vi "Interface.vi"() -> ()   [LabVIEW 2012]
uses:
  MeasureModeControl.ctl
  <vilib>/Utility/miscctls.llb/LVBoundsTypeDef.ctl
  GlobalVariables/LanguagesSettings.vi
  GlobalVariables/CaptParameters.vi
  GlobalVariables/MachineInfos.vi
  GlobalVariables/StabilizationSettings.vi
  GlobalVariables/CalibrationVolumes.vi
  GlobalVariables/HardwarePresent.vi
  GlobalVariables/AppState.vi
  GlobalVariables/PressureAndTimeSamples.vi
  GlobalVariables/CurrentPressure.vi
  GlobalVariables/CommunicationActivity.vi
  GlobalVariables/CalibrationState.vi
  GlobalVariables/FittedCurvePolynom.vi
  <vilib>/Utility/file.llb/Write To Spreadsheet File (string).vi
  <vilib>/Utility/file.llb/Read From Spreadsheet File (string).vi
  GlobalVariables/MeasureExportStrings.vi
  <vilib>/Utility/config.llb/Read Key (String).vi
  GlobalVariables/UserInfos.vi
  <vilib>/Utility/config.llb/NI_LVConfig.lvlib
panel:
  in  "DeleteMeasureLine":bool
  in  "ExportData":bool
  in  "LoadData":bool
  in  "SaveData":bool
  in  "ReloadResultTableTexts":bool
  in  "MeasureMode":T1
  in  "ReloadDiskVolumes":bool
  in  "StabilityAchieved":bool
  in  "UpdateServiceGraph":bool
  in  "ComputeCalibrationResult":bool
  in  "SingleCalibrationMeasureButtonsVisible":bool
  out "FirstGraphSampleIndex":i32
  in  "ServiceButtonsVisible":bool
  in  "ExportMeasuresButtonsVisible":bool
  in  "ChangeMenuState":bool
  in  "MeasureIndicatorsVisible":bool
  in  "MeasureSetupButtonsVisible":bool
  in  "CalibrationButtonsVisible":bool
  in  "CalibrationResultsVisible":bool
  in  "UserFilledDataChanged":bool
  out "NotificationTexts":string[](array[string])
  out "rPressionM":dbl caption="Pression courante" format="%#.1f bars"
  out "error out":errorcluster caption="sortie d'erreur"
  out "indicateurPerteSignal":bool caption="Perte du signal de pression"
  out "indicateurDefautPuissance":bool caption="Défaut de puissance"
  out "indicateurSurpression":bool caption="Surpression"
  in  "btnExit":bool
  out "vTimeDate":timestamp format="%<%.1X\n%x>T"
  out "strInstallName":string="INSTALL NAME"
  in  "AppTab":T2(tab) caption="Onglets1"
  out "presentationPicture":picture caption="Please wait …"
  in  "MeasuresTabs":enum32{"Grain measures", "Pore measures"}(tab) caption="Measures"
  in  "LoadGrainMeasuresBtn":bool
  in  "SaveGrainMeasuresBtn":bool caption="SaveDataFileButton"
  in  "ExportGrainMeasuresBtn":bool caption="Exporter"
  in  "ClearGrainMeasuresBtn":bool caption="Clear measures table"
  out "grainMeasuresTable":string[][](table)=[["Date", "Numéro", "ID de l'échantillon", "Profondeur (coudées)", "Poids à sec (g)", "Volume de grain (cm3)", "Densité de grain (g/cm3)", "Volume de pore (cm3)", "Porosité (%)", "Volume de l'enveloppe (cm3)", "Longueur (cm)", "Diamètre (cm)", "Epaisseur (cm)", "Température (°C)", "Commentaires"]] caption="Résultats Mesures de grains"
  in  "ClearGrainMeasureBtn":bool
  in  "LoadPoreMeasuresBtn":bool
  in  "SavePoreMeasuresBtn":bool caption="SaveDataFileButton"
  in  "ExportPoreMeasuresBtn":bool caption="Exporter"
  out "poreMeasuresTable":string[][](table)=[["Date", "Numéro", "ID de l'échantillon", "Profondeur (coudées)", "Poids à sec (g)", "Volume de grain (cm3)", "Densité de grain (g/cm3)", "Volume de pore (cm3)", "Porosité (%)", "Volume de l'enveloppe (cm3)", "Longueur (cm)", "Diamètre (cm)", "Epaisseur (cm)", "Température (°C)", "Commentaires"]] caption="Résultats"
  in  "ClearPoreMeasuresBtn":bool caption="Clear measures table"
  in  "ClearPoreMeasureBtn":bool
  in  "btnMesureGrain":bool
  out "MeasureTotalAddedVolume":dbl caption="Volume total"
  in  "MeasureDiskSet":i32(listbox) caption="Jeu de disques"
  in  "MeasureDiskVolumes":i32[](listbox) caption="Volumes disponibles"
  in  "Comments":string caption="Commentaires"
  in  "Temperature":dbl caption="Température (°C)"
  in  "BulkVolume":dbl caption="Volume de grain (cm3)"
  in  "DryWeight":dbl caption="Poids à sec (g)"
  in  "SampleDepth":dbl caption="Profondeur (cm)"
  in  "SampleID":string caption="ID de l'échantillon"
  in  "SampleNumber":string caption="Numéro"
  in  "DoMeasureMeasure":bool caption="LaunchMeasureMeasure"
  in  "ReferenceCellMeasure":u16=1 caption="Cellule de référence" min=1 max=2
  in  "DiskSet":i32(listbox) caption="Jeu de disques"
  in  "RestartCalibration":bool
  out "CalibrationStep":u32 caption="Nombre de mesures effectuées"
  in  "CalibrationFilePath":path caption="Fichier de calibration"
  in  "LoadCalibrationFileBtn":bool
  in  "ReferenceCellCalibration":u16=1 caption="Cellule de référence" min=1 max=2
  in  "AvalaibleVolumesList":i32[](listbox) caption="Volumes disponibles"
  in  "ChosenVolume":dbl caption="Volume total"
  in  "DoMeasureCalibration":bool caption="DoCalibrationMeasure"
  in  "EndCalibration":bool caption="Finir la calibration"
  out "Correlation":dbl
  out "AverageAbsoluteDeviation":dbl caption="Deviation moyenne"
  in  "SaveCalibrationFile":bool caption="Save calibration file"
  out "ResidueInd":dbl caption="Résidu"
  out "FittedPolynomCoeffs":dbl[](array[numeric]) caption="Coefficient du polynome d'interpolation"
  in  "ExportToPDF":bool caption="Export to PDF"
  in  "ExportToHTMLBtn":bool
  in  "Client":string
  in  "Country":string caption="Pays"
  in  "Formation":string
  in  "LatitudeLongitude":string caption="Latitude/Longitude"
  in  "Operator":string caption="Opérateur"
  in  "Well":string caption="Puits"
  in  "Lab":string caption="Laboratoire"
  in  "Company":string caption="Entreprise"
  in  "Field":string caption="Champs"
  in  "Location":string caption="Lieu"
  out "PurgeState":string
  in  "FlushPressureGraph":bool
  out "PressureGraph":T3(graph)
  out "NotificationArea":string
  in  "manualModeBtn":bool
  out "vPressionM":dbl format="%#.1f bars"
  in  "btnVidanger":bool
  in  "btnEtal":bool
  in  "btnMesurePore":bool
  in  "MaximalWaitTime":u32 caption="Temps maximal d'attente (ms)"
  in  "VarianceTrigger":dbl caption="Variance minimale"
  in  "MinimalWaitTime":u32 caption="Temps minimal d'attente (ms)"
  in  "PressureCaptorConfig":T4 caption="Configuration du capteur"
  in  "mdpControl":string caption="Mot de passe"
  in  "SamplesMasks":bool[](array[boolean]) caption="Prise en compte point n°"
  out "AverageAbsoluteDeviationServices":dbl caption="Deviation moyenne"
  out "CorrelationServices":dbl caption="Correlation"
  out "ResiduServices":dbl caption="Résidu"
  out "FittedPolynomCoeffsServices":dbl[](array[numeric]) caption="Coefficient du polynome d'interpolation"
  out "XYGraphService":cluster{dbl[], dbl[]}[](graph)=[{[1.0, 2.0, 4.0], [2.0, 1.0, 0.0]}, {[0.5, 1.5, 3.5], [3.0, 4.0, 2.0]}] caption="Mesure et courbe d'étalonnage"
  out "pumeActive":bool caption="PUM-E actif"
  out "pressureCaptorActive":bool caption="Capteur de pression actif"
  in  "MachineName":string caption="Nom de la machine"
  in  "Pressure Gain":dbl=1.0 caption="Gain de pression"
  in  "Pressure Offset":dbl caption="Offset de pression"
  in  "LanguagesList":i32(listbox) caption="Langues disponibles"
  in  "SaveConfigChanges":bool caption="Save changes"
  in  "ValvesConfig":T5 caption="Configuration des valves" {"Mode" items=["RTU", "ASCII"]}
  # "Stabilisation"
  # "Services"
  # "Transmission"
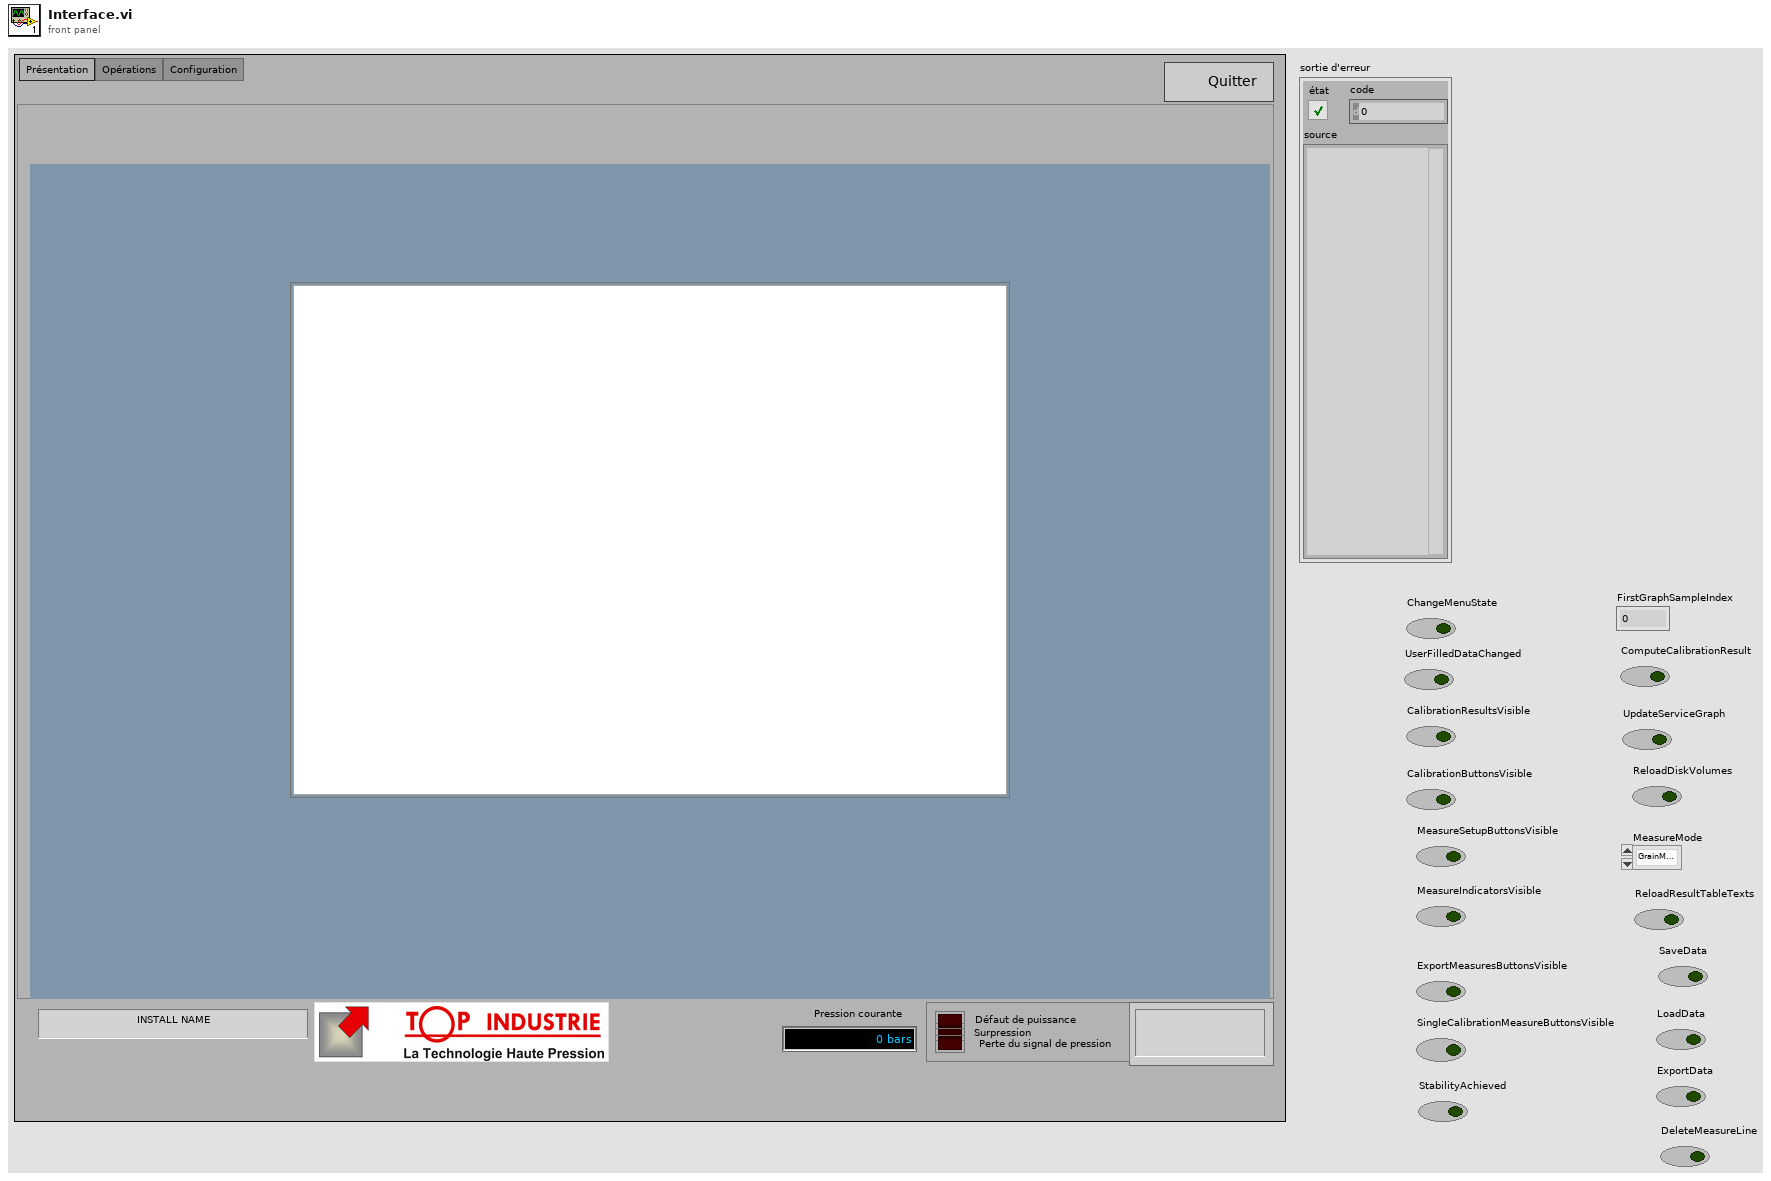
[diagram p1: front panel]
types:
  T1 = typedef "MeasureModeControl.ctl" = enum16{"GrainMeasure", "PoreMeasure"}
  T2 = enum32{"Présentation", "Opérations", "Configuration"}
  T3 = cluster{"TimeSamples":dbl[], "PressureSamples":dbl[]}
  T4 = cluster{"Baudrate":u32, "Port":string, "Databits":u16, "Parity":u16, "Stopbits":u16, "Flow Control":u16, "Slave Address":u16, "Register Address":u16, "Timeout (ms)":u16, "MaxCaptorPressure":dbl}
  T5 = cluster{"Baudrate":u32, "Port":string, "Databits":u16, "Parity":u16, "Stopbits":u16, "Flow Control":u16, "Slave Address":u16, "Mode":u16, "Timeout (ms)":u16}
  T6 = enum8{"Enabled", "Disabled", "Disabled and Grayed Out"}
  T7 = cluster{bool, "CalibrationStep":u32, "Volumes":dbl[], "PressureRatios":dbl[], "Weights":bool[]}
  T8 = typedef "LVBoundsTypeDef.ctl" = cluster{"Width":u32, "Height":u32}
  T9 = cluster{"SupportedLanguagesList":string[], "ActiveLanguage":string, "ActiveLanguageIndex":u16, "LocalisationFileContent[out]":cluster{"Indices":u32[], "LocalizedWords":string[][]}}
  T10 = cluster{"baudrate":u32, "databits":u16, "paritybit":u16, "stopbits":u16, "flux control":u16, "Port":string, "Register Address":u16, "Serial Parameters":cluster{"Mode":enum16{"RTU", "ASCII"}, "Slave Address":u8}, "Timeout":u32, "PressureLimit":dbl}
  T11 = cluster{"SerialNumber":string, "MachineName":string}
  T12 = cluster{"baudrate":u32, "Port":string, "databits":u16, "paritybit":u16, "stopbits":u16, "flux control":u16, "Slave Address":u8, "Register Address":u16, "Timeout":u32, "PressureLimit":dbl}
  T13 = cluster{"CalibrationVolumes":dbl[], "SetName":string}[]
  T14 = cluster{"MinimalWaitTime":u32, "VarianceTrigger":dbl, "MaxWaitTime":u32}
  T15 = typedef "imagedata.ctl" = cluster{"image type":i32, "image depth":i32, "image":u8[], "mask":u8[], "colors":u32[], "Rectangle":cluster{"left":i16, "top":i16, "right":i16, "bottom":i16}}
  T16 = cluster{"Indices":u32[], "LocalizedWords":string[][]}
  T17 = cluster{"SignalLoss":bool, "PumeActive":bool, "CaptorActive":bool}
  T18 = cluster{"CalibrationVolumes":dbl[], "SetName":string}
  T19 = cluster{"SampleNumber":string, "SampleID":string, "SampleDepth":dbl, "DryWeight":dbl, "BulkVolume":dbl, "Temperature":dbl, "Comments":string}
  T20 = cluster{"date":string, "sampleNumber":string, "sampleID":string, "sampleDepth":dbl, "dryWeight":dbl, "grainDensity":dbl, "bulk volume":dbl, "poreVolume":dbl, "porosity":dbl, "sleeveVolume":dbl, "sleeveLength":dbl, "sleeveDiameter":dbl, "sleeveThickness":dbl, "temperature":dbl, "comments":string}
  T21 = cluster{"NewVal":u32, "VarianceTrigger":dbl, "MaxWaitTime":u32}
  T22 = cluster{"MinimalWaitTime":u32, "NewVal":dbl, "MaxWaitTime":u32}
  T23 = cluster{"MinimalWaitTime":u32, "VarianceTrigger":dbl, "NewVal":u32}
  T24 = cluster{"Baudrate":u32, "Databits":u16, "Parity":u16, "Stopbits":u16, "Flow Control":u16, "Port":string, "Register Address":u16, cluster{u16, "Slave Address":u16}, "Timeout (ms)":u16, "MaxCaptorPressure":dbl}
  T25 = cluster{"SupportedLanguagesList":string[], "String":string, "LanguagesList":i32, "LocalisationFileContent[out]":cluster{"Indices":u32[], "LocalizedWords":string[][]}}
  T26 = typedef "NI_LVConfig.lvlib/Config Data RefNum.ctl" = refnum<k1>
  T27 = typedef "LVRowAndColumnTypeDef.ctl" = cluster{"Row":i32, "Column":i32}
  T28 = cluster{"location":string, "Field":string, "Company":string, "Lab":string, "Operator":string, "Well":string, "Lat/Long":string, "Formation":string, "Country":string, "Client":string}
  T29 = cluster{"NewVal":string, "Field":string, "Company":string, "Lab":string, "Operator":string, "Well":string, "Lat/Long":string, "Formation":string, "Country":string, "Client":string}
  T30 = cluster{"location":string, "NewVal":string, "Company":string, "Lab":string, "Operator":string, "Well":string, "Lat/Long":string, "Formation":string, "Country":string, "Client":string}
  T31 = cluster{"location":string, "Field":string, "NewVal":string, "Lab":string, "Operator":string, "Well":string, "Lat/Long":string, "Formation":string, "Country":string, "Client":string}
  T32 = cluster{"location":string, "Field":string, "Company":string, "NewVal":string, "Operator":string, "Well":string, "Lat/Long":string, "Formation":string, "Country":string, "Client":string}
  T33 = cluster{"location":string, "Field":string, "Company":string, "Lab":string, "NewVal":string, "Well":string, "Lat/Long":string, "Formation":string, "Country":string, "Client":string}
  T34 = cluster{"location":string, "Field":string, "Company":string, "Lab":string, "Operator":string, "NewVal":string, "Lat/Long":string, "Formation":string, "Country":string, "Client":string}
  T35 = cluster{"location":string, "Field":string, "Company":string, "Lab":string, "Operator":string, "Well":string, "NewVal":string, "Formation":string, "Country":string, "Client":string}
  T36 = cluster{"location":string, "Field":string, "Company":string, "Lab":string, "Operator":string, "Well":string, "Lat/Long":string, "NewVal":string, "Country":string, "Client":string}
  T37 = cluster{"location":string, "Field":string, "Company":string, "Lab":string, "Operator":string, "Well":string, "Lat/Long":string, "Formation":string, "NewVal":string, "Client":string}
  T38 = cluster{"location":string, "Field":string, "Company":string, "Lab":string, "Operator":string, "Well":string, "Lat/Long":string, "Formation":string, "Country":string, "NewVal":string}
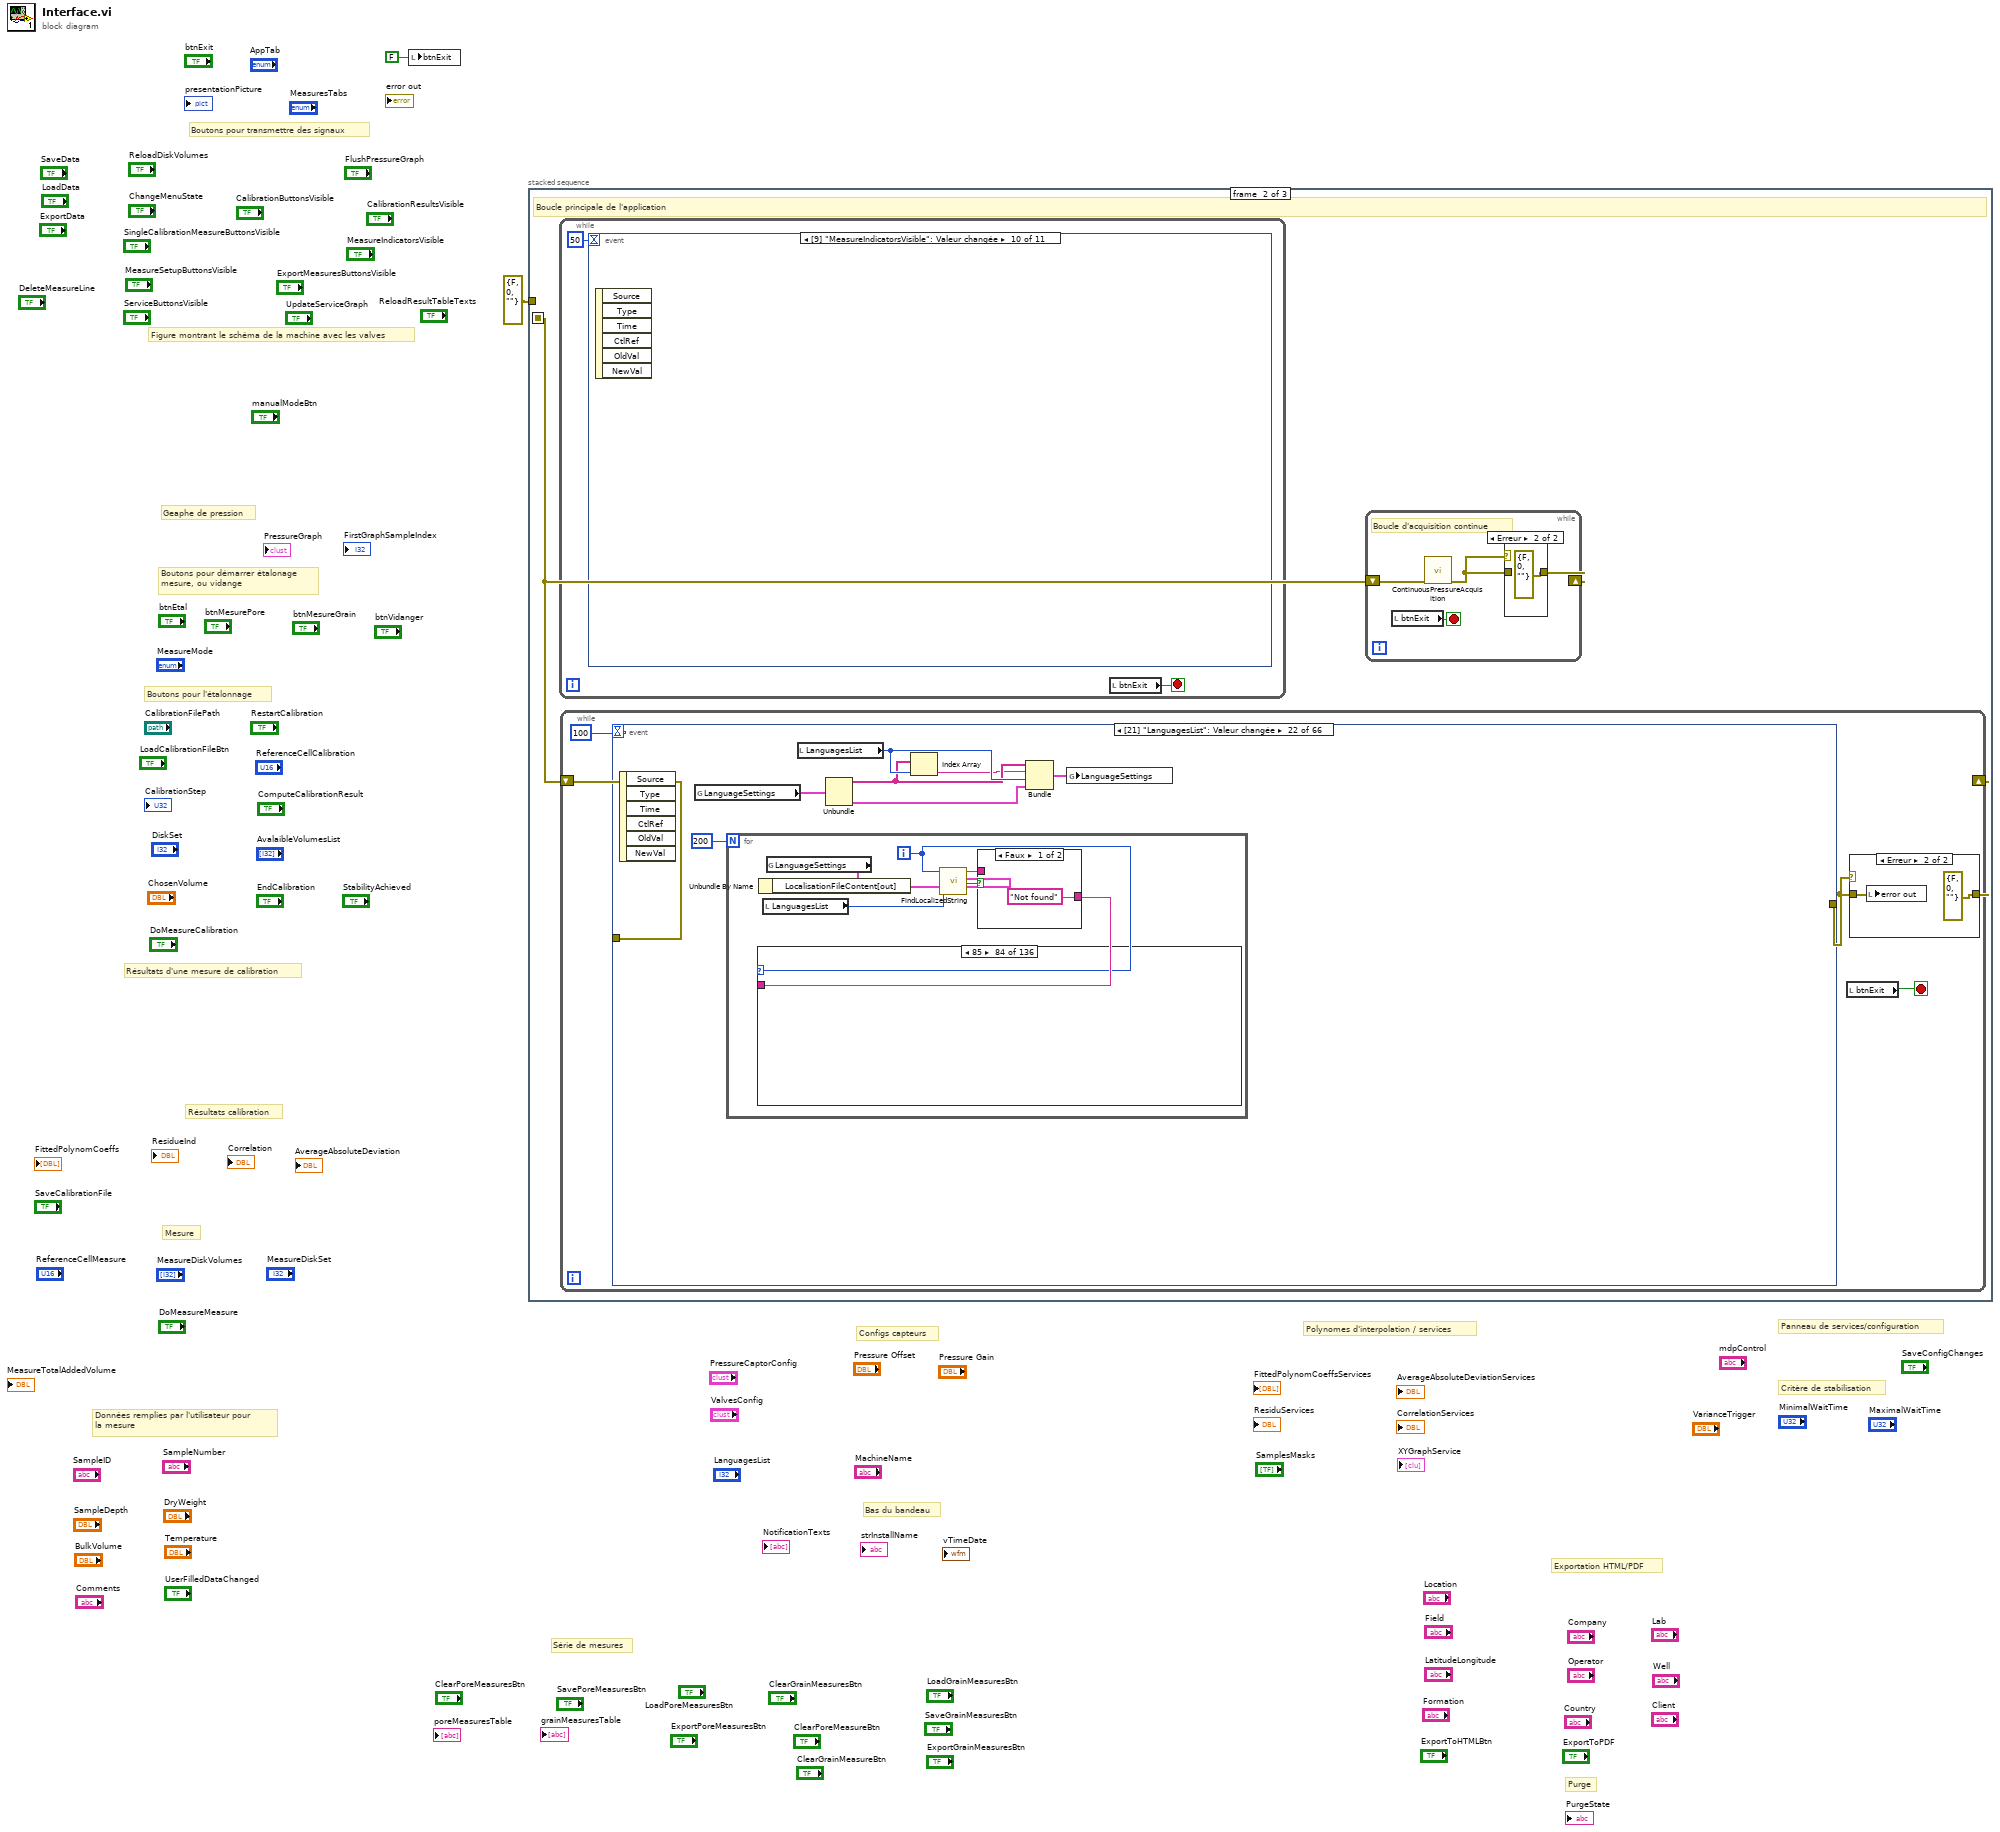
[diagram p0: block diagram]
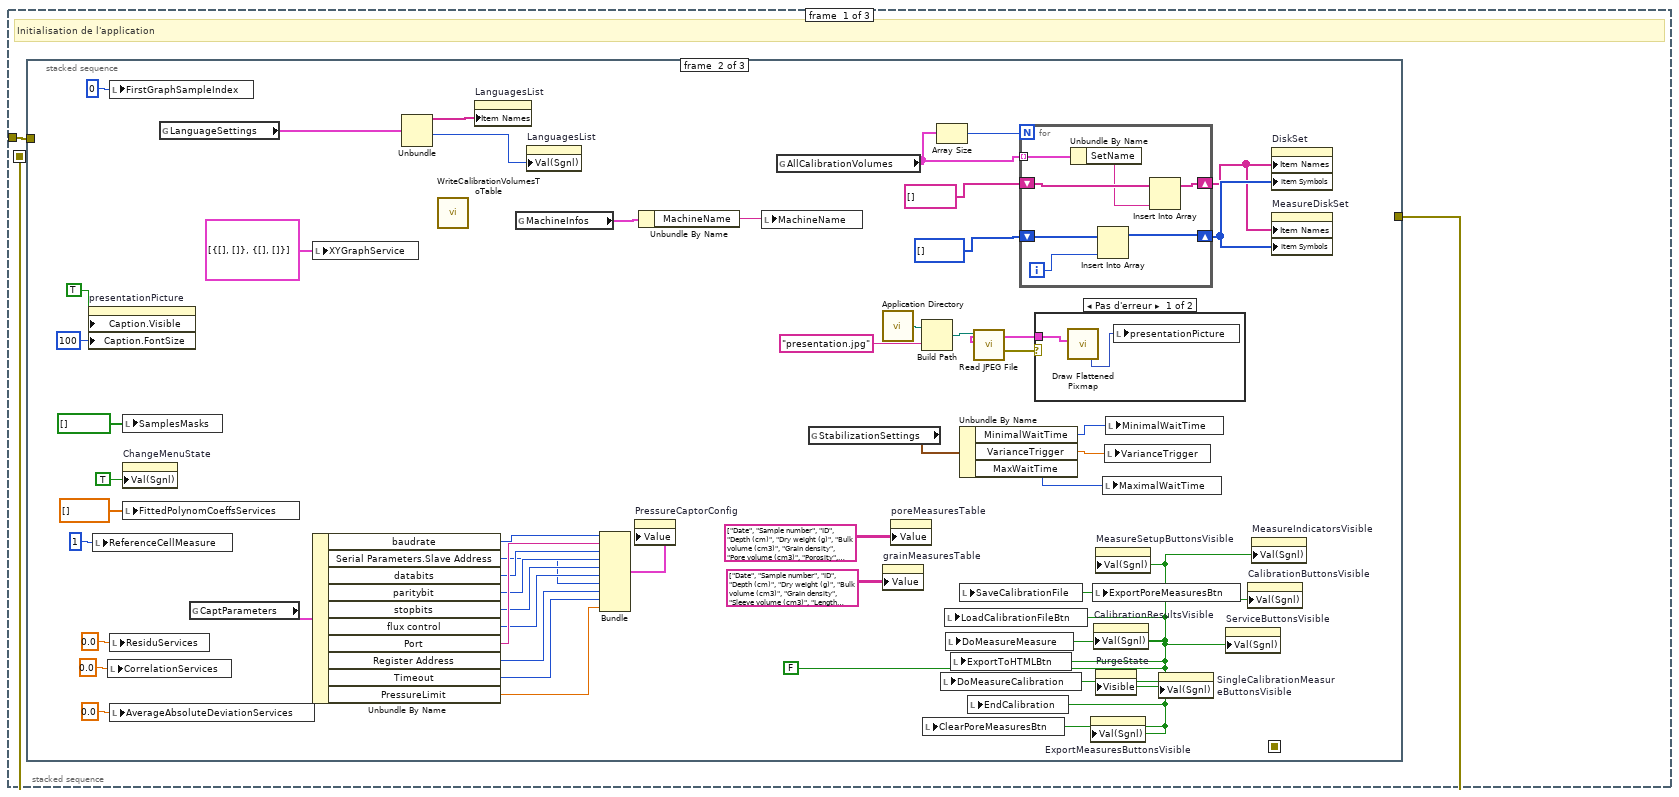
[diagram p2: hidden frame]
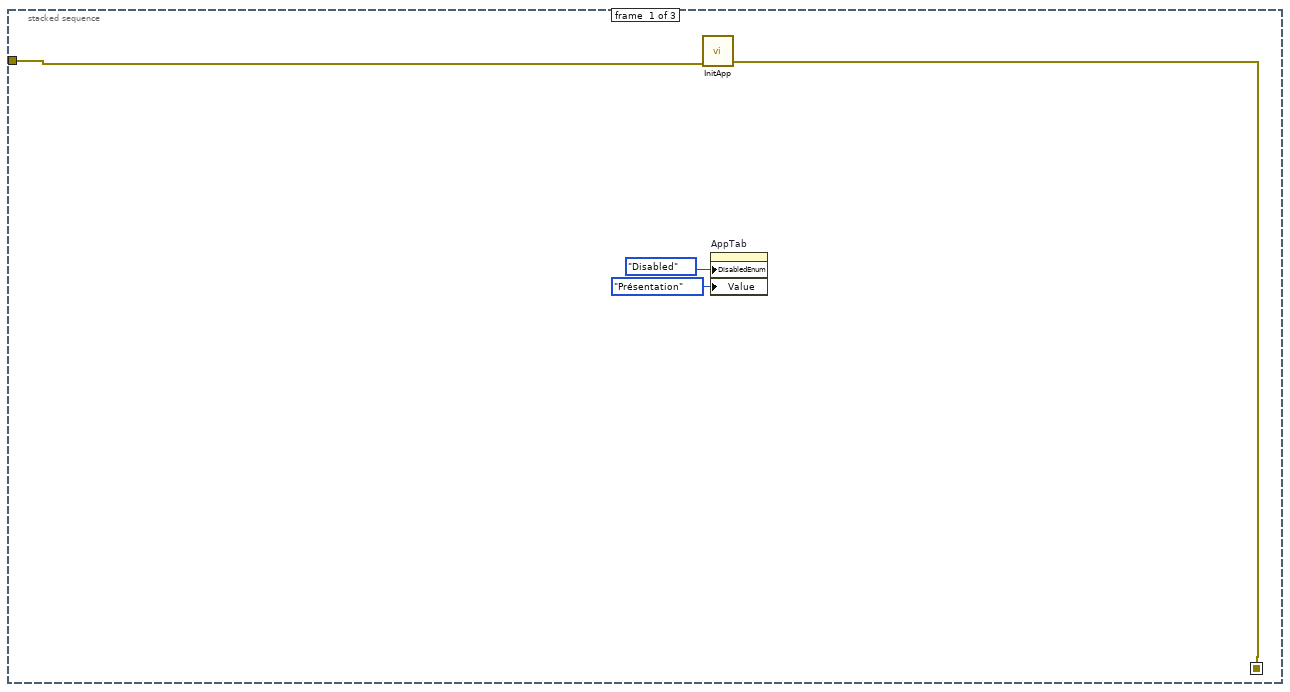
[diagram p3: hidden frame]
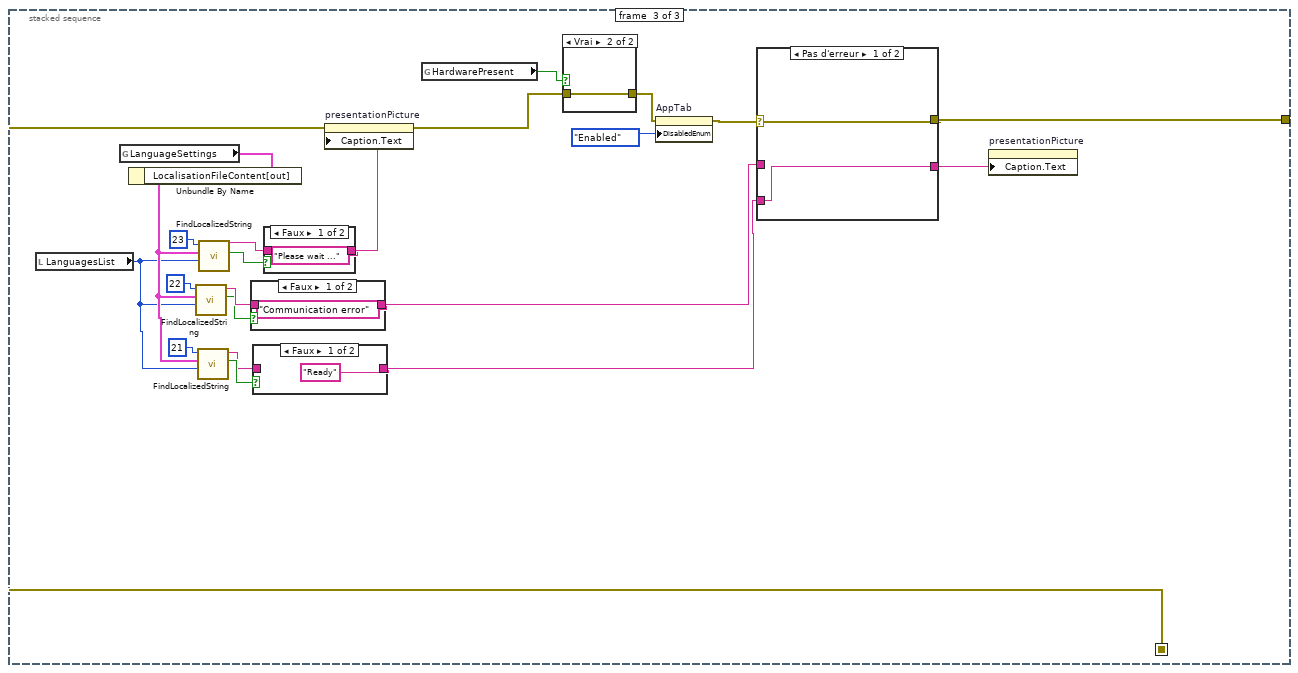
[diagram p5: hidden frame]
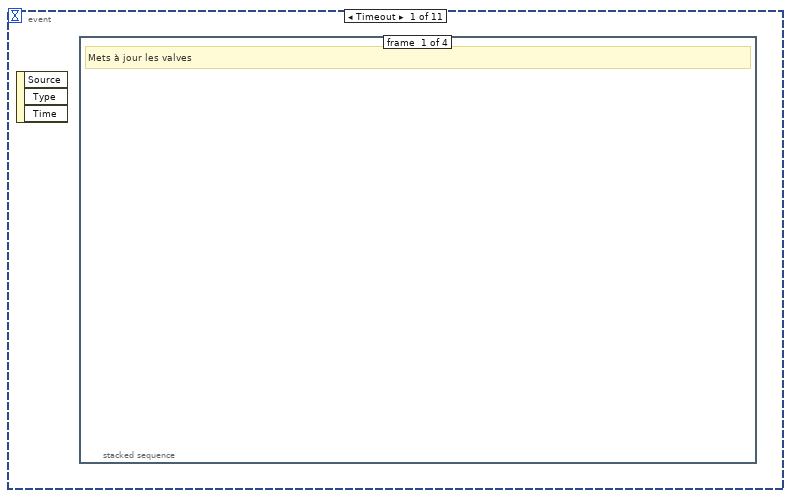
[diagram p12: hidden frame]
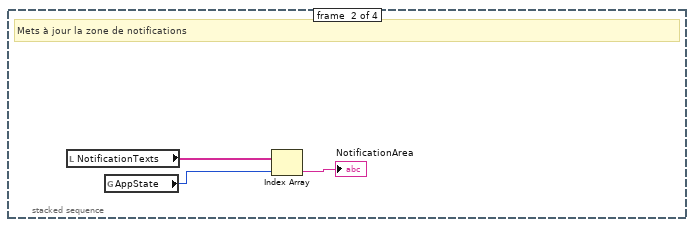
[diagram p13: hidden frame]
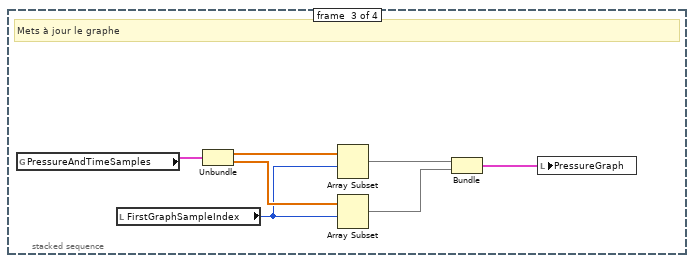
[diagram p14: hidden frame]
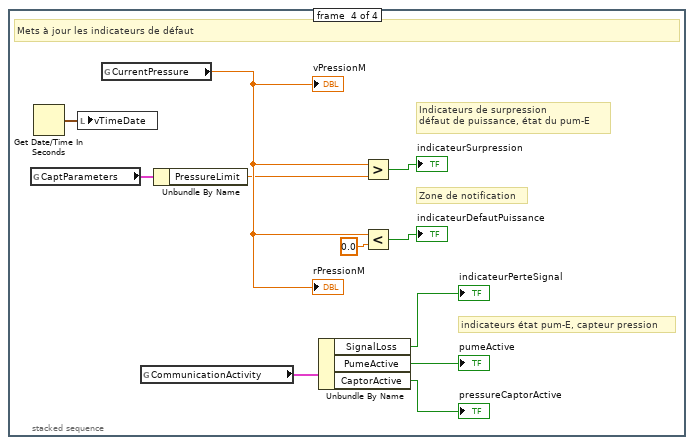
[diagram p15: hidden frame]
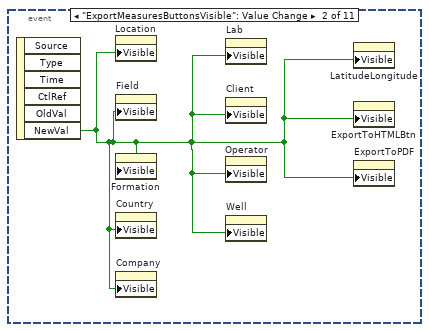
[diagram p16: hidden frame]
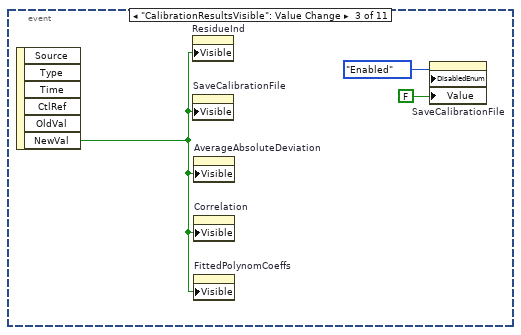
[diagram p17: hidden frame]
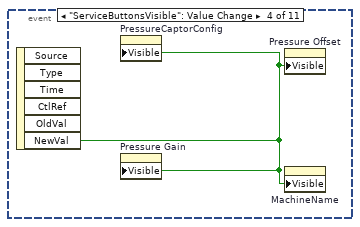
[diagram p18: hidden frame]
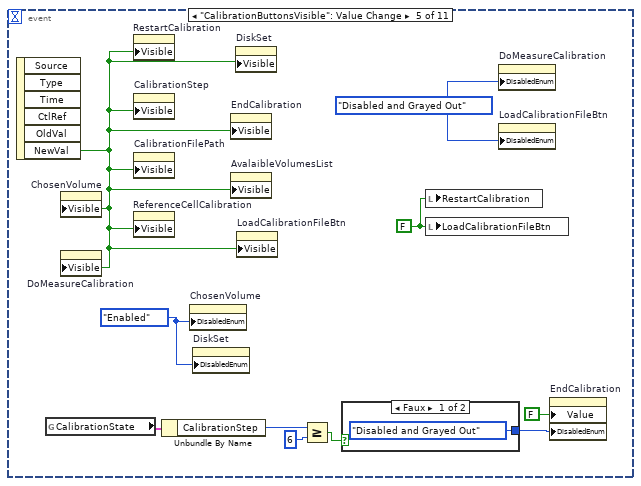
[diagram p19: hidden frame]
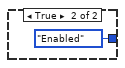
[diagram p20: hidden frame]
diagram:
  # "Boutons pour transmettre des signaux"
  # "Configs capteurs"
  # "Polynomes d'interpolation / services"
  # "Critère de stabilisation"
  # "Résultats d'une mesure de calibration"
  # "Geaphe de pression"
  # "Figure montrant le schéma de la machine avec les valves"
  # "Exportation HTML/PDF"
  # "Série de mesures"
  # "Données remplies par l'utilisateur pour \nla mesure"
  # "Panneau de services/configuration"
  # "Mesure"
  # "Résultats calibration"
  # "Purge"
  # "Boutons pour démarrer étalonage\nmesure, ou vidange"
  # "Bas du bandeau"
  # "Boutons pour l'étalonnage"
  n1 = local write "btnExit"(FALSE ("btnExit")) -> ()
  n2 = stacked-sequence {
    seq-local: [w3 _ _] -> [_ w99 _]
    tunnel: errorcluster {"status"=FALSE, "code"=0, "source"=""} ("error in") -> [w4 _ _]
    frame #0 {
      # "Initialisation de l'application"
      n3 = stacked-sequence {
        seq-local: [w5 _ _] -> [_ _ w64]
        tunnel: w4 -> [w8 _ _]
        tunnel: [_ _ w65] -> w3
        frame #0 {
          n4 = call "InitApp.vi"("error in"=w8) -> ("error out"=w5:errorcluster)  [unwired: 10 in]
          n5 = property on="AppTab" class="Onglet (strict)"("DisabledEnum"=T6."Disabled" ("Disabled"), "Value"=T2."Présentation" ("Onglets1")) -> ()  [unwired: 2 in, 2 out]
        }
        frame #1 {
          w30 = FALSE ("Visible")
          n6 = property on="presentationPicture" class="Image"("Caption.Visible"=TRUE, "Caption.FontSize"=100) -> ()  [unwired: 2 in, 2 out]
          n7 = local write "ReferenceCellMeasure"(u16 1 ("ReferenceCellMeasure")) -> ()
          n8 = local write "CorrelationServices"(0.0 ("CorrelationServices")) -> ()
          n9 = local write "FirstGraphSampleIndex"(u32 0 ("FirstGraphSampleIndex")) -> ()
          n10 = local write "ResiduServices"(0.0 ("ResiduServices")) -> ()
          n11 = local write "AverageAbsoluteDeviationServices"(0.0 ("AverageAbsoluteDeviationServices")) -> ()
          n12 = local write "SamplesMasks"(bool[] [] ("SamplesMasks")) -> ()
          n13 = property on="ChangeMenuState" class="Bool (strict)"("Val(Sgnl)"=TRUE ("Value (Signaling)")) -> ()  [unwired: 2 in, 2 out]
          n14 = local write "FittedPolynomCoeffsServices"(dbl[] [] ("FittedPolynomCoeffsServices")) -> ()
          n15 = global read "LanguagesSettings.vi" "LanguageSettings"() -> (w53:T9)
          n16 = global read "CaptParameters.vi" "CaptParameters"() -> (w50:T10)
          n17 = local write "XYGraphService"(cluster{dbl[], dbl[]}[] [{[], []}, {[], []}] ("XYGraphService")) -> ()
          n18 = Unbundle By Name(w50) -> ("baudrate"=w49:u32, "Serial Parameters.Slave Address"=w43:u8, "databits"=w47:u16, "paritybit"=w46:u16, "stopbits"=w45:u16, "flux control"=w44:u16, "Port"=w48:string, "Register Address"=w42:u16, "Timeout"=w41:u32, "PressureLimit"=w23:dbl)
          n19 = Unbundle(w53) -> ("SupportedLanguagesList"=w52:string[], "ActiveLanguageIndex"=w51:u16)  [unwired: 2 out]
          n20 = call "WriteCalibrationVolumesToTable.vi"() -> ()  [unwired: 12 in]
          n21 = property on="LanguagesList" class="LstDér (strict)"("Item Names"=w52) -> ()  [unwired: 2 in, 2 out]
          n22 = global read "MachineInfos.vi" "MachineInfos"() -> (w22:T11)
          n23 = property on="LanguagesList" class="LstDér (strict)"("Val(Sgnl)"=w51) -> ()  [unwired: 2 in, 2 out]
          n24 = Bundle("baudrate"=w49, "Port"=w48, "databits"=w47, "paritybit"=w46, "stopbits"=w45, "flux control"=w44, "Slave Address"=w43, "Register Address"=w42, "Timeout"=w41, "PressureLimit"=w23) -> (w40:T12)  [unwired: 1 in]
          n25 = property on="PressureCaptorConfig" class="Clust (strict)"("Value"=w40) -> ()  [unwired: 2 in, 2 out]
          n26 = Unbundle By Name(w22) -> ("MachineName"=w21:string)
          n27 = local write "MachineName"(w21) -> ()
          n28 = global read "CalibrationVolumes.vi" "AllCalibrationVolumes"() -> (w14:T13)
          n29 = global read "StabilizationSettings.vi" "StabilizationSettings"() -> (w20:T14)
          n30 = call <vilib>:"Application Directory.vi"() -> ("Application Directory"=w39:path)
          n31 = property on="grainMeasuresTable" class="Tbl (strict)"("Value"=string[][] [["Date", "Sample number", "ID", "Depth (cm)", "Dry weight (g)", "Bulk volume (cm3)", "Grain density", "Sleeve volume (cm3)", "Length (cm)", "Diameter (cm)", "Thickness (cm)", "Temperature (°C)", "Comments"]] ("measuresTable")) -> ()  [unwired: 2 in, 2 out]
          n32 = property on="poreMeasuresTable" class="Tbl (strict)"("Value"=string[][] [["Date", "Sample number", "ID", "Depth (cm)", "Dry weight (g)", "Bulk volume (cm3)", "Grain density", "Pore volume (cm3)", "Porosity", "Sleeve volume (cm3)", "Length (cm)", "Diameter (cm)", "Thickness (cm)", "Temperature (°C)", "Comments"]] ("measuresTable")) -> ()  [unwired: 2 in, 2 out]
          n33 = Build Path(base path=w39, name or relative path="presentation.jpg") -> (appended path=w38:path)
          n34 = local write "ClearPoreMeasuresBtn"(w30) -> ()
          n35 = Array Size(array=w14) -> (size(s)=w15:i32)
          n36 = local write "DoMeasureCalibration"(w30) -> ()
          n37 = local write "LoadCalibrationFileBtn"(w30) -> ()
          n38 = local write "DoMeasureMeasure"(w30) -> ()
          n39 = local write "ExportToHTMLBtn"(w30) -> ()
          n40 = Unbundle By Name(w20) -> ("MinimalWaitTime"=w19:u32, "VarianceTrigger"=w18:dbl, "MaxWaitTime"=w17:u32)
          n41 = local write "SaveCalibrationFile"(w30) -> ()
          n42 = local write "EndCalibration"(w30) -> ()
          n43 = call <vilib>:"Read JPEG File.vi"("path to JPEG file"=w38) -> ("error out"=w36:errorcluster, "image data"=w37:T15)  [unwired: 8 in, 1 out]
          n44 = for {
            N: w15 -> [_]
            shift-right: [w60] -> w11
            shift-left: string[] [] -> [w61]
            tunnel: w14 -> [w59] mode=indexing
            shift-right: [w55] -> w12
            shift-left: i32[] [] -> [w57]
            i -> [w56]
            n45 = Unbundle By Name(w59) -> ("SetName"=w58:string)
            n46 = Insert Into Array(array=w57, new element=w56) -> (w55:i32[])  [unwired: 1 in]
            n47 = Insert Into Array(array=w61, new element=w58) -> (w60:string[])  [unwired: 1 in]
          }
          n48 = case shown="Pas d'erreur" w36 {
            tunnel: w37 -> [w63 _]
            frame No Error {
              n49 = call <vilib>:"Draw Flattened Pixmap.vi"("image data"=w63) -> ("new picture"=w62:picture)  [unwired: 8 in]
              n50 = local write "presentationPicture"(w62) -> ()
            }
            frame Error {
            }
          }
          n51 = property on="ExportMeasuresButtonsVisible" class="Bool (strict)"("Val(Sgnl)"=w30) -> ()  [unwired: 2 in, 2 out]
          n52 = local write "ExportPoreMeasuresBtn"(w30) -> ()
          n53 = property on="CalibrationResultsVisible" class="Bool (strict)"("Val(Sgnl)"=w30) -> ()  [unwired: 2 in, 2 out]
          n54 = property on="MeasureSetupButtonsVisible" class="Bool (strict)"("Val(Sgnl)"=w30) -> ()  [unwired: 2 in, 2 out]
          n55 = property on="PurgeState" class="Ch"("Visible"=w30) -> ()  [unwired: 2 in, 2 out]
          n56 = local write "MaximalWaitTime"(w17) -> ()
          n57 = local write "VarianceTrigger"(w18) -> ()
          n58 = local write "MinimalWaitTime"(w19) -> ()
          n59 = property on="SingleCalibrationMeasureButtonsVisible" class="Bool (strict)"("Val(Sgnl)"=w30) -> ()  [unwired: 2 in, 2 out]
          n60 = property on="ServiceButtonsVisible" class="Bool (strict)"("Val(Sgnl)"=w30) -> ()  [unwired: 2 in, 2 out]
          n61 = property on="CalibrationButtonsVisible" class="Bool (strict)"("Val(Sgnl)"=w30) -> ()  [unwired: 2 in, 2 out]
          n62 = property on="MeasureIndicatorsVisible" class="Bool (strict)"("Val(Sgnl)"=w30) -> ()  [unwired: 2 in, 2 out]
          n63 = property on="DiskSet" class="LstDér (strict)"("Item Names"=w11, "Item Symbols"=w12) -> ()  [unwired: 2 in, 2 out]
          n64 = property on="MeasureDiskSet" class="LstDér (strict)"("Item Names"=w11, "Item Symbols"=w12) -> ()  [unwired: 2 in, 2 out]
        }
        frame #2 {
          n65 = local read "LanguagesList"() -> (w83:i32)
          n66 = global read "LanguagesSettings.vi" "LanguageSettings"() -> (w69:T9)
          n67 = Unbundle By Name(w69) -> ("LocalisationFileContent[out]"=w84:T16)
          n68 = call "FindLocalizedString.vi"("LangIndex"=w83, "LocalizationFileContent"=w84, "WordIndex"=22) -> ("Found"=w73:bool, "LocalizedString"=w74:string)  [unwired: 7 in]
          n69 = call "FindLocalizedString.vi"("LangIndex"=w83, "LocalizationFileContent"=w84, "WordIndex"=21) -> ("Found"=w81:bool, "LocalizedString"=w80:string)  [unwired: 7 in]
          n70 = call "FindLocalizedString.vi"("LangIndex"=w83, "LocalizationFileContent"=w84, "WordIndex"=23) -> ("Found"=w76:bool, "LocalizedString"=w77:string)  [unwired: 7 in]
          n71 = case shown="Faux" w73 {
            tunnel: w74 -> [_ w94]
            tunnel: ["Communication error" w94] -> w75
            frame False {
            }
            frame True {
            }
          }
          n72 = case shown="Faux" w81 {
            tunnel: w80 -> [_ w88]
            tunnel: ["Ready" w88] -> w85
            frame False {
            }
            frame True {
            }
          }
          n73 = case shown="Faux" w76 {
            tunnel: w77 -> [_ w92]
            tunnel: ["Please wait ..." w92] -> w78
            frame False {
            }
            frame True {
            }
          }
          n74 = property on="presentationPicture" class="Image"(error in=w64, "Caption.Text"=w78) -> (error out=w72:errorcluster)  [unwired: 1 in, 1 out]
          n75 = global read "HardwarePresent.vi" "HardwarePresent"() -> (w86:bool)
          n76 = case shown="Vrai" w86 {
            tunnel: [w89 w90] -> w68
            tunnel: w72 -> [w89 w90]
            frame False {
            }
            frame True {
            }
          }
          n77 = property on="AppTab" class="Onglet (strict)"(error in=w68, "DisabledEnum"=T6."Enabled" ("Disabled")) -> (error out=w67:errorcluster)  [unwired: 1 in, 1 out]
          n78 = case shown="Pas d'erreur" w67 {
            selector: w67 -> [w96 w98]
            tunnel: [w96 w98] -> w65
            tunnel: w75 -> [_ w97]
            tunnel: [w95 w97] -> w79
            tunnel: w85 -> [w95 _]
            frame No Error {
            }
            frame Error {
            }
          }
          n79 = property on="presentationPicture" class="Image"("Caption.Text"=w79) -> ()  [unwired: 2 in, 2 out]
        }
      }
    }
    frame #1 {
      # "Boucle principale de l'application"
      n80 = while {
        stop <- w106 stop-if-true
        n81 = event shown="[9] \"MeasureIndicatorsVisible\": Valeur changée" {
          selector: _ -> [_ _ _ _ _ _ _ _ _ _ _]
          dyn-events: _ -> [_ _ _ _ _ _ _ _ _ _ _]
          timeout: 50 -> [_ _ _ _ _ _ _ _ _ _ _]
          event Timeout {
            n82 = event-data() -> ()  [unwired: 1 in, 3 out]
            n83 = stacked-sequence {
              frame #0 {
                # "Mets à jour les valves"
              }
              frame #1 {
                # "Mets à jour la zone de notifications"
                n84 = local read "NotificationTexts"() -> (w108:string[])
                n85 = global read "AppState.vi" "AppState"() -> (w110:u16)
                n86 = Index Array(array=w108, index=w110) -> (element=→"NotificationArea":string)
              }
              frame #2 {
                # "Mets à jour le graphe"
                n87 = global read "PressureAndTimeSamples.vi" "PressureAndTimeSamples"() -> (w117:T3)
                n88 = local read "FirstGraphSampleIndex"() -> (w113:i32)
                n89 = Unbundle(w117) -> ("TimeSamples"=w115:dbl[], "PressureSamples"=w114:dbl[])
                n90 = Array Subset(array=w115, index=w113) -> (w112:dbl[])  [unwired: 1 in]
                n91 = Array Subset(array=w114, index=w113) -> (w111:dbl[])  [unwired: 1 in]
                n92 = Bundle(w112, w111) -> (w116:cluster{dbl[], dbl[]})  [unwired: 1 in]
                n93 = local write "PressureGraph"(w116) -> ()
              }
              frame #3 {
                # "indicateurs état pum-E, capteur pression"
                # "Indicateurs de surpression\ndéfaut de puissance, état du pum-E"
                # "Zone de notification"
                # "Mets à jour les indicateurs de défaut"
                n94 = global read "CaptParameters.vi" "CaptParameters"() -> (w120:T10)
                n95 = Get Date/Time In Seconds() -> (seconds since 1Jan1904=w118:timestamp)
                n96 = local write "vTimeDate"(w118) -> ()
                n97 = global read "CurrentPressure.vi" "CurrentPressure"() -> (w121:dbl)
                "vPressionM" <- w121
                "rPressionM" <- w121
                n98 = global read "CommunicationActivity.vi" "CommunicationActivity"() -> (w128:T17)
                n99 = Unbundle By Name(w120) -> ("PressureLimit"=w119:dbl)
                n100 = Unbundle By Name(w128) -> ("SignalLoss"=→"indicateurPerteSignal":bool, "PumeActive"=→"pumeActive":bool, "CaptorActive"=→"pressureCaptorActive":bool)
                n101 = Greater?(x=w121, y=w119) -> (0:→"indicateurSurpression":bool)
                n102 = Less?(x=w121, y=0.0) -> (x < y?=→"indicateurDefautPuissance":bool)
              }
            }
          }
          event "ExportMeasuresButtonsVisible": Value Change {
            n103 = event-data() -> ("NewVal"=w129:bool)  [unwired: 1 in, 5 out]
            n104 = property on="Location" class="Ch"("Visible"=w129) -> ()  [unwired: 2 in, 2 out]
            n105 = property on="Field" class="Ch"("Visible"=w129) -> ()  [unwired: 2 in, 2 out]
            n106 = property on="Formation" class="Ch"("Visible"=w129) -> ()  [unwired: 2 in, 2 out]
            n107 = property on="Country" class="Ch"("Visible"=w129) -> ()  [unwired: 2 in, 2 out]
            n108 = property on="Company" class="Ch"("Visible"=w129) -> ()  [unwired: 2 in, 2 out]
            n109 = property on="Lab" class="Ch"("Visible"=w129) -> ()  [unwired: 2 in, 2 out]
            n110 = property on="Client" class="Ch"("Visible"=w129) -> ()  [unwired: 2 in, 2 out]
            n111 = property on="Operator" class="Ch"("Visible"=w129) -> ()  [unwired: 2 in, 2 out]
            n112 = property on="Well" class="Ch"("Visible"=w129) -> ()  [unwired: 2 in, 2 out]
            n113 = property on="LatitudeLongitude" class="Ch"("Visible"=w129) -> ()  [unwired: 2 in, 2 out]
            n114 = property on="ExportToHTMLBtn" class="Bool (strict)"("Visible"=w129) -> ()  [unwired: 2 in, 2 out]
            n115 = property on="ExportToPDF" class="Bool (strict)"("Visible"=w129) -> ()  [unwired: 2 in, 2 out]
          }
          event "CalibrationResultsVisible": Value Change {
            n116 = event-data() -> ("NewVal"=w131:bool)  [unwired: 1 in, 5 out]
            n117 = property on="ResidueInd" class="NumNb (strict)"("Visible"=w131) -> ()  [unwired: 2 in, 2 out]
            n118 = property on="SaveCalibrationFile" class="Bool (strict)"("Visible"=w131) -> ()  [unwired: 2 in, 2 out]
            n119 = property on="AverageAbsoluteDeviation" class="NumNb (strict)"("Visible"=w131) -> ()  [unwired: 2 in, 2 out]
            n120 = property on="Correlation" class="NumNb (strict)"("Visible"=w131) -> ()  [unwired: 2 in, 2 out]
            n121 = property on="FittedPolynomCoeffs" class="Tabl (strict)"("Visible"=w131) -> ()  [unwired: 2 in, 2 out]
            n122 = property on="SaveCalibrationFile" class="Bool (strict)"("DisabledEnum"=T6."Enabled" ("Disabled"), "Value"=FALSE ("SaveCalibrationFile")) -> ()  [unwired: 2 in, 2 out]
          }
          event "ServiceButtonsVisible": Value Change {
            n123 = event-data() -> ("NewVal"=w133:bool)  [unwired: 1 in, 5 out]
            n124 = property on="PressureCaptorConfig" class="Clust (strict)"("Visible"=w133) -> ()  [unwired: 2 in, 2 out]
            n125 = property on="Pressure Gain" class="NumNb (strict)"("Visible"=w133) -> ()  [unwired: 2 in, 2 out]
            n126 = property on="Pressure Offset" class="NumNb (strict)"("Visible"=w133) -> ()  [unwired: 2 in, 2 out]
            n127 = property on="MachineName" class="Ch"("Visible"=w133) -> ()  [unwired: 2 in, 2 out]
          }
          event "CalibrationButtonsVisible": Value Change {
            w136 = FALSE ("RestartCalibration")
            w135 = T6."Enabled" ("Disabled")
            w143 = T6."Disabled and Grayed Out" ("Disabled")
            n128 = event-data() -> ("NewVal"=w134:bool)  [unwired: 1 in, 5 out]
            n129 = global read "CalibrationState.vi" "CalibrationState"() -> (w137:T7)
            n130 = property on="ChosenVolume" class="NumNb (strict)"("Visible"=w134) -> ()  [unwired: 2 in, 2 out]
            n131 = property on="DoMeasureCalibration" class="Bool (strict)"("Visible"=w134) -> ()  [unwired: 2 in, 2 out]
            n132 = property on="RestartCalibration" class="Bool (strict)"("Visible"=w134) -> ()  [unwired: 2 in, 2 out]
            n133 = property on="CalibrationStep" class="NumNb (strict)"("Visible"=w134) -> ()  [unwired: 2 in, 2 out]
            n134 = property on="CalibrationFilePath" class="Chm"("Visible"=w134) -> ()  [unwired: 2 in, 2 out]
            n135 = property on="ReferenceCellCalibration" class="NumNb (strict)"("Visible"=w134) -> ()  [unwired: 2 in, 2 out]
            n136 = Unbundle By Name(w137) -> ("CalibrationStep"=w138:u32)
            n137 = property on="ChosenVolume" class="NumNb (strict)"("DisabledEnum"=w135) -> ()  [unwired: 2 in, 2 out]
            n138 = property on="DiskSet" class="LstDér (strict)"("DisabledEnum"=w135) -> ()  [unwired: 2 in, 2 out]
            n139 = property on="EndCalibration" class="Bool (strict)"("Visible"=w134) -> ()  [unwired: 2 in, 2 out]
            n140 = property on="AvalaibleVolumesList" class="LstDér (strict)"("Visible"=w134) -> ()  [unwired: 2 in, 2 out]
            n141 = property on="DiskSet" class="LstDér (strict)"("Visible"=w134) -> ()  [unwired: 2 in, 2 out]
            n142 = property on="LoadCalibrationFileBtn" class="Bool (strict)"("Visible"=w134) -> ()  [unwired: 2 in, 2 out]
            n143 = Greater Or Equal?(x=w138, y=u32 6) -> (x >= y?=w140:bool)
            n144 = case shown="Faux" w140 {
              tunnel: [T6."Disabled and Grayed Out" ("Disabled") T6."Enabled" ("Disabled")] -> w141
              frame False {
              }
              frame True {
              }
            }
            n145 = local write "RestartCalibration"(w136) -> ()
            n146 = local write "LoadCalibrationFileBtn"(w136) -> ()
            n147 = property on="DoMeasureCalibration" class="Bool (strict)"("DisabledEnum"=w143) -> ()  [unwired: 2 in, 2 out]
            n148 = property on="LoadCalibrationFileBtn" class="Bool (strict)"("DisabledEnum"=w143) -> ()  [unwired: 2 in, 2 out]
            n149 = property on="EndCalibration" class="Bool (strict)"("Value"=FALSE ("EndCalibration"), "DisabledEnum"=w141) -> ()  [unwired: 2 in, 2 out]
          }
          event "SingleCalibrationMeasureButtonsVisible": Value Change {
            n150 = event-data() -> ()  [unwired: 1 in, 6 out]
          }
          event "ChangeMenuState": Value Change {
            n151 = event-data() -> ()  [unwired: 1 in, 6 out]
            n152 = global read "AppState.vi" "AppState"() -> (w152:u16)
            n153 = global read "CalibrationState.vi" "CalibrationState"() -> (w148:T7)
            n154 = global read "AppState.vi" "AppState"() -> (w170:u16)
            n155 = global read "CalibrationState.vi" "CalibrationState"() -> (w176:T7)
            n156 = global read "AppState.vi" "AppState"() -> (w165:u16)
            n157 = global read "AppState.vi" "AppState"() -> (w160:u16)
            n158 = Not Equal?(x=w152, y=u16 1) -> (x != y?=w154:bool)
            n159 = Not Equal?(x=w152, y=u16 3) -> (x != y?=w155:bool)
            n160 = Unbundle(w148) -> (w150:bool)  [unwired: 4 out]
            n161 = And(x=w154, y=w155) -> (x .and. y?=w146:bool)
            n162 = Not Equal?(x=w170, y=u16 3) -> (x != y?=w171:bool)
            n163 = And(x=w150, y=w146) -> (x .and. y?=w149:bool)
            n164 = Unbundle(w176) -> (w167:bool)  [unwired: 4 out]
            n165 = Not Equal?(x=w160, y=u16 1) -> (x != y?=w158:bool)
            n166 = Not Equal?(x=w160, y=u16 3) -> (x != y?=w157:bool)
            n167 = Not Equal?(x=w165, y=u16 1) -> (x != y?=w162:bool)
            n168 = Not Equal?(x=w165, y=u16 3) -> (x != y?=w163:bool)
            n169 = case shown="Faux" w149 {
              tunnel: [T6."Disabled and Grayed Out" ("Disabled") T6."Enabled" ("Disabled")] -> w147
              frame False {
              }
              frame True {
              }
            }
            n170 = case shown="Faux" w171 {
              tunnel: [T6."Disabled and Grayed Out" ("Disabled") T6."Enabled" ("Disabled")] -> w174
              frame False {
              }
              frame True {
              }
            }
            n171 = And(x=w158, y=w157) -> (x .and. y?=w156:bool)
            n172 = And(x=w162, y=w163) -> (x .and. y?=w161:bool)
            n173 = And(x=w167, y=w156) -> (x .and. y?=w168:bool)
            n174 = case shown="Faux" w161 {
              tunnel: [T6."Disabled and Grayed Out" ("Disabled") T6."Enabled" ("Disabled")] -> w173
              frame False {
              }
              frame True {
              }
            }
            n175 = case shown="Faux" w168 {
              tunnel: [T6."Disabled and Grayed Out" ("Disabled") T6."Enabled" ("Disabled")] -> w175
              frame False {
              }
              frame True {
              }
            }
            n176 = property on="btnMesureGrain" class="Bool (strict)"("DisabledEnum"=w147) -> ()  [unwired: 2 in, 2 out]
            n177 = property on="btnVidanger" class="Bool (strict)"("DisabledEnum"=w174) -> ()  [unwired: 2 in, 2 out]
            n178 = property on="btnEtal" class="Bool (strict)"("DisabledEnum"=w173) -> ()  [unwired: 2 in, 2 out]
            n179 = property on="btnMesurePore" class="Bool (strict)"("DisabledEnum"=w175) -> ()  [unwired: 2 in, 2 out]
          }
          event "MeasureSetupButtonsVisible": Value Change {
            n180 = event-data() -> ("NewVal"=w186:bool)  [unwired: 1 in, 5 out]
            n181 = local read "MeasureMode"() -> (w188:T1)
            n182 = property on="ReferenceCellMeasure" class="NumNb (strict)"("Visible"=w186) -> ()  [unwired: 2 in, 2 out]
            n183 = property on="SampleNumber" class="Ch"("Visible"=w186) -> ()  [unwired: 2 in, 2 out]
            n184 = property on="Temperature" class="NumNb (strict)"("Visible"=w186) -> ()  [unwired: 2 in, 2 out]
            n185 = property on="Comments" class="Ch"("Visible"=w186) -> ()  [unwired: 2 in, 2 out]
            n186 = property on="SampleDepth" class="NumNb (strict)"("Visible"=w186) -> ()  [unwired: 2 in, 2 out]
            n187 = property on="DryWeight" class="NumNb (strict)"("Visible"=w186) -> ()  [unwired: 2 in, 2 out]
            n188 = property on="SampleID" class="Ch"("Visible"=w186) -> ()  [unwired: 2 in, 2 out]
            n189 = Equal?(x=w188, y=MeasureModeControl."PoreMeasure") -> (x = y?=w189:bool)
            n190 = And(x=w186, y=w189) -> (x .and. y?=w185:bool)
            n191 = property on="BulkVolume" class="NumNb (strict)"("Visible"=w185) -> ()  [unwired: 2 in, 2 out]
            n192 = property on="MeasureTotalAddedVolume" class="NumNb (strict)"("Visible"=w186) -> ()  [unwired: 2 in, 2 out]
            n193 = property on="MeasureDiskSet" class="LstDér (strict)"("Visible"=w186) -> ()  [unwired: 2 in, 2 out]
            n194 = property on="MeasureDiskVolumes" class="LstDér (strict)"("Visible"=w186) -> ()  [unwired: 2 in, 2 out]
            n195 = property on="DoMeasureMeasure" class="Bool (strict)"("Visible"=w186, "DisabledEnum"=T6."Disabled and Grayed Out" ("Disabled")) -> ()  [unwired: 2 in, 2 out]
          }
          event "ReloadDiskVolumes": Value Change {
            # "On re-remplit la liste des volumes des disques"
            # "On re-remplit la liste des volumes des disques"
            n196 = event-data() -> ()  [unwired: 1 in, 6 out]
            n197 = global read "CalibrationVolumes.vi" "AllCalibrationVolumes"() -> (w194:T13)
            n198 = global read "CalibrationVolumes.vi" "AllCalibrationVolumes"() -> (w199:T13)
            n199 = local read "MeasureDiskSet"() -> (w195:i32)
            n200 = global read "CalibrationVolumes.vi" "AllCalibrationVolumes"() -> (w210:T13)
            n201 = local read "DiskSet"() -> (w206:i32)
            n202 = To Long Integer(number=w195) -> (32bit integer=w193:i32)
            n203 = To Long Integer(number=w206) -> (32bit integer=w200:i32)
            n204 = Index Array(array=w194, index=w193) -> (element=w192:T18)
            n205 = Array Size(array=w210) -> (size(s)=w211:i32)
            n206 = Index Array(array=w199, index=w200) -> (element=w201:T18)
            n207 = Unbundle(w192) -> ("CalibrationVolumes"=w191:dbl[])  [unwired: 1 out]
            n208 = for {
              N: w211 -> [_]
              shift-right: [w218] -> w207
              shift-left: string[] [] -> [w219]
              tunnel: w210 -> [w217] mode=indexing
              shift-right: [w213] -> w208
              shift-left: i32[] [] -> [w215]
              i -> [w214]
              n209 = Insert Into Array(array=w215, new element=w214) -> (w213:i32[])  [unwired: 1 in]
              n210 = Unbundle By Name(w217) -> ("SetName"=w216:string)
              n211 = Insert Into Array(array=w219, new element=w216) -> (w218:string[])  [unwired: 1 in]
            }
            n212 = Unbundle(w201) -> ("CalibrationVolumes"=w203:dbl[])  [unwired: 1 out]
            n213 = Number To Fractional String(number=w191) -> (F-format string=w196:string[])  [unwired: 3 in]
            n214 = Number To Fractional String(number=w203) -> (F-format string=w202:string[])  [unwired: 3 in]
            n215 = property on="MeasureDiskVolumes" class="LstDér (strict)"("Item Names"=w196, "DisabledEnum"=T6."Enabled" ("Disabled"), "Val(Sgnl)"=i32[] [] ("Value (Signaling)")) -> ()  [unwired: 2 in, 2 out]
            n216 = property on="AvalaibleVolumesList" class="LstDér (strict)"("Item Names"=w202, "DisabledEnum"=T6."Enabled" ("Disabled"), "Val(Sgnl)"=i32[] [] ("Value (Signaling)")) -> ()  [unwired: 2 in, 2 out]
            n217 = property on="DiskSet" class="LstDér (strict)"("Item Names"=w207, "Item Symbols"=w208) -> ()  [unwired: 2 in, 2 out]
            n218 = property on="MeasureDiskSet" class="LstDér (strict)"("Item Names"=w207, "Item Symbols"=w208) -> ()  [unwired: 2 in, 2 out]
          }
          event "MeasureIndicatorsVisible": Value Change {
            n219 = event-data() -> ()  [unwired: 1 in, 6 out]
          }
          event "ReloadResultTableTexts": Value Change {
            n220 = event-data() -> ()  [unwired: 1 in, 6 out]
            n221 = for {
              N: 15 -> [_]
              i -> [w225]
              n222 = local read "LanguagesList"() -> (w224:i32)
              n223 = global read "LanguagesSettings.vi" "LanguageSettings"() -> (w223:T9)
              n224 = Unbundle By Name(w223) -> ("LocalisationFileContent[out]"=w222:T16)
              n225 = call "FindLocalizedString.vi"("LangIndex"=w224, "LocalizationFileContent"=w222, "WordIndex"=w225) -> ("Found"=w226:bool, "LocalizedString"=w227:string)  [unwired: 7 in]
              n226 = case shown="Faux" w226 {
                tunnel: w227 -> [_ w347]
                tunnel: ["Not found" w347] -> w221
                frame False {
                }
                frame True {
                }
              }
              n227 = case shown="Par défaut" w225 {
                tunnel: w221 -> [_ w228 w237 w246 w255 w264 w273 w282 w287 w292 w301 w310 w319 w328 w337]
                frame Default {
                }
                frame 1 {
                  n228 = local read "poreMeasuresTable"() -> (w236:string[][])
                  n229 = property on="SampleNumber" class="Ch"("Caption.Text"=w228) -> ()  [unwired: 2 in, 2 out]
                  n230 = local read "grainMeasuresTable"() -> (w229:string[][])
                  n231 = Replace Array Subset(array=w236, new element=w228, index (row)=0, index (col)=1) -> (w235:string[][])
                  n232 = local write "poreMeasuresTable"(w235) -> ()
                  n233 = Replace Array Subset(array=w229, new element=w228, index (row)=0, index (col)=1) -> (w230:string[][])
                  n234 = local write "grainMeasuresTable"(w230) -> ()
                }
                frame 2 {
                  n235 = local read "poreMeasuresTable"() -> (w245:string[][])
                  n236 = local read "grainMeasuresTable"() -> (w238:string[][])
                  n237 = property on="SampleID" class="Ch"("Caption.Text"=w237) -> ()  [unwired: 2 in, 2 out]
                  n238 = Replace Array Subset(array=w245, new element=w237, index (row)=0, index (col)=2) -> (w244:string[][])
                  n239 = local write "poreMeasuresTable"(w244) -> ()
                  n240 = Replace Array Subset(array=w238, new element=w237, index (row)=0, index (col)=2) -> (w239:string[][])
                  n241 = local write "grainMeasuresTable"(w239) -> ()
                }
                frame 3 {
                  n242 = local read "poreMeasuresTable"() -> (w254:string[][])
                  n243 = local read "grainMeasuresTable"() -> (w247:string[][])
                  n244 = property on="SampleDepth" class="NumNb (strict)"("Caption.Text"=w246) -> ()  [unwired: 2 in, 2 out]
                  n245 = Replace Array Subset(array=w254, new element=w246, index (row)=0, index (col)=3) -> (w253:string[][])
                  n246 = local write "poreMeasuresTable"(w253) -> ()
                  n247 = Replace Array Subset(array=w247, new element=w246, index (row)=0, index (col)=3) -> (w248:string[][])
                  n248 = local write "grainMeasuresTable"(w248) -> ()
                }
                frame 4 {
                  n249 = local read "poreMeasuresTable"() -> (w263:string[][])
                  n250 = local read "grainMeasuresTable"() -> (w256:string[][])
                  n251 = property on="DryWeight" class="NumNb (strict)"("Caption.Text"=w255) -> ()  [unwired: 2 in, 2 out]
                  n252 = Replace Array Subset(array=w263, new element=w255, index (row)=0, index (col)=4) -> (w262:string[][])
                  n253 = local write "poreMeasuresTable"(w262) -> ()
                  n254 = Replace Array Subset(array=w256, new element=w255, index (row)=0, index (col)=4) -> (w257:string[][])
                  n255 = local write "grainMeasuresTable"(w257) -> ()
                }
                frame 5 {
                  n256 = local read "poreMeasuresTable"() -> (w272:string[][])
                  n257 = local read "grainMeasuresTable"() -> (w265:string[][])
                  n258 = property on="BulkVolume" class="NumNb (strict)"("Caption.Text"=w264) -> ()  [unwired: 2 in, 2 out]
                  n259 = Replace Array Subset(array=w272, new element=w264, index (row)=0, index (col)=5) -> (w271:string[][])
                  n260 = local write "poreMeasuresTable"(w271) -> ()
                  n261 = Replace Array Subset(array=w265, new element=w264, index (row)=0, index (col)=5) -> (w266:string[][])
                  n262 = local write "grainMeasuresTable"(w266) -> ()
                }
                frame 6 {
                  n263 = local read "poreMeasuresTable"() -> (w281:string[][])
                  n264 = local read "grainMeasuresTable"() -> (w274:string[][])
                  n265 = Replace Array Subset(array=w281, new element=w273, index (row)=0, index (col)=6) -> (w280:string[][])
                  n266 = local write "poreMeasuresTable"(w280) -> ()
                  n267 = Replace Array Subset(array=w274, new element=w273, index (row)=0, index (col)=6) -> (w275:string[][])
                  n268 = local write "grainMeasuresTable"(w275) -> ()
                }
                frame 7 {
                  n269 = local read "poreMeasuresTable"() -> (w286:string[][])
                  n270 = Replace Array Subset(array=w286, new element=w282, index (row)=0, index (col)=7) -> (w285:string[][])
                  n271 = local write "poreMeasuresTable"(w285) -> ()
                }
                frame 8 {
                  n272 = local read "poreMeasuresTable"() -> (w291:string[][])
                  n273 = Replace Array Subset(array=w291, new element=w287, index (row)=0, index (col)=8) -> (w290:string[][])
                  n274 = local write "poreMeasuresTable"(w290) -> ()
                }
                frame 9 {
                  n275 = local read "poreMeasuresTable"() -> (w300:string[][])
                  n276 = local read "grainMeasuresTable"() -> (w293:string[][])
                  n277 = Replace Array Subset(array=w300, new element=w292, index (row)=0, index (col)=9) -> (w299:string[][])
                  n278 = local write "poreMeasuresTable"(w299) -> ()
                  n279 = Replace Array Subset(array=w293, new element=w292, index (row)=0, index (col)=7) -> (w294:string[][])
                  n280 = local write "grainMeasuresTable"(w294) -> ()
                }
                frame 10 {
                  n281 = local read "poreMeasuresTable"() -> (w309:string[][])
                  n282 = local read "grainMeasuresTable"() -> (w302:string[][])
                  n283 = Replace Array Subset(array=w309, new element=w301, index (row)=0, index (col)=10) -> (w308:string[][])
                  n284 = local write "poreMeasuresTable"(w308) -> ()
                  n285 = Replace Array Subset(array=w302, new element=w301, index (row)=0, index (col)=8) -> (w303:string[][])
                  n286 = local write "grainMeasuresTable"(w303) -> ()
                }
                frame 11 {
                  n287 = local read "poreMeasuresTable"() -> (w318:string[][])
                  n288 = local read "grainMeasuresTable"() -> (w311:string[][])
                  n289 = Replace Array Subset(array=w318, new element=w310, index (row)=0, index (col)=11) -> (w317:string[][])
                  n290 = local write "poreMeasuresTable"(w317) -> ()
                  n291 = Replace Array Subset(array=w311, new element=w310, index (row)=0, index (col)=9) -> (w312:string[][])
                  n292 = local write "grainMeasuresTable"(w312) -> ()
                }
                frame 12 {
                  n293 = local read "poreMeasuresTable"() -> (w327:string[][])
                  n294 = local read "grainMeasuresTable"() -> (w320:string[][])
                  n295 = Replace Array Subset(array=w327, new element=w319, index (row)=0, index (col)=12) -> (w326:string[][])
                  n296 = local write "poreMeasuresTable"(w326) -> ()
                  n297 = Replace Array Subset(array=w320, new element=w319, index (row)=0, index (col)=10) -> (w321:string[][])
                  n298 = local write "grainMeasuresTable"(w321) -> ()
                }
                frame 13 {
                  n299 = local read "poreMeasuresTable"() -> (w336:string[][])
                  n300 = property on="Temperature" class="NumNb (strict)"("Caption.Text"=w328) -> ()  [unwired: 2 in, 2 out]
                  n301 = local read "grainMeasuresTable"() -> (w329:string[][])
                  n302 = Replace Array Subset(array=w336, new element=w328, index (row)=0, index (col)=13) -> (w335:string[][])
                  n303 = local write "poreMeasuresTable"(w335) -> ()
                  n304 = Replace Array Subset(array=w329, new element=w328, index (row)=0, index (col)=11) -> (w330:string[][])
                  n305 = local write "grainMeasuresTable"(w330) -> ()
                }
                frame 14 {
                  n306 = local read "poreMeasuresTable"() -> (w345:string[][])
                  n307 = property on="Comments" class="Ch"("Caption.Text"=w337) -> ()  [unwired: 2 in, 2 out]
                  n308 = local read "grainMeasuresTable"() -> (w338:string[][])
                  n309 = Replace Array Subset(array=w345, new element=w337, index (row)=0, index (col)=14) -> (w344:string[][])
                  n310 = local write "poreMeasuresTable"(w344) -> ()
                  n311 = Replace Array Subset(array=w338, new element=w337, index (row)=0, index (col)=12) -> (w339:string[][])
                  n312 = local write "grainMeasuresTable"(w339) -> ()
                }
              }
            }
          }
        }
        n313 = local read "btnExit"() -> (w106:bool)
      }
      n314 = while {
        shift-right: [w349] -> _
        shift-left: w99 -> [w351]
        stop <- w352 stop-if-true
        n315 = event shown="[21] \"LanguagesList\": Valeur changée" {
          selector: _ -> [_ _ _ _ _ _ _ _ _ _ _ _ _ _ _ _ _ _ _ _ _ _ _ _ _ _ _ _ _ _ _ _ _ _ _ _ _ _ _ _ _ _ _ _ _ _ _ _ _ _ _ _ _ _ _ _ _ _ _ _ _ _ _ _ _ _]
          dyn-events: _ -> [_ _ _ _ _ _ _ _ _ _ _ _ _ _ _ _ _ _ _ _ _ _ _ _ _ _ _ _ _ _ _ _ _ _ _ _ _ _ _ _ _ _ _ _ _ _ _ _ _ _ _ _ _ _ _ _ _ _ _ _ _ _ _ _ _ _]
          timeout: 100 -> [_ _ _ _ _ _ _ _ _ _ _ _ _ _ _ _ _ _ _ _ _ _ _ _ _ _ _ _ _ _ _ _ _ _ _ _ _ _ _ _ _ _ _ _ _ _ _ _ _ _ _ _ _ _ _ _ _ _ _ _ _ _ _ _ _ _]
          tunnel: w351 -> [_ _ w376 w446 w466 _ _ _ _ _ _ _ _ _ _ _ w506 _ _ _ _ _ w834 w838 _ w865 _ _ _ _ _ _ _ w926 _ _ w974 _ _ _ w1020 _ _ _ _ _ _ _ _ _ _ _ _ _ _ _ _ _ _ _ _ w1252 _ w1264 w1286 w1319]
          tunnel: [_ _ w378 w445 w465 _ _ _ _ _ _ _ _ _ _ _ w507 _ _ _ _ _ w834 w838 _ w860 _ _ _ _ _ _ _ w925 _ _ w973 _ _ _ w1019 _ _ _ _ _ _ _ _ _ _ _ _ _ _ _ _ _ _ _ _ w1251 _ w1263 w1285 w1318] -> w348
          event "btnMesurePore": Value Change {
            # "Si la calibration est faîte, que l'on est\nen mode idle: on lance la mesure"
            n316 = event-data() -> ("NewVal"=w359:bool)  [unwired: 1 in, 5 out]
            n317 = global read "CalibrationState.vi" "CalibrationState"() -> (w358:T7)
            n318 = Unbundle(w358) -> (w357:bool)  [unwired: 4 out]
            n319 = And(x=w357, y=w359) -> (x .and. y?=w356:bool)
            n320 = case shown="Vrai" w356 {
              frame False {
              }
              frame True {
                n321 = stacked-sequence {
                  frame #0 {
                    # "On désactive le mode automatique"
                    n322 = property on="manualModeBtn" class="Bool (strict)"("Val(Sgnl)"=FALSE ("Value (Signaling)")) -> ()  [unwired: 2 in, 2 out]
                  }
                  frame #1 {
                    # "On passe en mode mesure: et on indique que c'est une mesure de pores"
                    n323 = global write "AppState.vi" "AppState"(u16 2 ("AppState")) -> ()
                    n324 = local write "MeasureMode"(MeasureModeControl."PoreMeasure" ("MeasureMode")) -> ()
                  }
                  frame #2 {
                    w363 = TRUE ("Value (Signaling)")
                    w364 = FALSE ("Value (Signaling)")
                    # "On efface/affiche les contrôles qu'il faut. On change l'état de l'app"
                    n325 = property on="MeasureSetupButtonsVisible" class="Bool (strict)"("Val(Sgnl)"=w363) -> ()  [unwired: 2 in, 2 out]
                    n326 = property on="ChangeMenuState" class="Bool (strict)"("Val(Sgnl)"=w363) -> ()  [unwired: 2 in, 2 out]
                    n327 = property on="ReloadDiskVolumes" class="Bool (strict)"("Val(Sgnl)"=w363) -> ()  [unwired: 2 in, 2 out]
                    n328 = property on="CalibrationResultsVisible" class="Bool (strict)"("Val(Sgnl)"=w364) -> ()  [unwired: 2 in, 2 out]
                    n329 = property on="CalibrationButtonsVisible" class="Bool (strict)"("Val(Sgnl)"=w364) -> ()  [unwired: 2 in, 2 out]
                    n330 = property on="MeasureIndicatorsVisible" class="Bool (strict)"("Val(Sgnl)"=w364) -> ()  [unwired: 2 in, 2 out]
                    n331 = property on="PurgeState" class="Ch"("Visible"=w364) -> ()  [unwired: 2 in, 2 out]
                    n332 = property on="ExportMeasuresButtonsVisible" class="Bool (strict)"("Val(Sgnl)"=w364) -> ()  [unwired: 2 in, 2 out]
                  }
                  frame #3 {
                    # "On change l'onglet des résultats de mesure affiché"
                    n333 = property on="MeasuresTabs" class="Onglet (strict)"("Value"=enum32{"Grain measures", "Pore measures"}."Pore measures" ("MeasuresTabs")) -> ()  [unwired: 2 in, 2 out]
                  }
                }
              }
            }
          }
          event "btnMesureGrain": Value Change {
            # "Si la calibration est faîte, que l'on est\nen mode idle: on lance la mesure"
            n334 = event-data() -> ("NewVal"=w366:bool)  [unwired: 1 in, 5 out]
            n335 = global read "CalibrationState.vi" "CalibrationState"() -> (w369:T7)
            n336 = Unbundle(w369) -> (w368:bool)  [unwired: 4 out]
            n337 = And(x=w368, y=w366) -> (x .and. y?=w367:bool)
            n338 = case shown="Vrai" w367 {
              frame False {
              }
              frame True {
                n339 = stacked-sequence {
                  frame #0 {
                    # "On désactive le mode automatique"
                    n340 = property on="manualModeBtn" class="Bool (strict)"("Val(Sgnl)"=FALSE ("Value (Signaling)")) -> ()  [unwired: 2 in, 2 out]
                  }
                  frame #1 {
                    # "On passe en mode mesure: et on indique que c'est une mesure de pores"
                    n341 = global write "AppState.vi" "AppState"(u16 2 ("AppState")) -> ()
                    n342 = local write "MeasureMode"(MeasureModeControl."GrainMeasure" ("MeasureMode")) -> ()
                  }
                  frame #2 {
                    w373 = TRUE ("Value (Signaling)")
                    w374 = FALSE ("Value (Signaling)")
                    # "On efface/affiche les contrôles qu'il faut. On change l'état de l'app"
                    n343 = property on="MeasureSetupButtonsVisible" class="Bool (strict)"("Val(Sgnl)"=w373) -> ()  [unwired: 2 in, 2 out]
                    n344 = property on="ChangeMenuState" class="Bool (strict)"("Val(Sgnl)"=w373) -> ()  [unwired: 2 in, 2 out]
                    n345 = property on="ReloadDiskVolumes" class="Bool (strict)"("Val(Sgnl)"=w373) -> ()  [unwired: 2 in, 2 out]
                    n346 = property on="CalibrationResultsVisible" class="Bool (strict)"("Val(Sgnl)"=w374) -> ()  [unwired: 2 in, 2 out]
                    n347 = property on="CalibrationButtonsVisible" class="Bool (strict)"("Val(Sgnl)"=w374) -> ()  [unwired: 2 in, 2 out]
                    n348 = property on="MeasureIndicatorsVisible" class="Bool (strict)"("Val(Sgnl)"=w374) -> ()  [unwired: 2 in, 2 out]
                    n349 = property on="PurgeState" class="Ch"("Visible"=w374) -> ()  [unwired: 2 in, 2 out]
                    n350 = property on="ExportMeasuresButtonsVisible" class="Bool (strict)"("Val(Sgnl)"=w374) -> ()  [unwired: 2 in, 2 out]
                  }
                  frame #3 {
                    # "On change l'onglet de résultats de mesures affiché"
                    n351 = property on="MeasuresTabs" class="Onglet (strict)"("Value"=enum32{"Grain measures", "Pore measures"}."Grain measures" ("MeasuresTabs")) -> ()  [unwired: 2 in, 2 out]
                  }
                }
              }
            }
          }
          event "DoMeasureMeasure": Value Change {
            # "Si on est bien dans l'état de mesure"
            n352 = event-data() -> ("NewVal"=w382:bool)  [unwired: 1 in, 5 out]
            n353 = global read "AppState.vi" "AppState"() -> (w380:u16)
            n354 = Equal?(x=w380, y=u16 2) -> (x = y?=w381:bool)
            n355 = And(x=w381, y=w382) -> (x .and. y?=w377:bool)
            n356 = case shown="Vrai" w377 {
              tunnel: w376 -> [w383 w385]
              tunnel: [w383 w384] -> w378
              frame False {
              }
              frame True {
                n357 = stacked-sequence {
                  tunnel: w385 -> [_ w402 _ _]
                  tunnel: [_ w398 _ _] -> w384
                  frame #0 {
                    n358 = property on="manualModeBtn" class="Bool (strict)"("DisabledEnum"=T6."Disabled and Grayed Out" ("Disabled"), "Val(Sgnl)"=FALSE ("Value (Signaling)")) -> ()  [unwired: 2 in, 2 out]
                  }
                  frame #1 {
                    # "Effectue la mesure et reporte la valeur"
                    n359 = local read "MeasureTotalAddedVolume"() -> (w396:dbl)
                    n360 = local read "ReferenceCellMeasure"() -> (w414:u16)
                    n361 = global read "PressureAndTimeSamples.vi" "PressureAndTimeSamples"() -> (w416:T3)
                    n362 = global read "FittedCurvePolynom.vi" "FittedCurvePolynom"() -> (w415:dbl[])
                    n363 = To Long Integer(number=w414) -> ()  [unwired: 1 out]
                    n364 = call "Measure.vi"("Graph in"=w416, "error in"=w402) -> ("error out"=w398:errorcluster, "Values"=w394:cluster{dbl[], dbl[]}, "StabilityAchieved"=w399:bool)  [unwired: 7 in]
                    n365 = local write "StabilityAchieved"(w399) -> ()
                    n366 = global write "PressureAndTimeSamples.vi" "PressureAndTimeSamples"(w394) -> ()
                    n367 = call "Horner.vi"("Meilleure poly"=w415) -> ("Y"=w395:dbl[])  [unwired: 10 in]
                    n368 = call "ElementWiseMinus.vi"("a"=w396, "Array [in]"=w395) -> ("Array[out]"=w397:dbl[])  [unwired: 9 in]
                    n369 = local read "SampleNumber"() -> (w411:string)
                    n370 = local read "SampleDepth"() -> (w409:dbl)
                    n371 = local read "Temperature"() -> (w408:dbl)
                    n372 = local read "BulkVolume"() -> (w404:dbl)
                    n373 = local read "Comments"() -> (w407:string)
                    n374 = local read "DryWeight"() -> (w403:dbl)
                    n375 = local read "SampleID"() -> (w410:string)
                    n376 = Bundle("SampleNumber"=w411, "SampleID"=w410, "SampleDepth"=w409, "DryWeight"=w403, "BulkVolume"=w404, "Temperature"=w408, "Comments"=w407) -> (w412:T19)  [unwired: 1 in]
                    n377 = local read "MeasureMode"() -> (w388:T1)
                    n378 = Index Array(array=w397, index=0) -> (element=w400:dbl)
                    n379 = local read "MeasureMode"() -> (w393:T1)
                    n380 = call "ComputeSampleData.vi"("MeasureMode"=w388, "MeasuredVolume"=w400, "UserFilledData"=w412) -> ("MeasureData"=w413:T20)  [unwired: 8 in]
                    n381 = local read "MeasureMode"() -> (w391:T1)
                    n382 = call "DataToStringArray.vi"("MeasureMode"=w393, "MeasureData"=w413) -> ("Array"=w405:string[])  [unwired: 9 in]
                    n383 = Equal?(x=w391, y=MeasureModeControl."PoreMeasure") -> (x = y?=w389:bool)
                    n384 = case shown="Vrai" w389 {
                      tunnel: [w419 w420] -> w406
                      frame False {
                        n385 = property on="grainMeasuresTable" class="Tbl (strict)"() -> ("Value"=w419:string[][])  [unwired: 2 in, 2 out]
                      }
                      frame True {
                        n386 = property on="poreMeasuresTable" class="Tbl (strict)"() -> ("Value"=w420:string[][])  [unwired: 2 in, 2 out]
                      }
                    }
                    n387 = Insert Into Array(array=w406, new element=w405) -> (w392:string[][])  [unwired: 2 in]
                    n388 = case shown="Vrai" w389 {
                      tunnel: w392 -> [w417 w418]
                      frame False {
                        n389 = property on="grainMeasuresTable" class="Tbl (strict)"("Value"=w417) -> ()  [unwired: 2 in, 2 out]
                      }
                      frame True {
                        n390 = property on="poreMeasuresTable" class="Tbl (strict)"("Value"=w418) -> ()  [unwired: 2 in, 2 out]
                      }
                    }
                  }
                  frame #2 {
                    # "Affiche/cache les boutons qu'il faut"
                    n391 = property on="MeasureIndicatorsVisible" class="Bool (strict)"("Val(Sgnl)"=TRUE) -> ()  [unwired: 2 in, 2 out]
                    n392 = global write "AppState.vi" "AppState"(u16 0 ("AppState")) -> ()
                    n393 = property on="manualModeBtn" class="Bool (strict)"("DisabledEnum"=T6."Enabled" ("Disabled")) -> ()  [unwired: 2 in, 2 out]
                    n394 = global read "LanguagesSettings.vi" "LanguageSettings"() -> (w430:T9)
                    n395 = Unbundle By Name(w430) -> ("LocalisationFileContent[out]"=w431:T16)
                    n396 = local read "StabilityAchieved"() -> (w426:bool)
                    n397 = local read "MeasureMode"() -> (w422:T1)
                    n398 = local read "LanguagesList"() -> (w427:i32)
                    n399 = case shown="Faux" w426 {
                      tunnel: [u32 131 ("WordIndex") u32 130 ("WordIndex")] -> w425
                      frame False {
                      }
                      frame True {
                      }
                    }
                    n400 = call "FindLocalizedString.vi"("LangIndex"=w427, "LocalizationFileContent"=w431, "WordIndex"=w425) -> ("Found"=w428:bool, "LocalizedString"=w429:string)  [unwired: 7 in]
                    n401 = Equal?(x=w422, y=MeasureModeControl."GrainMeasure") -> (x = y?=w423:bool)
                    n402 = case shown="Faux" w428 {
                      tunnel: w429 -> [_ w442]
                      tunnel: ["Not found" w442] -> _
                      frame False {
                      }
                      frame True {
                      }
                    }
                    n403 = case shown="Faux" w423 {
                      tunnel: [enum32{"Grain measures", "Pore measures"}."Pore measures" ("MeasuresTabs") enum32{"Grain measures", "Pore measures"}."Grain measures" ("MeasuresTabs")] -> w424
                      frame False {
                      }
                      frame True {
                      }
                    }
                    n404 = property on="MeasuresTabs" class="Onglet (strict)"("Value"=w424) -> ()  [unwired: 2 in, 2 out]
                    n405 = property on="DoMeasureMeasure" class="Bool (strict)"("Value"=FALSE ("DoMeasureMeasure")) -> ()  [unwired: 2 in, 2 out]
                    n406 = property on="MeasureSetupButtonsVisible" class="Bool (strict)"("Val(Sgnl)"=FALSE ("Value (Signaling)")) -> ()  [unwired: 2 in, 2 out]
                  }
                  frame #3 {
                    n407 = property on="ChangeMenuState" class="Bool (strict)"("Val(Sgnl)"=TRUE ("Value (Signaling)")) -> ()  [unwired: 2 in, 2 out]
                  }
                }
              }
            }
          }
          event "SaveData": Value Change {
            n408 = event-data() -> ("NewVal"=w444:bool)  [unwired: 1 in, 5 out]
            n409 = case shown="Vrai" w444 {
              tunnel: w446 -> [w447 w455]
              tunnel: [w447 w454] -> w445
              frame False {
              }
              frame True {
                n410 = call "File Dialog4"("default name"="data.csv", "error in"=w455, "pattern (all files)"="*.csv", "pattern label"="Data file") -> ("selected path"=w448:path, "cancelled"=w449:bool, "error out"=w454:errorcluster)  [unwired: 8 in, 1 out]
                n411 = Not(x=w449) -> (.not. x?=w450:bool)
                n412 = case shown="Vrai" w450 {
                  tunnel: w448 -> [_ w461]
                  frame False {
                  }
                  frame True {
                    n413 = local read "MeasureMode"() -> (w457:T1)
                    n414 = Equal?(x=w457, y=MeasureModeControl."PoreMeasure" ("MeasureMode")) -> (x = y?=w458:bool)
                    n415 = case shown="Vrai" w458 {
                      tunnel: [w462 w463] -> w459
                      frame False {
                        n416 = property on="grainMeasuresTable" class="Tbl (strict)"() -> ("Value"=w462:string[][])  [unwired: 2 in, 2 out]
                      }
                      frame True {
                        n417 = property on="poreMeasuresTable" class="Tbl (strict)"() -> ("Value"=w463:string[][])  [unwired: 2 in, 2 out]
                      }
                    }
                    n418 = call-poly <vilib>:"Write To Spreadsheet File.vi"("delimiter (\\t)"=";" ("delimiter (\\t)"), "2D data"=w459, "file path (dialog if empty)"=w461) -> ()  [unwired: 5 in, 1 out]
                  }
                }
              }
            }
          }
          event "LoadData": Value Change {
            n419 = event-data() -> ("NewVal"=w464:bool)  [unwired: 1 in, 5 out]
            n420 = case shown="Vrai" w464 {
              tunnel: w466 -> [w467 w469]
              tunnel: [w467 w468] -> w465
              frame False {
              }
              frame True {
                n421 = call "File Dialog"("default name"="data.csv", "error in"=w469, "pattern (all files)"="*.csv", "pattern label"="Data file") -> ("selected path"=w475:path, "cancelled"=w474:bool, "error out"=w468:errorcluster)  [unwired: 8 in, 1 out]
                n422 = Not(x=w474) -> (.not. x?=w473:bool)
                n423 = case shown="Vrai" w473 {
                  tunnel: w475 -> [_ w481]
                  frame False {
                  }
                  frame True {
                    n424 = call-poly <vilib>:"Read From Spreadsheet File.vi"("delimiter (\\t)"=";" ("delimiter (\\t)"), "file path (dialog if empty)"=w481) -> ("all rows"=w476:string[][])  [unwired: 5 in, 4 out]
                    n425 = local read "MeasureMode"() -> (w478:T1)
                    n426 = Equal?(x=w478, y=MeasureModeControl."PoreMeasure" ("MeasureMode")) -> (x = y?=w479:bool)
                    n427 = case shown="Vrai" w479 {
                      tunnel: w476 -> [w482 w483]
                      frame False {
                        n428 = property on="grainMeasuresTable" class="Tbl (strict)"("Value"=w482) -> ()  [unwired: 2 in, 2 out]
                      }
                      frame True {
                        n429 = property on="poreMeasuresTable" class="Tbl (strict)"("Value"=w483) -> ()  [unwired: 2 in, 2 out]
                      }
                    }
                  }
                }
              }
            }
          }
          event "ExportData": Value Change {
            n430 = event-data() -> ("NewVal"=w484:bool)  [unwired: 1 in, 5 out]
            n431 = case shown="Vrai" w484 {
              selector: w484 -> [_ w489]
              frame False {
              }
              frame True {
                w488 = FALSE ("Value (Signaling)")
                n432 = property on="ExportMeasuresButtonsVisible" class="Bool (strict)"("Val(Sgnl)"=w489) -> ()  [unwired: 2 in, 2 out]
                n433 = property on="CalibrationButtonsVisible" class="Bool (strict)"("Val(Sgnl)"=w488) -> ()  [unwired: 2 in, 2 out]
                n434 = property on="CalibrationResultsVisible" class="Bool (strict)"("Val(Sgnl)"=w488) -> ()  [unwired: 2 in, 2 out]
                n435 = property on="MeasureIndicatorsVisible" class="Bool (strict)"("Val(Sgnl)"=w488) -> ()  [unwired: 2 in, 2 out]
                n436 = property on="MeasureSetupButtonsVisible" class="Bool (strict)"("Val(Sgnl)"=w488) -> ()  [unwired: 2 in, 2 out]
                n437 = property on="PurgeState" class="Ch"("Visible"=FALSE) -> ()  [unwired: 2 in, 2 out]
                n438 = property on="ChangeMenuState" class="Bool (strict)"("Val(Sgnl)"=TRUE ("Value (Signaling)")) -> ()  [unwired: 2 in, 2 out]
                n439 = global write "AppState.vi" "AppState"(u16 5 ("AppState")) -> ()
              }
            }
          }
          event "SampleNumber": Value Change {
            n440 = event-data() -> ()  [unwired: 1 in, 6 out]
            n441 = property on="UserFilledDataChanged" class="Bool (strict)"("Val(Sgnl)"=TRUE ("Value (Signaling)")) -> ()  [unwired: 2 in, 2 out]
          }
          event "btnExit": Value Change {
            w491 = TRUE ("Visible")
            w492 = T6."Enabled" ("Disabled")
            n442 = event-data() -> ()  [unwired: 1 in, 6 out]
            n443 = property on="PurgeState" class="Ch"("Visible"=w491) -> ()  [unwired: 2 in, 2 out]
            n444 = property on="CalibrationButtonsVisible" class="Bool (strict)"("Val(Sgnl)"=w491) -> ()  [unwired: 2 in, 2 out]
            n445 = property on="CalibrationResultsVisible" class="Bool (strict)"("Val(Sgnl)"=w491) -> ()  [unwired: 2 in, 2 out]
            n446 = property on="MeasureIndicatorsVisible" class="Bool (strict)"("Val(Sgnl)"=w491) -> ()  [unwired: 2 in, 2 out]
            n447 = property on="MeasureSetupButtonsVisible" class="Bool (strict)"("Val(Sgnl)"=w491) -> ()  [unwired: 2 in, 2 out]
            n448 = property on="ExportMeasuresButtonsVisible" class="Bool (strict)"("Val(Sgnl)"=w491) -> ()  [unwired: 2 in, 2 out]
            n449 = property on="btnMesurePore" class="Bool (strict)"("DisabledEnum"=w492) -> ()  [unwired: 2 in, 2 out]
            n450 = property on="btnVidanger" class="Bool (strict)"("DisabledEnum"=w492) -> ()  [unwired: 2 in, 2 out]
            n451 = property on="btnEtal" class="Bool (strict)"("DisabledEnum"=w492) -> ()  [unwired: 2 in, 2 out]
          }
          event "MachineName": Value Change {
            n452 = event-data() -> ("NewVal"=w493:string)  [unwired: 1 in, 5 out]
            n453 = global read "MachineInfos.vi" "MachineInfos"() -> (w496:T11)
            n454 = Unbundle By Name(w496) -> ("SerialNumber"=w494:string)
            n455 = Bundle("SerialNumber"=w494, "NewVal"=w493) -> (w495:cluster{"SerialNumber":string, "NewVal":string})  [unwired: 1 in]
            n456 = global write "MachineInfos.vi" "MachineInfos"(w495) -> ()
          }
          event "SampleID": Value Change {
            n457 = event-data() -> ()  [unwired: 1 in, 6 out]
            n458 = property on="UserFilledDataChanged" class="Bool (strict)"("Val(Sgnl)"=TRUE ("Value (Signaling)")) -> ()  [unwired: 2 in, 2 out]
          }
          event "SampleDepth": Value Change {
            n459 = event-data() -> ()  [unwired: 1 in, 6 out]
            n460 = property on="UserFilledDataChanged" class="Bool (strict)"("Val(Sgnl)"=TRUE ("Value (Signaling)")) -> ()  [unwired: 2 in, 2 out]
          }
          event "DryWeight": Value Change {
            n461 = event-data() -> ()  [unwired: 1 in, 6 out]
            n462 = property on="UserFilledDataChanged" class="Bool (strict)"("Val(Sgnl)"=TRUE ("Value (Signaling)")) -> ()  [unwired: 2 in, 2 out]
          }
          event "BulkVolume": Value Change {
            n463 = event-data() -> ()  [unwired: 1 in, 6 out]
            n464 = property on="UserFilledDataChanged" class="Bool (strict)"("Val(Sgnl)"=TRUE ("Value (Signaling)")) -> ()  [unwired: 2 in, 2 out]
          }
          event "Temperature": Value Change {
            n465 = event-data() -> ()  [unwired: 1 in, 6 out]
            n466 = property on="UserFilledDataChanged" class="Bool (strict)"("Val(Sgnl)"=TRUE ("Value (Signaling)")) -> ()  [unwired: 2 in, 2 out]
          }
          event "Comments": Value Change {
            n467 = event-data() -> ()  [unwired: 1 in, 6 out]
            n468 = property on="UserFilledDataChanged" class="Bool (strict)"("Val(Sgnl)"=TRUE ("Value (Signaling)")) -> ()  [unwired: 2 in, 2 out]
          }
          event "UserFilledDataChanged": Value Change {
            n469 = event-data() -> ("NewVal"=w503:bool)  [unwired: 1 in, 5 out]
            n470 = case shown="Vrai" w503 {
              frame False {
              }
              frame True {
                n471 = local write "UserFilledDataChanged"(FALSE ("UserFilledDataChanged")) -> ()
                n472 = property on="DoMeasureMeasure" class="Bool (strict)"("DisabledEnum"=T6."Enabled" ("Disabled")) -> ()  [unwired: 2 in, 2 out]
              }
            }
          }
          event "SaveConfigChanges": Value Change {
            n473 = event-data() -> ("NewVal"=w508:bool)  [unwired: 1 in, 5 out]
            n474 = case shown="Vrai" w508 {
              tunnel: w506 -> [w509 w512]
              tunnel: [w509 w511] -> w507
              frame False {
              }
              frame True {
                n475 = flat-sequence {
                  tunnel: w512 -> [w514]
                  tunnel: [w513] -> w510
                  tunnel: [w516] -> w511
                  tunnel: w510 -> [w516]
                  frame #0 {
                    n476 = call "WriteConfiguration.vi"("error in"=w514) -> ("error out"=w513:errorcluster)  [unwired: 10 in]
                  }
                  frame #1 {
                    n477 = local write "SaveConfigChanges"(FALSE ("SaveConfigChanges")) -> ()
                  }
                }
              }
            }
          }
          event "MinimalWaitTime": Value Change {
            n478 = event-data() -> ("NewVal"=w518:u32)  [unwired: 1 in, 5 out]
            n479 = global read "StabilizationSettings.vi" "StabilizationSettings"() -> (w520:T14)
            n480 = Unbundle(w520) -> ("VarianceTrigger"=w519:dbl, "MaxWaitTime"=w517:u32)  [unwired: 1 out]
            n481 = Bundle("NewVal"=w518, "VarianceTrigger"=w519, "MaxWaitTime"=w517) -> (w521:T21)  [unwired: 1 in]
            n482 = global write "StabilizationSettings.vi" "StabilizationSettings"(w521) -> ()
          }
          event "VarianceTrigger": Value Change {
            n483 = event-data() -> ("NewVal"=w523:dbl)  [unwired: 1 in, 5 out]
            n484 = global read "StabilizationSettings.vi" "StabilizationSettings"() -> (w526:T14)
            n485 = Unbundle(w526) -> ("MinimalWaitTime"=w524:u32, "MaxWaitTime"=w522:u32)  [unwired: 1 out]
            n486 = Bundle("MinimalWaitTime"=w524, "NewVal"=w523, "MaxWaitTime"=w522) -> (w525:T22)  [unwired: 1 in]
            n487 = global write "StabilizationSettings.vi" "StabilizationSettings"(w525) -> ()
          }
          event "MaximalWaitTime": Value Change {
            n488 = event-data() -> ("NewVal"=w527:u32)  [unwired: 1 in, 5 out]
            n489 = global read "StabilizationSettings.vi" "StabilizationSettings"() -> (w531:T14)
            n490 = Unbundle(w531) -> ("MinimalWaitTime"=w529:u32, "VarianceTrigger"=w528:dbl)  [unwired: 1 out]
            n491 = Bundle("MinimalWaitTime"=w529, "VarianceTrigger"=w528, "NewVal"=w527) -> (w530:T23)  [unwired: 1 in]
            n492 = global write "StabilizationSettings.vi" "StabilizationSettings"(w530) -> ()
          }
          event "PressureCaptorConfig", "ValvesConfig": Value Change {
            n493 = event-data() -> ()  [unwired: 1 in, 6 out]
            n494 = local read "PressureCaptorConfig"() -> (w536:T4)
            n495 = Unbundle By Name(w536) -> ("Baudrate"=w545:u32, "Port"=w540:string, "Databits"=w544:u16, "Parity"=w543:u16, "Stopbits"=w542:u16, "Flow Control"=w541:u16, "Slave Address"=w538:u16, "Register Address"=w534:u16, "Timeout (ms)"=w539:u16, "MaxCaptorPressure"=w532:dbl)
            n496 = Bundle(u16 0, "Slave Address"=w538) -> (w537:cluster{u16, "Slave Address":u16})  [unwired: 1 in]
            n497 = Bundle("Baudrate"=w545, "Databits"=w544, "Parity"=w543, "Stopbits"=w542, "Flow Control"=w541, "Port"=w540, "Register Address"=w534, w537, "Timeout (ms)"=w539, "MaxCaptorPressure"=w532) -> (w535:T24)  [unwired: 1 in]
            n498 = global write "CaptParameters.vi" "CaptParameters"(w535) -> ()
          }
          event "LanguagesList": Value Change {
            n499 = event-data() -> ()  [unwired: 1 in, 6 out]
            n500 = global read "LanguagesSettings.vi" "LanguageSettings"() -> (w550:T9)
            n501 = for {
              N: 200 -> [_]
              i -> [w556]
              n502 = local read "LanguagesList"() -> (w555:i32)
              n503 = global read "LanguagesSettings.vi" "LanguageSettings"() -> (w554:T9)
              n504 = Unbundle By Name(w554) -> ("LocalisationFileContent[out]"=w553:T16)
              n505 = call "FindLocalizedString.vi"("LangIndex"=w555, "LocalizationFileContent"=w553, "WordIndex"=w556) -> ("Found"=w557:bool, "LocalizedString"=w559:string)  [unwired: 7 in]
              n506 = case shown="Faux" w557 {
                tunnel: w559 -> [_ w832]
                tunnel: ["Not found" w832] -> w558
                frame False {
                }
                frame True {
                }
              }
              n507 = case shown="85" w556 {
                tunnel: w558 -> [_ w560 w569 w578 w587 w596 w605 w614 w619 w624 w633 w642 w651 w660 w669 _ _ _ _ _ _ _ _ _ w678 w684 w689 _ w693 w694 w695 w696 w697 w699 w703 _ _ _ _ _ _ _ _ _ _ _ w707 _ _ _ _ w708 w709 _ w710 _ _ _ _ _ _ _ _ _ _ _ w711 w712 w713 w714 w715 w716 w717 _ w718 w719 w720 w721 w724 w728 w732 w735 w740 _ w744 _ w746 w747 w748 _ _ w749 w750 w751 w752 _ w753 w754 w755 _ w756 w757 w758 w759 _ w760 w767 w768 w769 w770 w771 w772 w773 w774 w775 w776 w777 w778 w779 w780 w782 w785 w789 w793 w797 w801 w805 _ _ _ _ w809 w816 w817 w821 w826]
                frame 0, Default {
                }
                frame 1 {
                  n508 = local read "poreMeasuresTable"() -> (w568:string[][])
                  n509 = property on="SampleNumber" class="Ch"("Caption.Text"=w560) -> ()  [unwired: 2 in, 2 out]
                  n510 = local read "grainMeasuresTable"() -> (w561:string[][])
                  n511 = Replace Array Subset(array=w568, new element=w560, index (row)=0, index (col)=1) -> (w567:string[][])
                  n512 = Replace Array Subset(array=w561, new element=w560, index (row)=0, index (col)=1) -> (w562:string[][])
                  n513 = local write "grainMeasuresTable"(w562) -> ()
                  n514 = local write "poreMeasuresTable"(w567) -> ()
                }
                frame 2 {
                  n515 = local read "poreMeasuresTable"() -> (w574:string[][])
                  n516 = property on="SampleID" class="Ch"("Caption.Text"=w569) -> ()  [unwired: 2 in, 2 out]
                  n517 = local read "grainMeasuresTable"() -> (w570:string[][])
                  n518 = Replace Array Subset(array=w574, new element=w569, index (row)=0, index (col)=2) -> (w577:string[][])
                  n519 = local write "poreMeasuresTable"(w577) -> ()
                  n520 = Replace Array Subset(array=w570, new element=w569, index (row)=0, index (col)=2) -> (w571:string[][])
                  n521 = local write "grainMeasuresTable"(w571) -> ()
                }
                frame 3 {
                  n522 = property on="SampleDepth" class="NumNb (strict)"("Caption.Text"=w578) -> ()  [unwired: 2 in, 2 out]
                  n523 = local read "poreMeasuresTable"() -> (w583:string[][])
                  n524 = local read "grainMeasuresTable"() -> (w579:string[][])
                  n525 = Replace Array Subset(array=w579, new element=w578, index (row)=0, index (col)=3) -> (w580:string[][])
                  n526 = Replace Array Subset(array=w583, new element=w578, index (row)=0, index (col)=3) -> (w586:string[][])
                  n527 = local write "grainMeasuresTable"(w580) -> ()
                  n528 = local write "poreMeasuresTable"(w586) -> ()
                }
                frame 4 {
                  n529 = local read "poreMeasuresTable"() -> (w595:string[][])
                  n530 = local read "grainMeasuresTable"() -> (w588:string[][])
                  n531 = property on="DryWeight" class="NumNb (strict)"("Caption.Text"=w587) -> ()  [unwired: 2 in, 2 out]
                  n532 = Replace Array Subset(array=w588, new element=w587, index (row)=0, index (col)=4) -> (w589:string[][])
                  n533 = Replace Array Subset(array=w595, new element=w587, index (row)=0, index (col)=4) -> (w594:string[][])
                  n534 = local write "grainMeasuresTable"(w589) -> ()
                  n535 = local write "poreMeasuresTable"(w594) -> ()
                }
                frame 5 {
                  n536 = property on="BulkVolume" class="NumNb (strict)"("Caption.Text"=w596) -> ()  [unwired: 2 in, 2 out]
                  n537 = local read "poreMeasuresTable"() -> (w604:string[][])
                  n538 = local read "grainMeasuresTable"() -> (w597:string[][])
                  n539 = Replace Array Subset(array=w597, new element=w596, index (row)=0, index (col)=5) -> (w598:string[][])
                  n540 = Replace Array Subset(array=w604, new element=w596, index (row)=0, index (col)=5) -> (w603:string[][])
                  n541 = local write "grainMeasuresTable"(w598) -> ()
                  n542 = local write "poreMeasuresTable"(w603) -> ()
                }
                frame 6 {
                  n543 = local read "poreMeasuresTable"() -> (w613:string[][])
                  n544 = local read "grainMeasuresTable"() -> (w606:string[][])
                  n545 = Replace Array Subset(array=w606, new element=w605, index (row)=0, index (col)=6) -> (w607:string[][])
                  n546 = Replace Array Subset(array=w613, new element=w605, index (row)=0, index (col)=6) -> (w612:string[][])
                  n547 = local write "grainMeasuresTable"(w607) -> ()
                  n548 = local write "poreMeasuresTable"(w612) -> ()
                }
                frame 7 {
                  n549 = local read "poreMeasuresTable"() -> (w618:string[][])
                  n550 = Replace Array Subset(array=w618, new element=w614, index (row)=0, index (col)=7) -> (w617:string[][])
                  n551 = local write "poreMeasuresTable"(w617) -> ()
                }
                frame 8 {
                  n552 = local read "poreMeasuresTable"() -> (w623:string[][])
                  n553 = Replace Array Subset(array=w623, new element=w619, index (row)=0, index (col)=8) -> (w622:string[][])
                  n554 = local write "poreMeasuresTable"(w622) -> ()
                }
                frame 9 {
                  n555 = local read "poreMeasuresTable"() -> (w632:string[][])
                  n556 = local read "grainMeasuresTable"() -> (w625:string[][])
                  n557 = Replace Array Subset(array=w632, new element=w624, index (row)=0, index (col)=9) -> (w631:string[][])
                  n558 = Replace Array Subset(array=w625, new element=w624, index (row)=0, index (col)=7) -> (w626:string[][])
                  n559 = local write "grainMeasuresTable"(w626) -> ()
                  n560 = local write "poreMeasuresTable"(w631) -> ()
                }
                frame 10 {
                  n561 = local read "poreMeasuresTable"() -> (w641:string[][])
                  n562 = local read "grainMeasuresTable"() -> (w634:string[][])
                  n563 = Replace Array Subset(array=w634, new element=w633, index (row)=0, index (col)=8) -> (w635:string[][])
                  n564 = Replace Array Subset(array=w641, new element=w633, index (row)=0, index (col)=10) -> (w640:string[][])
                  n565 = local write "poreMeasuresTable"(w640) -> ()
                  n566 = local write "grainMeasuresTable"(w635) -> ()
                }
                frame 11 {
                  n567 = local read "poreMeasuresTable"() -> (w650:string[][])
                  n568 = local read "grainMeasuresTable"() -> (w643:string[][])
                  n569 = Replace Array Subset(array=w643, new element=w642, index (row)=0, index (col)=9) -> (w644:string[][])
                  n570 = Replace Array Subset(array=w650, new element=w642, index (row)=0, index (col)=11) -> (w649:string[][])
                  n571 = local write "grainMeasuresTable"(w644) -> ()
                  n572 = local write "poreMeasuresTable"(w649) -> ()
                }
                frame 12 {
                  n573 = local read "poreMeasuresTable"() -> (w659:string[][])
                  n574 = local read "grainMeasuresTable"() -> (w652:string[][])
                  n575 = Replace Array Subset(array=w652, new element=w651, index (row)=0, index (col)=10) -> (w653:string[][])
                  n576 = Replace Array Subset(array=w659, new element=w651, index (row)=0, index (col)=12) -> (w658:string[][])
                  n577 = local write "poreMeasuresTable"(w658) -> ()
                  n578 = local write "grainMeasuresTable"(w653) -> ()
                }
                frame 13 {
                  n579 = property on="Temperature" class="NumNb (strict)"("Caption.Text"=w660) -> ()  [unwired: 2 in, 2 out]
                  n580 = local read "poreMeasuresTable"() -> (w668:string[][])
                  n581 = local read "grainMeasuresTable"() -> (w661:string[][])
                  n582 = Replace Array Subset(array=w668, new element=w660, index (row)=0, index (col)=13) -> (w667:string[][])
                  n583 = Replace Array Subset(array=w661, new element=w660, index (row)=0, index (col)=11) -> (w662:string[][])
                  n584 = local write "grainMeasuresTable"(w662) -> ()
                  n585 = local write "poreMeasuresTable"(w667) -> ()
                }
                frame 14 {
                  n586 = property on="Comments" class="Ch"("Caption.Text"=w669) -> ()  [unwired: 2 in, 2 out]
                  n587 = local read "poreMeasuresTable"() -> (w677:string[][])
                  n588 = local read "grainMeasuresTable"() -> (w670:string[][])
                  n589 = Replace Array Subset(array=w670, new element=w669, index (row)=0, index (col)=12) -> (w671:string[][])
                  n590 = Replace Array Subset(array=w677, new element=w669, index (row)=0, index (col)=14) -> (w676:string[][])
                  n591 = local write "grainMeasuresTable"(w671) -> ()
                  n592 = local write "poreMeasuresTable"(w676) -> ()
                }
                frame 15 {
                }
                frame 16 {
                }
                frame 17 {
                }
                frame 18 {
                }
                frame 19 {
                }
                frame 20 {
                }
                frame 21 {
                }
                frame 22 {
                }
                frame 23 {
                }
                frame 24 {
                  n593 = property on="AppTab" class="Onglet (strict)"() -> ("Pages"=w682:refnum<vi>[])  [unwired: 2 in, 2 out]
                  n594 = Index Array(array=w682, index=0) -> (element=w680:refnum<vi>)
                  n595 = property class="Page"(reference=w680, "IndependentLabel"=TRUE, "TabCaption"=w678) -> ()  [unwired: 1 in, 2 out]
                }
                frame 25 {
                  n596 = property on="AppTab" class="Onglet (strict)"() -> ("Pages"=w685:refnum<vi>[])  [unwired: 2 in, 2 out]
                  n597 = Index Array(array=w685, index=1) -> (element=w686:refnum<vi>)
                  n598 = property class="Page"(reference=w686, "IndependentLabel"=TRUE, "TabCaption"=w684) -> ()  [unwired: 1 in, 2 out]
                }
                frame 26 {
                  n599 = property on="AppTab" class="Onglet (strict)"() -> ("Pages"=w690:refnum<vi>[])  [unwired: 2 in, 2 out]
                  n600 = Index Array(array=w690, index=2) -> (element=w691:refnum<vi>)
                  n601 = property class="Page"(reference=w691, "IndependentLabel"=TRUE, "TabCaption"=w689) -> ()  [unwired: 1 in, 2 out]
                }
                frame 27 {
                }
                frame 28 {
                  n602 = property on="strInstallName" class="Ch"("Value"=w693) -> ()  [unwired: 2 in, 2 out]
                }
                frame 29 {
                  n603 = property on="btnExit" class="Bool (strict)"("BoolText.Text"=w694) -> ()  [unwired: 2 in, 2 out]
                }
                frame 30 {
                  n604 = property on="btnEtal" class="Bool (strict)"("BoolText.Text"=w695) -> ()  [unwired: 2 in, 2 out]
                }
                frame 31 {
                  n605 = property on="btnMesurePore" class="Bool (strict)"("BoolText.Text"=w696) -> ()  [unwired: 2 in, 2 out]
                }
                frame 32 {
                  n606 = property on="btnVidanger" class="Bool (strict)"("BoolText.Text"=w697) -> ()  [unwired: 2 in, 2 out]
                  n607 = property on="manualModeBtn" class="Bool (strict)"("Value"=FALSE) -> ()  [unwired: 2 in, 2 out]
                }
                frame 33 {
                  n608 = property on="manualModeBtn" class="Bool (strict)"() -> ("Strings [4]"=w702:string[])  [unwired: 2 in, 2 out]
                  n609 = Replace Array Subset(array=w702, new element=w699, index=0) -> (w701:string[])
                  n610 = property on="manualModeBtn" class="Bool (strict)"("Strings [4]"=w701) -> ()  [unwired: 2 in, 2 out]
                }
                frame 34 {
                  n611 = property on="manualModeBtn" class="Bool (strict)"() -> ("Strings [4]"=w706:string[])  [unwired: 2 in, 2 out]
                  n612 = Replace Array Subset(array=w706, new element=w703, index=1) -> (w705:string[])
                  n613 = property on="manualModeBtn" class="Bool (strict)"("Strings [4]"=w705) -> ()  [unwired: 2 in, 2 out]
                }
                frame 35 {
                }
                frame 36 {
                }
                frame 37 {
                }
                frame 38 {
                }
                frame 39 {
                }
                frame 40 {
                }
                frame 41 {
                }
                frame 42 {
                }
                frame 43 {
                }
                frame 44 {
                }
                frame 45 {
                }
                frame 46 {
                  n614 = property on="ReferenceCellCalibration" class="NumNb (strict)"("Caption.Text"=w707) -> ()  [unwired: 2 in, 2 out]
                }
                frame 47 {
                }
                frame 48 {
                }
                frame 49 {
                }
                frame 50 {
                }
                frame 51 {
                  n615 = property on="MachineName" class="Ch"("Caption.Text"=w708) -> ()  [unwired: 2 in, 2 out]
                }
                frame 52 {
                  n616 = property on="AverageAbsoluteDeviationServices" class="NumNb (strict)"("Caption.Text"=w709) -> ()  [unwired: 2 in, 2 out]
                  n617 = property on="AverageAbsoluteDeviation" class="NumNb (strict)"("Caption.Text"=w709) -> ()  [unwired: 2 in, 2 out]
                }
                frame 53 {
                }
                frame 54 {
                  n618 = property on="mdpControl" class="Ch"("Caption.Text"=w710) -> ()  [unwired: 2 in, 2 out]
                }
                frame 55 {
                }
                frame 56 {
                }
                frame 57 {
                }
                frame 58 {
                }
                frame 59 {
                }
                frame 60 {
                }
                frame 61 {
                }
                frame 62 {
                }
                frame 63 {
                }
                frame 64 {
                }
                frame 65 {
                }
                frame 66 {
                  n619 = property on="pumeActive" class="Bool (strict)"("Caption.Text"=w711) -> ()  [unwired: 2 in, 2 out]
                }
                frame 67 {
                  n620 = property on="pressureCaptorActive" class="Bool (strict)"("Caption.Text"=w712) -> ()  [unwired: 2 in, 2 out]
                }
                frame 68 {
                  n621 = property on="indicateurDefautPuissance" class="Bool (strict)"("Caption.Text"=w713) -> ()  [unwired: 2 in, 2 out]
                }
                frame 69 {
                  n622 = property on="indicateurSurpression" class="Bool (strict)"("Caption.Text"=w714) -> ()  [unwired: 2 in, 2 out]
                }
                frame 70 {
                  n623 = property on="indicateurPerteSignal" class="Bool (strict)"("Caption.Text"=w715) -> ()  [unwired: 2 in, 2 out]
                }
                frame 71 {
                  n624 = property on="rPressionM" class="NumNb (strict)"("Caption.Text"=w716) -> ()  [unwired: 2 in, 2 out]
                }
                frame 72 {
                  n625 = property on="PressureGraph" class="GraphXY (strict)"("Plot.Plot Name"=w717) -> ()  [unwired: 2 in, 2 out]
                }
                frame 73 {
                }
                frame 74 {
                  n626 = property on="MeasureDiskSet" class="LstDér (strict)"("Caption.Text"=w718) -> ()  [unwired: 2 in, 2 out]
                  n627 = property on="DiskSet" class="LstDér (strict)"("Caption.Text"=w718) -> ()  [unwired: 2 in, 2 out]
                }
                frame 77 {
                  n628 = property on="CalibrationStep" class="NumNb (strict)"("Caption.Text"=w719) -> ()  [unwired: 2 in, 2 out]
                }
                frame 78 {
                  n629 = property on="SaveCalibrationFile" class="Bool (strict)"("BoolText.Text"=w720) -> ()  [unwired: 2 in, 2 out]
                }
                frame 79 {
                  n630 = property on="RestartCalibration" class="Bool (strict)"("BoolText.Text"=w721) -> ()  [unwired: 2 in, 2 out]
                }
                frame 80 {
                  # "Idle: 0\nCalibration: 1\nMesure: 2\nVidange: 3"
                  n631 = local read "NotificationTexts"() -> (w722:string[])
                  n632 = Insert Into Array(array=w722, index=0, new element=w724) -> (w723:string[])
                  n633 = local write "NotificationTexts"(w723) -> ()
                }
                frame 81 {
                  # "Idle: 0\nCalibration: 1\nMesure: 2\nVidange: 3"
                  n634 = local read "NotificationTexts"() -> (w727:string[])
                  n635 = Insert Into Array(array=w727, index=1, new element=w728) -> (w726:string[])
                  n636 = local write "NotificationTexts"(w726) -> ()
                }
                frame 82 {
                  # "Idle: 0\nCalibration: 1\nMesure: 2\nVidange: 3"
                  n637 = local read "NotificationTexts"() -> (w730:string[])
                  n638 = Insert Into Array(array=w730, index=2, new element=w732) -> (w731:string[])
                  n639 = local write "NotificationTexts"(w731) -> ()
                }
                frame 83 {
                  # "Idle: 0\nCalibration: 1\nMesure: 2\nVidange: 3"
                  n640 = local read "NotificationTexts"() -> (w734:string[])
                  n641 = Insert Into Array(array=w734, index=3, new element=w735) -> (w736:string[])
                  n642 = local write "NotificationTexts"(w736) -> ()
                }
                frame 84 {
                  # "Idle: 0\nCalibration: 1\nMesure: 2\nVidange: 3"
                  n643 = local read "NotificationTexts"() -> (w738:string[])
                  n644 = Insert Into Array(array=w738, index=4, new element=w740) -> (w739:string[])
                  n645 = local write "NotificationTexts"(w739) -> ()
                }
                frame 85 {
                }
                frame 86 {
                  # "Idle: 0\nCalibration: 1\nMesure: 2\nVidange: 3"
                  n646 = local read "NotificationTexts"() -> (w743:string[])
                  n647 = Insert Into Array(array=w743, index=6, new element=w744) -> (w742:string[])
                  n648 = local write "NotificationTexts"(w742) -> ()
                }
                frame 87 {
                }
                frame 88 {
                  n649 = property on="PurgeState" class="Ch"("Text.Text"=w746) -> ()  [unwired: 2 in, 2 out]
                }
                frame 89 {
                  n650 = property on="PressureCaptorConfig" class="Clust (strict)"("Caption.Text"=w747) -> ()  [unwired: 2 in, 2 out]
                }
                frame 90 {
                  n651 = property on="ValvesConfig" class="Clust (strict)"("Caption.Text"=w748) -> ()  [unwired: 2 in, 2 out]
                }
                frame 91 {
                }
                frame 92 {
                }
                frame 93 {
                  n652 = property on="Pressure Offset" class="NumNb (strict)"("Caption.Text"=w749) -> ()  [unwired: 2 in, 2 out]
                }
                frame 94 {
                  n653 = property on="Pressure Gain" class="NumNb (strict)"("Caption.Text"=w750) -> ()  [unwired: 2 in, 2 out]
                }
                frame 95 {
                  n654 = property on="SaveConfigChanges" class="Bool (strict)"("BoolText.Text"=w751) -> ()  [unwired: 2 in, 2 out]
                }
                frame 96 {
                  n655 = property on="LanguagesList" class="LstDér (strict)"("Caption.Text"=w752) -> ()  [unwired: 2 in, 2 out]
                }
                frame 97 {
                }
                frame 98 {
                  n656 = property on="XYGraphService" class="GraphXY (strict)"("Caption.Text"=w753) -> ()  [unwired: 2 in, 2 out]
                }
                frame 99 {
                  n657 = property on="FittedPolynomCoeffs" class="Tabl (strict)"("Caption.Text"=w754) -> ()  [unwired: 2 in, 2 out]
                  n658 = property on="FittedPolynomCoeffsServices" class="Tabl (strict)"("Caption.Text"=w754) -> ()  [unwired: 2 in, 2 out]
                }
                frame 100 {
                  n659 = property on="ResidueInd" class="NumNb (strict)"("Caption.Text"=w755) -> ()  [unwired: 2 in, 2 out]
                  n660 = property on="ResiduServices" class="NumNb (strict)"("Caption.Text"=w755) -> ()  [unwired: 2 in, 2 out]
                }
                frame 101 {
                }
                frame 102 {
                  n661 = property on="CalibrationFilePath" class="Chm"("Caption.Text"=w756) -> ()  [unwired: 2 in, 2 out]
                }
                frame 103 {
                  n662 = property on="LoadCalibrationFileBtn" class="Bool (strict)"("BoolText.Text"=w757) -> ()  [unwired: 2 in, 2 out]
                }
                frame 104 {
                  n663 = property on="MeasureDiskVolumes" class="LstDér (strict)"("Caption.Text"=w758) -> ()  [unwired: 2 in, 2 out]
                  n664 = property on="AvalaibleVolumesList" class="LstDér (strict)"("Caption.Text"=w758) -> ()  [unwired: 2 in, 2 out]
                }
                frame 105 {
                  n665 = property on="MeasureTotalAddedVolume" class="NumNb (strict)"("Caption.Text"=w759) -> ()  [unwired: 2 in, 2 out]
                  n666 = property on="ChosenVolume" class="NumNb (strict)"("Caption.Text"=w759) -> ()  [unwired: 2 in, 2 out]
                }
                frame 106 {
                }
                frame 107 {
                  n667 = property on="DoMeasureCalibration" class="Bool (strict)"() -> ("Strings [4]"=w765:string[])  [unwired: 2 in, 2 out]
                  n668 = property on="DoMeasureMeasure" class="Bool (strict)"() -> ("Strings [4]"=w762:string[])  [unwired: 2 in, 2 out]
                  n669 = Replace Array Subset(array=w765, new element=w760, index=0) -> (w764:string[])
                  n670 = Replace Array Subset(array=w762, new element=w760, index=0) -> (w761:string[])
                  n671 = property on="DoMeasureCalibration" class="Bool (strict)"("Strings [4]"=w764) -> ()  [unwired: 2 in, 2 out]
                  n672 = property on="DoMeasureMeasure" class="Bool (strict)"("Strings [4]"=w761) -> ()  [unwired: 2 in, 2 out]
                }
                frame 108 {
                  n673 = property on="EndCalibration" class="Bool (strict)"("BoolText.Text"=w767) -> ()  [unwired: 2 in, 2 out]
                }
                frame 109 {
                  n674 = property on="poreMeasuresTable" class="Tbl (strict)"("Caption.Text"=w768) -> ()  [unwired: 2 in, 2 out]
                }
                frame 110 {
                  n675 = property on="ClearGrainMeasuresBtn" class="Bool (strict)"("BoolText.Text"=w769) -> ()  [unwired: 2 in, 2 out]
                  n676 = property on="ClearPoreMeasuresBtn" class="Bool (strict)"("BoolText.Text"=w769) -> ()  [unwired: 2 in, 2 out]
                }
                frame 111 {
                  n677 = property on="ExportToHTMLBtn" class="Bool (strict)"("BoolText.Text"=w770) -> ()  [unwired: 2 in, 2 out]
                }
                frame 112 {
                  n678 = property on="ExportGrainMeasuresBtn" class="Bool (strict)"("BoolText.Text"=w771) -> ()  [unwired: 2 in, 2 out]
                  n679 = property on="ExportPoreMeasuresBtn" class="Bool (strict)"("BoolText.Text"=w771) -> ()  [unwired: 2 in, 2 out]
                }
                frame 113 {
                  n680 = property on="SaveGrainMeasuresBtn" class="Bool (strict)"("BoolText.Text"=w772) -> ()  [unwired: 2 in, 2 out]
                  n681 = property on="SavePoreMeasuresBtn" class="Bool (strict)"("BoolText.Text"=w772) -> ()  [unwired: 2 in, 2 out]
                }
                frame 114 {
                  n682 = property on="LoadGrainMeasuresBtn" class="Bool (strict)"("BoolText.Text"=w773) -> ()  [unwired: 2 in, 2 out]
                  n683 = property on="LoadPoreMeasuresBtn" class="Bool (strict)"("BoolText.Text"=w773) -> ()  [unwired: 2 in, 2 out]
                }
                frame 115 {
                  n684 = property on="FlushPressureGraph" class="Bool (strict)"("BoolText.Text"=w774) -> ()  [unwired: 2 in, 2 out]
                }
                frame 116 {
                  n685 = property on="ExportToPDF" class="Bool (strict)"("BoolText.Text"=w775) -> ()  [unwired: 2 in, 2 out]
                }
                frame 117 {
                  n686 = property on="MaximalWaitTime" class="NumNb (strict)"("Caption.Text"=w776) -> ()  [unwired: 2 in, 2 out]
                }
                frame 118 {
                  n687 = property on="MinimalWaitTime" class="NumNb (strict)"("Caption.Text"=w777) -> ()  [unwired: 2 in, 2 out]
                }
                frame 119 {
                  n688 = property on="VarianceTrigger" class="NumNb (strict)"("Caption.Text"=w778) -> ()  [unwired: 2 in, 2 out]
                }
                frame 120 {
                  n689 = property on="SamplesMasks" class="Tabl (strict)"("Caption.Text"=w779) -> ()  [unwired: 2 in, 2 out]
                }
                frame 121 {
                  n690 = property on="ClearGrainMeasureBtn" class="Bool (strict)"("BoolText.Text"=w780) -> ()  [unwired: 2 in, 2 out]
                  n691 = property on="ClearPoreMeasureBtn" class="Bool (strict)"("BoolText.Text"=w780) -> ()  [unwired: 2 in, 2 out]
                }
                frame 122 {
                  n692 = global read "MeasureExportStrings.vi" "MeasureExportStrings"() -> (w783:string[])
                  n693 = property on="Company" class="Ch"("Caption.Text"=w782) -> ()  [unwired: 2 in, 2 out]
                  n694 = Replace Array Subset(array=w783, new element=w782, index=8) -> (w784:string[])
                  n695 = global write "MeasureExportStrings.vi" "MeasureExportStrings"(w784) -> ()
                }
                frame 123 {
                  n696 = global read "MeasureExportStrings.vi" "MeasureExportStrings"() -> (w787:string[])
                  n697 = property on="Location" class="Ch"("Caption.Text"=w785) -> ()  [unwired: 2 in, 2 out]
                  n698 = Replace Array Subset(array=w787, new element=w785, index=4) -> (w788:string[])
                  n699 = global write "MeasureExportStrings.vi" "MeasureExportStrings"(w788) -> ()
                }
                frame 124 {
                  n700 = global read "MeasureExportStrings.vi" "MeasureExportStrings"() -> (w791:string[])
                  n701 = property on="Country" class="Ch"("Caption.Text"=w789) -> ()  [unwired: 2 in, 2 out]
                  n702 = Replace Array Subset(array=w791, new element=w789, index=9) -> (w792:string[])
                  n703 = global write "MeasureExportStrings.vi" "MeasureExportStrings"(w792) -> ()
                }
                frame 125 {
                  n704 = global read "MeasureExportStrings.vi" "MeasureExportStrings"() -> (w795:string[])
                  n705 = property on="Lab" class="Ch"("Caption.Text"=w793) -> ()  [unwired: 2 in, 2 out]
                  n706 = Replace Array Subset(array=w795, new element=w793, index=10) -> (w796:string[])
                  n707 = global write "MeasureExportStrings.vi" "MeasureExportStrings"(w796) -> ()
                }
                frame 126 {
                  n708 = global read "MeasureExportStrings.vi" "MeasureExportStrings"() -> (w799:string[])
                  n709 = property on="Operator" class="Ch"("Caption.Text"=w797) -> ()  [unwired: 2 in, 2 out]
                  n710 = Replace Array Subset(array=w799, new element=w797, index=12) -> (w800:string[])
                  n711 = global write "MeasureExportStrings.vi" "MeasureExportStrings"(w800) -> ()
                }
                frame 127 {
                  n712 = global read "MeasureExportStrings.vi" "MeasureExportStrings"() -> (w803:string[])
                  n713 = property on="Field" class="Ch"("Caption.Text"=w801) -> ()  [unwired: 2 in, 2 out]
                  n714 = Replace Array Subset(array=w803, new element=w801, index=6) -> (w804:string[])
                  n715 = global write "MeasureExportStrings.vi" "MeasureExportStrings"(w804) -> ()
                }
                frame 128 {
                  n716 = global read "MeasureExportStrings.vi" "MeasureExportStrings"() -> (w807:string[])
                  n717 = Replace Array Subset(array=w807, new element=w805, index=3) -> (w808:string[])
                  n718 = property on="Well" class="Ch"("Caption.Text"=w805) -> ()  [unwired: 2 in, 2 out]
                  n719 = global write "MeasureExportStrings.vi" "MeasureExportStrings"(w808) -> ()
                }
                frame 129 {
                }
                frame 130 {
                }
                frame 131 {
                }
                frame 132 {
                }
                frame 133 {
                  n720 = property on="DoMeasureCalibration" class="Bool (strict)"() -> ("Strings [4]"=w814:string[])  [unwired: 2 in, 2 out]
                  n721 = property on="DoMeasureMeasure" class="Bool (strict)"() -> ("Strings [4]"=w811:string[])  [unwired: 2 in, 2 out]
                  n722 = Replace Array Subset(array=w814, new element=w809, index=1) -> (w813:string[])
                  n723 = Replace Array Subset(array=w811, new element=w809, index=1) -> (w810:string[])
                  n724 = property on="DoMeasureCalibration" class="Bool (strict)"("Strings [4]"=w813) -> ()  [unwired: 2 in, 2 out]
                  n725 = property on="DoMeasureMeasure" class="Bool (strict)"("Strings [4]"=w810) -> ()  [unwired: 2 in, 2 out]
                }
                frame 134 {
                  n726 = property on="Correlation" class="NumNb (strict)"("Caption.Text"=w816) -> ()  [unwired: 2 in, 2 out]
                  n727 = property on="CorrelationServices" class="NumNb (strict)"("Caption.Text"=w816) -> ()  [unwired: 2 in, 2 out]
                }
                frame 135 {
                  n728 = property on="btnMesureGrain" class="Bool (strict)"() -> ("Strings [4]"=w820:string[])  [unwired: 2 in, 2 out]
                  n729 = Replace Array Subset(array=w820, new element=w817, index=0) -> (w819:string[])
                  n730 = property on="btnMesureGrain" class="Bool (strict)"("Strings [4]"=w819) -> ()  [unwired: 2 in, 2 out]
                }
                frame 136 {
                  n731 = property on="MeasuresTabs" class="Onglet (strict)"() -> ("Pages"=w825:refnum<vi>[])  [unwired: 2 in, 2 out]
                  n732 = Index Array(array=w825, index=0) -> (element=w823:refnum<vi>)
                  n733 = property class="Page"(reference=w823, "IndependentLabel"=TRUE, "TabCaption"=w821) -> ()  [unwired: 1 in, 2 out]
                }
                frame 137 {
                  n734 = property on="MeasuresTabs" class="Onglet (strict)"() -> ("Pages"=w830:refnum<vi>[])  [unwired: 2 in, 2 out]
                  n735 = Index Array(array=w830, index=1) -> (element=w828:refnum<vi>)
                  n736 = property class="Page"(reference=w828, "IndependentLabel"=TRUE, "TabCaption"=w826) -> ()  [unwired: 1 in, 2 out]
                }
              }
            }
            n737 = local read "LanguagesList"() -> (w548:i32)
            n738 = Unbundle(w550) -> ("SupportedLanguagesList"=w547:string[], "LocalisationFileContent[out]"=w549:T16)  [unwired: 2 out]
            n739 = Index Array(array=w547, index=w548) -> (element=w546:string)
            n740 = Bundle("SupportedLanguagesList"=w547, "String"=w546, "LanguagesList"=w548, "LocalisationFileContent[out]"=w549) -> (w551:T25)  [unwired: 1 in]
            n741 = global write "LanguagesSettings.vi" "LanguageSettings"(w551) -> ()
          }
          event "SavePoreMeasuresBtn": Value Change {
            n742 = event-data() -> ("NewVal"=w833:bool)  [unwired: 1 in, 5 out]
            n743 = case shown="Vrai" w833 {
              frame False {
              }
              frame True {
                n744 = flat-sequence {
                  frame #0 {
                    n745 = local write "MeasureMode"(MeasureModeControl."PoreMeasure" ("MeasureMode")) -> ()
                  }
                  frame #1 {
                    n746 = property on="SaveData" class="Bool (strict)"("Val(Sgnl)"=TRUE ("Value (Signaling)")) -> ()  [unwired: 2 in, 2 out]
                  }
                }
              }
            }
          }
          event "LoadPoreMeasuresBtn": Value Change {
            n747 = event-data() -> ("NewVal"=w837:bool)  [unwired: 1 in, 5 out]
            n748 = case shown="Vrai" w837 {
              frame False {
              }
              frame True {
                n749 = flat-sequence {
                  frame #0 {
                    n750 = local write "MeasureMode"(MeasureModeControl."PoreMeasure" ("MeasureMode")) -> ()
                  }
                  frame #1 {
                    n751 = property on="LoadData" class="Bool (strict)"("Val(Sgnl)"=TRUE ("Value (Signaling)")) -> ()  [unwired: 2 in, 2 out]
                  }
                }
              }
            }
          }
          event "FlushPressureGraph": Value Change {
            n752 = event-data() -> ("NewVal"=w841:bool)  [unwired: 1 in, 5 out]
            n753 = case shown="Vrai" w841 {
              frame False {
              }
              frame True {
                n754 = local write "FlushPressureGraph"(FALSE ("FlushPressureGraph")) -> ()
                n755 = global read "PressureAndTimeSamples.vi" "PressureAndTimeSamples"() -> (w847:T3)
                n756 = Unbundle(w847) -> ("TimeSamples"=w846:dbl[])  [unwired: 1 out]
                n757 = Array Size(array=w846) -> (size(s)=w843:i32)
                n758 = Greater Than 0?(x=w843) -> (x > 0?=w845:bool)
                n759 = case shown="Faux" w845 {
                  tunnel: w843 -> [_ w849]
                  tunnel: [0 w849] -> w844
                  frame False {
                  }
                  frame True {
                  }
                }
                n760 = local write "FirstGraphSampleIndex"(w844) -> ()
              }
            }
          }
          event "mdpControl": Value Change {
            n761 = event-data() -> ("NewVal"=w859:string)  [unwired: 1 in, 5 out]
            n762 = call <vilib>:"Application Directory.vi"() -> ("Application Directory"=w869:path)
            n763 = Build Path(base path=w869, name or relative path=path "config.ini" ("default name")) -> (appended path=w870:path)
            n764 = call <vilib>:"Open Config Data.vi"("error in (no error)"=w865, "create file if necessary (T)"=FALSE ("create file if necessary? (T)"), "configuration file path"=w870) -> ("error out"=w868:errorcluster, "refnum"=w867:T26)  [unwired: 6 in, 1 out]
            n765 = call-poly <vilib>:"Read Key.vi"("section"="System", "error in (no error)"=w868, "key"="password", "refnum"=w867) -> ("error out"=w862:errorcluster, "value"=w852:string, "refnum out"=w861:T26)  [unwired: 4 in, 1 out]
            n766 = String Length(string=w852) -> (length=w857:i32)
            n767 = call <vilib>:"Close Config Data.vi"("error in (no error)"=w862, "write file if changed (T)"=TRUE ("write configuration file? (T)"), "refnum"=w861) -> ("error out"=w860:errorcluster)  [unwired: 8 out]
            n768 = Quotient & Remainder(x=w857, y=2) -> (floor(x/y)=w856:i32)  [unwired: 1 out]
            n769 = for {
              N: w856 -> [_]
              tunnel: w852 -> [w874]
              tunnel: [w873] -> w854 mode=indexing
              i -> [w877]
              n770 = Add(x=w877, y=w877) -> (x+y=w876:i32)
              n771 = String Subset(string=w874, offset (0)=w876, length (rest)=2 ("length (rest)")) -> (substring=w873:string)
            }
            n772 = Hexadecimal String To Number(string=w854, default (0uL)=u8 0 ("default (0 U32)")) -> (number=w853:u8[])  [unwired: 1 in, 1 out]
            n773 = Byte Array To String(unsigned byte array=w853) -> (string=w851:string)
            n774 = Equal?(x=w851, y=w859) -> (x = y?=w850:bool)
            n775 = property on="ServiceButtonsVisible" class="Bool (strict)"("Val(Sgnl)"=w850) -> ()  [unwired: 2 in, 2 out]
          }
          event "manualModeBtn": Value Change {
            n776 = event-data() -> ()  [unwired: 1 in, 6 out]
          }
          event "btnEtal": Value Change {
            n777 = event-data() -> ("NewVal"=w878:bool)  [unwired: 1 in, 5 out]
            n778 = case shown="Vrai" w878 {
              frame False {
              }
              frame True {
                n779 = stacked-sequence {
                  frame #0 {
                    # "On désactive ici\nle mode manuel\npour qu'il prenne bien effet\n(si app state n'est pas idle,\npas traité)"
                    n780 = property on="manualModeBtn" class="Bool (strict)"("Val(Sgnl)"=FALSE) -> ()  [unwired: 2 in, 2 out]
                  }
                  frame #1 {
                    # "Calibration state"
                    n781 = global read "CalibrationState.vi" "CalibrationState"() -> (w880:T7)
                    n782 = global write "AppState.vi" "AppState"(u16 1) -> ()
                    n783 = Unbundle By Name(w880) -> ("CalibrationStep"=w881:u32)
                    n784 = Unbundle(w880) -> ("CalibrationStep"=w886:u32, "Volumes"=w885:dbl[], "PressureRatios"=w884:dbl[], "Weights"=w883:bool[])  [unwired: 1 out]
                    n785 = Bundle(FALSE, "CalibrationStep"=w886, "Volumes"=w885, "PressureRatios"=w884, "Weights"=w883) -> (w887:T7)  [unwired: 1 in]
                    n786 = local write "CalibrationStep"(w881) -> ()
                    n787 = global write "CalibrationState.vi" "CalibrationState"(w887) -> ()
                  }
                  frame #2 {
                    w889 = TRUE ("Value (Signaling)")
                    w890 = FALSE ("Value (Signaling)")
                    # "Fait la transition vers l'état de calibration:\nactive et désactive les bouttons nécessaires"
                    n788 = property on="CalibrationButtonsVisible" class="Bool (strict)"("Val(Sgnl)"=w889) -> ()  [unwired: 2 in, 2 out]
                    n789 = property on="UpdateServiceGraph" class="Bool (strict)"("Val(Sgnl)"=w889) -> ()  [unwired: 2 in, 2 out]
                    n790 = property on="ChangeMenuState" class="Bool (strict)"("Val(Sgnl)"=w889) -> ()  [unwired: 2 in, 2 out]
                    n791 = property on="ReloadDiskVolumes" class="Bool (strict)"("Val(Sgnl)"=w889) -> ()  [unwired: 2 in, 2 out]
                    n792 = property on="MeasureIndicatorsVisible" class="Bool (strict)"("Val(Sgnl)"=w890) -> ()  [unwired: 2 in, 2 out]
                    n793 = property on="CalibrationResultsVisible" class="Bool (strict)"("Val(Sgnl)"=w890) -> ()  [unwired: 2 in, 2 out]
                    n794 = property on="ExportMeasuresButtonsVisible" class="Bool (strict)"("Val(Sgnl)"=w890) -> ()  [unwired: 2 in, 2 out]
                    n795 = property on="PurgeState" class="Ch"("Visible"=w890) -> ()  [unwired: 2 in, 2 out]
                    n796 = property on="MeasureSetupButtonsVisible" class="Bool (strict)"("Val(Sgnl)"=w890) -> ()  [unwired: 2 in, 2 out]
                  }
                }
              }
            }
          }
          event "RestartCalibration": Value Change {
            n797 = event-data() -> ()  [unwired: 1 in, 6 out]
            n798 = flat-sequence {
              frame #0 {
                n799 = property on="btnEtal" class="Bool (strict)"("Val(Sgnl)"=TRUE ("Value (Signaling)")) -> ()  [unwired: 2 in, 2 out]
              }
              frame #1 {
                n800 = property on="btnEtal" class="Bool (strict)"("Value"=FALSE ("btnEtal")) -> ()  [unwired: 2 in, 2 out]
              }
            }
            n801 = global write "CalibrationState.vi" "CalibrationState"(T7 {FALSE, "CalibrationStep"=0, "Volumes"=[], "PressureRatios"=[], "Weights"=[]} ("CalibrationState")) -> ()
          }
          event "DiskSet": Value Change {
            n802 = event-data() -> ()  [unwired: 1 in, 6 out]
            n803 = property on="ReloadDiskVolumes" class="Bool (strict)"("Val(Sgnl)"=TRUE ("Value (Signaling)")) -> ()  [unwired: 2 in, 2 out]
          }
          event "MeasureDiskSet": Value Change {
            n804 = event-data() -> ()  [unwired: 1 in, 6 out]
            n805 = property on="ReloadDiskVolumes" class="Bool (strict)"("Val(Sgnl)"=TRUE ("Value (Signaling)")) -> ()  [unwired: 2 in, 2 out]
          }
          event "AvalaibleVolumesList": Value Change {
            n806 = event-data() -> ()  [unwired: 1 in, 6 out]
            n807 = global read "AppState.vi" "AppState"() -> (w896:u16)
            n808 = Equal?(x=w896, y=u16 1) -> (x = y?=w898:bool)
            n809 = case shown="Vrai" w898 {
              frame False {
              }
              frame True {
                n810 = local read "AvalaibleVolumesList"() -> (w901:i32[])
                n811 = Array Size(array=w901) -> (size(s)=w902:i32)
                n812 = for {
                  N: w902 -> [_]
                  tunnel: w901 -> [w907] mode=indexing
                  shift-right: [w903] -> w899
                  shift-left: 0.0 -> [w905]
                  n813 = global read "CalibrationVolumes.vi" "AllCalibrationVolumes"() -> (w911:T13)
                  n814 = local read "DiskSet"() -> (w904:i32)
                  n815 = To Long Integer(number=w904) -> (32bit integer=w910:i32)
                  n816 = Index Array(array=w911, index=w910) -> (element=w909:T18)
                  n817 = Unbundle(w909) -> ("CalibrationVolumes"=w908:dbl[])  [unwired: 1 out]
                  n818 = Index Array(array=w908, index=w907) -> (element=w906:dbl)
                  n819 = Add(x=w905, y=w906) -> (x+y=w903:dbl)
                }
                n820 = property on="ChosenVolume" class="NumNb (strict)"("Val(Sgnl)"=w899) -> ()  [unwired: 2 in, 2 out]
              }
            }
          }
          event "MeasureDiskVolumes": Value Change {
            n821 = event-data() -> ()  [unwired: 1 in, 6 out]
            n822 = local read "MeasureDiskVolumes"() -> (w915:i32[])
            n823 = Array Size(array=w915) -> (size(s)=w912:i32)
            n824 = for {
              N: w912 -> [_]
              tunnel: w915 -> [w920] mode=indexing
              shift-right: [w917] -> w914
              shift-left: 0.0 -> [w918]
              n825 = local read "MeasureDiskSet"() -> (w916:i32)
              n826 = global read "CalibrationVolumes.vi" "AllCalibrationVolumes"() -> (w924:T13)
              n827 = To Long Integer(number=w916) -> (32bit integer=w923:i32)
              n828 = Index Array(array=w924, index=w923) -> (element=w922:T18)
              n829 = Unbundle(w922) -> ("CalibrationVolumes"=w921:dbl[])  [unwired: 1 out]
              n830 = Index Array(array=w921, index=w920) -> (element=w919:dbl)
              n831 = Add(x=w918, y=w919) -> (x+y=w917:dbl)
            }
            n832 = property on="MeasureTotalAddedVolume" class="NumNb (strict)"("Val(Sgnl)"=w914) -> ()  [unwired: 2 in, 2 out]
          }
          event "DoMeasureCalibration": Value Change {
            n833 = event-data() -> ("NewVal"=w927:bool)  [unwired: 1 in, 5 out]
            n834 = global read "AppState.vi" "AppState"() -> (w929:u16)
            n835 = Equal?(x=w929, y=u16 1) -> (x = y?=w928:bool)
            n836 = And(x=w928, y=w927) -> (x .and. y?=w931:bool)
            n837 = case shown="Vrai" w931 {
              tunnel: w926 -> [w932 w934]
              tunnel: [w932 w933] -> w925
              frame False {
              }
              frame True {
                n838 = stacked-sequence {
                  tunnel: w934 -> [_ w941 _ _]
                  tunnel: [_ w940 _ _] -> w933
                  frame #0 {
                    n839 = global write "AppState.vi" "AppState"(4) -> ()
                    n840 = property on="DoMeasureCalibration" class="Bool (strict)"("DisabledEnum"=T6."Disabled" ("Disabled")) -> ()  [unwired: 2 in, 2 out]
                    n841 = property on="manualModeBtn" class="Bool (strict)"("DisabledEnum"=T6."Disabled and Grayed Out" ("Disabled"), "Val(Sgnl)"=FALSE ("Value (Signaling)")) -> ()  [unwired: 2 in, 2 out]
                  }
                  frame #1 {
                    n842 = local read "ReferenceCellCalibration"() -> (w944:u16)
                    n843 = global read "PressureAndTimeSamples.vi" "PressureAndTimeSamples"() -> (w943:T3)
                    n844 = To Long Integer(number=w944) -> ()  [unwired: 1 out]
                    n845 = call "Measure.vi"("Graph in"=w943, "error in"=w941) -> ("error out"=w940:errorcluster, "Values"=w942:cluster{dbl[], dbl[]}, "StabilityAchieved"=w939:bool)  [unwired: 7 in]
                    n846 = global write "PressureAndTimeSamples.vi" "PressureAndTimeSamples"(w942) -> ()
                    n847 = local write "StabilityAchieved"(w939) -> ()
                  }
                  frame #2 {
                    n848 = global write "AppState.vi" "AppState"(1) -> ()
                    n849 = property on="DoMeasureCalibration" class="Bool (strict)"("Value"=FALSE ("DoCalibrationMeasure")) -> ()  [unwired: 2 in, 2 out]
                    n850 = property on="manualModeBtn" class="Bool (strict)"("DisabledEnum"=T6."Enabled" ("Disabled")) -> ()  [unwired: 2 in, 2 out]
                  }
                  frame #3 {
                    n851 = global read "LanguagesSettings.vi" "LanguageSettings"() -> (w952:T9)
                    n852 = Unbundle By Name(w952) -> ("LocalisationFileContent[out]"=w953:T16)
                    n853 = local read "StabilityAchieved"() -> (w948:bool)
                    n854 = local read "LanguagesList"() -> (w949:i32)
                    n855 = property on="CalibrationButtonsVisible" class="Bool (strict)"("Val(Sgnl)"=FALSE ("Value (Signaling)")) -> ()  [unwired: 2 in, 2 out]
                    n856 = property on="SingleCalibrationMeasureButtonsVisible" class="Bool (strict)"("Val(Sgnl)"=TRUE ("Value (Signaling)")) -> ()  [unwired: 2 in, 2 out]
                    n857 = case shown="Vrai" w948 {
                      tunnel: [u32 131 ("WordIndex") u32 130 ("WordIndex")] -> w954
                      frame False {
                      }
                      frame True {
                      }
                    }
                    n858 = call "FindLocalizedString.vi"("LangIndex"=w949, "LocalizationFileContent"=w953, "WordIndex"=w954) -> ("Found"=w950:bool, "LocalizedString"=w951:string)  [unwired: 7 in]
                    n859 = case shown="Faux" w950 {
                      tunnel: w951 -> [_ w960]
                      tunnel: ["Not found" w960] -> _
                      frame False {
                      }
                      frame True {
                      }
                    }
                  }
                }
              }
            }
          }
          event "ClearPoreMeasuresBtn": Value Change {
            n860 = event-data() -> ("NewVal"=w961:bool)  [unwired: 1 in, 5 out]
            n861 = case shown="Vrai" w961 {
              frame False {
              }
              frame True {
                n862 = stacked-sequence {
                  frame #0 {
                    n863 = property on="poreMeasuresTable" class="Tbl (strict)"("Number of Columns"=u32 15, "Number of Rows"=u32 1) -> ()  [unwired: 2 in, 2 out]
                  }
                  frame #1 {
                    n864 = property on="poreMeasuresTable" class="Tbl (strict)"("Size"=T8 {"Width"=828, "Height"=205}) -> ()  [unwired: 2 in, 2 out]
                  }
                  frame #2 {
                    n865 = property on="ClearPoreMeasuresBtn" class="Bool (strict)"("Value"=FALSE ("ClearMeasuresBtn")) -> ()  [unwired: 2 in, 2 out]
                    n866 = property on="ReloadResultTableTexts" class="Bool (strict)"("Val(Sgnl)"=TRUE ("Value (Signaling)")) -> ()  [unwired: 2 in, 2 out]
                  }
                }
              }
            }
          }
          event "ClearGrainMeasuresBtn": Value Change {
            n867 = event-data() -> ("NewVal"=w967:bool)  [unwired: 1 in, 5 out]
            n868 = case shown="Vrai" w967 {
              frame False {
              }
              frame True {
                n869 = stacked-sequence {
                  frame #0 {
                    n870 = property on="grainMeasuresTable" class="Tbl (strict)"("Number of Columns"=u32 12, "Number of Rows"=u32 1) -> ()  [unwired: 2 in, 2 out]
                  }
                  frame #1 {
                    n871 = property on="grainMeasuresTable" class="Tbl (strict)"("Size"=T8 {"Width"=828, "Height"=205}) -> ()  [unwired: 2 in, 2 out]
                  }
                  frame #2 {
                    n872 = property on="ClearGrainMeasuresBtn" class="Bool (strict)"("Value"=FALSE ("ClearMeasuresBtn")) -> ()  [unwired: 2 in, 2 out]
                    n873 = property on="ReloadResultTableTexts" class="Bool (strict)"("Val(Sgnl)"=TRUE ("Value (Signaling)")) -> ()  [unwired: 2 in, 2 out]
                  }
                }
              }
            }
          }
          event "ExportToHTMLBtn": Value Change {
            n874 = event-data() -> ("NewVal"=w975:bool)  [unwired: 1 in, 5 out]
            n875 = case shown="Vrai" w975 {
              tunnel: w974 -> [w976 w979]
              tunnel: [w976 w978] -> w973
              frame False {
              }
              frame True {
                n876 = flat-sequence {
                  tunnel: w979 -> [w985]
                  tunnel: [w984] -> w977
                  tunnel: w977 -> [w990]
                  tunnel: [w990] -> w978
                  frame #0 {
                    n877 = local read "MeasureMode"() -> (w981:T1)
                    n878 = Equal?(x=MeasureModeControl."PoreMeasure", y=w981) -> (x = y?=w982:bool)
                    n879 = case shown="Faux" w982 {
                      tunnel: [w986 w987] -> w983
                      frame False {
                        n880 = control-ref of="grainMeasuresTable"() -> (w986:refnum<vi>)
                      }
                      frame True {
                        n881 = control-ref of="poreMeasuresTable"() -> (w987:refnum<vi>)
                      }
                    }
                    n882 = call "ExportMeasuresToHTML.vi"("error in (no error)"=w985, "MeasureMode"=w981, "Table in"=w983) -> ("error out"=w984:errorcluster)  [unwired: 8 in]
                  }
                  frame #1 {
                    n883 = property on="ExportMeasuresButtonsVisible" class="Bool (strict)"("Val(Sgnl)"=FALSE ("Value (Signaling)")) -> ()  [unwired: 2 in, 2 out]
                    n884 = local write "ExportToHTMLBtn"(FALSE ("ExportToHTMLBtn")) -> ()
                  }
                }
              }
            }
          }
          event "ClearPoreMeasureBtn": Value Change {
            n885 = event-data() -> ("NewVal"=w991:bool)  [unwired: 1 in, 5 out]
            n886 = case shown="Vrai" w991 {
              frame False {
              }
              frame True {
                n887 = flat-sequence {
                  frame #0 {
                    n888 = local write "MeasureMode"(MeasureModeControl."PoreMeasure" ("MeasureMode")) -> ()
                  }
                  frame #1 {
                    n889 = property on="DeleteMeasureLine" class="Bool (strict)"("Val(Sgnl)"=TRUE ("Value (Signaling)")) -> ()  [unwired: 2 in, 2 out]
                  }
                }
              }
            }
          }
          event "ClearGrainMeasureBtn": Value Change {
            n890 = event-data() -> ("NewVal"=w994:bool)  [unwired: 1 in, 5 out]
            n891 = case shown="Vrai" w994 {
              frame False {
              }
              frame True {
                n892 = flat-sequence {
                  frame #0 {
                    n893 = local write "MeasureMode"(MeasureModeControl."GrainMeasure" ("MeasureMode")) -> ()
                  }
                  frame #1 {
                    n894 = property on="DeleteMeasureLine" class="Bool (strict)"("Val(Sgnl)"=TRUE ("Value (Signaling)")) -> ()  [unwired: 2 in, 2 out]
                  }
                }
              }
            }
          }
          event "DeleteMeasureLine": Value Change {
            n895 = event-data() -> ("NewVal"=w997:bool)  [unwired: 1 in, 5 out]
            n896 = case shown="Vrai" w997 {
              frame False {
              }
              frame True {
                w1012 = 0 ("index")
                n897 = local read "MeasureMode"() -> (w1015:T1)
                n898 = Equal?(x=w1015, y=MeasureModeControl."GrainMeasure") -> (x = y?=w1016:bool)
                n899 = case shown="Vrai" w1016 {
                  tunnel: [w1017 w1018] -> w998
                  frame False {
                    n900 = control-ref of="poreMeasuresTable"() -> (w1017:refnum<vi>)
                  }
                  frame True {
                    n901 = control-ref of="grainMeasuresTable"() -> (w1018:refnum<vi>)
                  }
                }
                n902 = property class="Tbl (strict)"(reference=w998) -> ("Active Cell"=w1013:T27)  [unwired: 1 in, 2 out]
                n903 = property class="Tbl (strict)"(reference=w998) -> ("Value"=w1009:string[][])  [unwired: 1 in, 2 out]
                n904 = Unbundle By Name(w1013) -> ("Row"=w999:i32)
                n905 = Increment(x=w999) -> (x+1=w1005:i32)
                n906 = Array Size(array=w1009) -> (size(s)=w1008:i32[])
                n907 = Index Array(array=w1008, index=0) -> (element=w1006:i32)
                n908 = Subtract(x=w1006, y=w1005) -> (x-y=w1004:i32)
                n909 = Index Array(array=w1008, index=1) -> (element=w1002:i32)
                n910 = Array Subset(array=w1009, index (row)=w1012, length (row)=w999, index (col)=w1012, length (col)=w1002) -> (w1010:string[][])
                n911 = Array Subset(array=w1009, index (row)=w1005, length (row)=w1004, index (col)=0 ("index"), length (col)=w1002) -> (w1001:string[][])
                n912 = Insert Into Array(array=w1010, new element=w1001) -> (w1000:string[][])  [unwired: 2 in]
                n913 = property class="Tbl (strict)"(reference=w998, "Value"=w1000) -> ()  [unwired: 1 in, 2 out]
              }
            }
          }
          event "ExportToPDF": Value Change {
            n914 = event-data() -> ("NewVal"=w1021:bool)  [unwired: 1 in, 5 out]
            n915 = case shown="Vrai" w1021 {
              tunnel: w1020 -> [w1022 w1024]
              tunnel: [w1022 w1023] -> w1019
              frame False {
              }
              frame True {
                n916 = flat-sequence {
                  tunnel: w1024 -> [w1030]
                  tunnel: [w1029] -> w1023
                  frame #0 {
                    n917 = local read "MeasureMode"() -> (w1026:T1)
                    n918 = Equal?(x=MeasureModeControl."PoreMeasure", y=w1026) -> (x = y?=w1027:bool)
                    n919 = case shown="Faux" w1027 {
                      tunnel: [w1031 w1032] -> w1028
                      frame False {
                        n920 = control-ref of="grainMeasuresTable"() -> (w1031:refnum<vi>)
                      }
                      frame True {
                        n921 = control-ref of="poreMeasuresTable"() -> (w1032:refnum<vi>)
                      }
                    }
                    n922 = call "ExportMeasuresToPDF.vi"("error in (no error)"=w1030, "MeasureMode"=w1026, "Table in"=w1028) -> ("error out"=w1029:errorcluster)  [unwired: 8 in]
                  }
                  frame #1 {
                    n923 = local write "ExportToPDF"(FALSE ("ExportToPDF")) -> ()
                    n924 = property on="ExportMeasuresButtonsVisible" class="Bool (strict)"("Val(Sgnl)"=FALSE ("Value (Signaling)")) -> ()  [unwired: 2 in, 2 out]
                  }
                }
              }
            }
          }
          event "ExportPoreMeasuresBtn": Value Change {
            n925 = event-data() -> ("NewVal"=w1035:bool)  [unwired: 1 in, 5 out]
            n926 = case shown="Vrai" w1035 {
              frame False {
              }
              frame True {
                n927 = flat-sequence {
                  frame #0 {
                    n928 = local write "MeasureMode"(MeasureModeControl."PoreMeasure" ("MeasureMode")) -> ()
                  }
                  frame #1 {
                    n929 = property on="ExportData" class="Bool (strict)"("Val(Sgnl)"=TRUE ("Value (Signaling)")) -> ()  [unwired: 2 in, 2 out]
                  }
                }
              }
            }
          }
          event "LoadGrainMeasuresBtn": Value Change {
            n930 = event-data() -> ("NewVal"=w1038:bool)  [unwired: 1 in, 5 out]
            n931 = case shown="Vrai" w1038 {
              frame False {
              }
              frame True {
                n932 = flat-sequence {
                  frame #0 {
                    n933 = local write "MeasureMode"(MeasureModeControl."GrainMeasure" ("MeasureMode")) -> ()
                  }
                  frame #1 {
                    n934 = property on="LoadData" class="Bool (strict)"("Val(Sgnl)"=TRUE ("Value (Signaling)")) -> ()  [unwired: 2 in, 2 out]
                  }
                }
              }
            }
          }
          event "SaveGrainMeasuresBtn": Value Change {
            n935 = event-data() -> ("NewVal"=w1041:bool)  [unwired: 1 in, 5 out]
            n936 = case shown="Vrai" w1041 {
              frame False {
              }
              frame True {
                n937 = flat-sequence {
                  frame #0 {
                    n938 = local write "MeasureMode"(MeasureModeControl."GrainMeasure" ("MeasureMode")) -> ()
                  }
                  frame #1 {
                    n939 = property on="SaveData" class="Bool (strict)"("Val(Sgnl)"=TRUE ("Value (Signaling)")) -> ()  [unwired: 2 in, 2 out]
                  }
                }
              }
            }
          }
          event "ExportGrainMeasuresBtn": Value Change {
            n940 = event-data() -> ("NewVal"=w1044:bool)  [unwired: 1 in, 5 out]
            n941 = case shown="Vrai" w1044 {
              frame False {
              }
              frame True {
                n942 = flat-sequence {
                  frame #0 {
                    n943 = local write "MeasureMode"(MeasureModeControl."GrainMeasure" ("MeasureMode")) -> ()
                  }
                  frame #1 {
                    n944 = property on="ExportData" class="Bool (strict)"("Val(Sgnl)"=TRUE ("Value (Signaling)")) -> ()  [unwired: 2 in, 2 out]
                  }
                }
              }
            }
          }
          event "Location": Value Change {
            n945 = event-data() -> ("NewVal"=w1047:string)  [unwired: 1 in, 5 out]
            n946 = global read "UserInfos.vi" "UserInfos"() -> (w1058:T28)
            n947 = Unbundle(w1058) -> ("Field"=w1056:string, "Company"=w1055:string, "Lab"=w1054:string, "Operator"=w1053:string, "Well"=w1052:string, "Lat/Long"=w1051:string, "Formation"=w1050:string, "Country"=w1049:string, "Client"=w1048:string)  [unwired: 1 out]
            n948 = Bundle("NewVal"=w1047, "Field"=w1056, "Company"=w1055, "Lab"=w1054, "Operator"=w1053, "Well"=w1052, "Lat/Long"=w1051, "Formation"=w1050, "Country"=w1049, "Client"=w1048) -> (w1057:T29)  [unwired: 1 in]
            n949 = global write "UserInfos.vi" "UserInfos"(w1057) -> ()
          }
          event "Field": Value Change {
            n950 = event-data() -> ("NewVal"=w1067:string)  [unwired: 1 in, 5 out]
            n951 = global read "UserInfos.vi" "UserInfos"() -> (w1070:T28)
            n952 = Unbundle(w1070) -> ("location"=w1068:string, "Company"=w1066:string, "Lab"=w1065:string, "Operator"=w1064:string, "Well"=w1063:string, "Lat/Long"=w1062:string, "Formation"=w1061:string, "Country"=w1060:string, "Client"=w1059:string)  [unwired: 1 out]
            n953 = Bundle("location"=w1068, "NewVal"=w1067, "Company"=w1066, "Lab"=w1065, "Operator"=w1064, "Well"=w1063, "Lat/Long"=w1062, "Formation"=w1061, "Country"=w1060, "Client"=w1059) -> (w1069:T30)  [unwired: 1 in]
            n954 = global write "UserInfos.vi" "UserInfos"(w1069) -> ()
          }
          event "Company": Value Change {
            n955 = event-data() -> ("NewVal"=w1078:string)  [unwired: 1 in, 5 out]
            n956 = global read "UserInfos.vi" "UserInfos"() -> (w1081:T28)
            n957 = Unbundle(w1081) -> ("location"=w1080:string, "Field"=w1079:string, "Lab"=w1077:string, "Operator"=w1076:string, "Well"=w1075:string, "Lat/Long"=w1074:string, "Formation"=w1073:string, "Country"=w1072:string, "Client"=w1071:string)  [unwired: 1 out]
            n958 = Bundle("location"=w1080, "Field"=w1079, "NewVal"=w1078, "Lab"=w1077, "Operator"=w1076, "Well"=w1075, "Lat/Long"=w1074, "Formation"=w1073, "Country"=w1072, "Client"=w1071) -> (w1082:T31)  [unwired: 1 in]
            n959 = global write "UserInfos.vi" "UserInfos"(w1082) -> ()
          }
          event "Lab": Value Change {
            n960 = event-data() -> ("NewVal"=w1089:string)  [unwired: 1 in, 5 out]
            n961 = global read "UserInfos.vi" "UserInfos"() -> (w1094:T28)
            n962 = Unbundle(w1094) -> ("location"=w1092:string, "Field"=w1091:string, "Company"=w1090:string, "Operator"=w1088:string, "Well"=w1087:string, "Lat/Long"=w1086:string, "Formation"=w1085:string, "Country"=w1084:string, "Client"=w1083:string)  [unwired: 1 out]
            n963 = Bundle("location"=w1092, "Field"=w1091, "Company"=w1090, "NewVal"=w1089, "Operator"=w1088, "Well"=w1087, "Lat/Long"=w1086, "Formation"=w1085, "Country"=w1084, "Client"=w1083) -> (w1093:T32)  [unwired: 1 in]
            n964 = global write "UserInfos.vi" "UserInfos"(w1093) -> ()
          }
          event "ChosenVolume": Value Change {
            n965 = event-data() -> ()  [unwired: 1 in, 6 out]
            n966 = global read "AppState.vi" "AppState"() -> (w1096:u16)
            n967 = Equal?(x=w1096, y=u16 1) -> (x = y?=w1097:bool)
            n968 = case shown="Vrai" w1097 {
              frame False {
              }
              frame True {
                n969 = property on="DoMeasureCalibration" class="Bool (strict)"("DisabledEnum"=T6."Enabled" ("Disabled")) -> ()  [unwired: 2 in, 2 out]
              }
            }
          }
          event "Operator": Value Change {
            n970 = event-data() -> ("NewVal"=w1104:string)  [unwired: 1 in, 5 out]
            n971 = global read "UserInfos.vi" "UserInfos"() -> (w1110:T28)
            n972 = Unbundle(w1110) -> ("location"=w1108:string, "Field"=w1107:string, "Company"=w1106:string, "Lab"=w1105:string, "Well"=w1103:string, "Lat/Long"=w1102:string, "Formation"=w1101:string, "Country"=w1100:string, "Client"=w1099:string)  [unwired: 1 out]
            n973 = Bundle("location"=w1108, "Field"=w1107, "Company"=w1106, "Lab"=w1105, "NewVal"=w1104, "Well"=w1103, "Lat/Long"=w1102, "Formation"=w1101, "Country"=w1100, "Client"=w1099) -> (w1109:T33)  [unwired: 1 in]
            n974 = global write "UserInfos.vi" "UserInfos"(w1109) -> ()
          }
          event "Well": Value Change {
            n975 = event-data() -> ("NewVal"=w1115:string)  [unwired: 1 in, 5 out]
            n976 = global read "UserInfos.vi" "UserInfos"() -> (w1122:T28)
            n977 = Unbundle(w1122) -> ("location"=w1120:string, "Field"=w1119:string, "Company"=w1118:string, "Lab"=w1117:string, "Operator"=w1116:string, "Lat/Long"=w1114:string, "Formation"=w1113:string, "Country"=w1111:string, "Client"=w1112:string)  [unwired: 1 out]
            n978 = Bundle("location"=w1120, "Field"=w1119, "Company"=w1118, "Lab"=w1117, "Operator"=w1116, "NewVal"=w1115, "Lat/Long"=w1114, "Formation"=w1113, "Country"=w1111, "Client"=w1112) -> (w1121:T34)  [unwired: 1 in]
            n979 = global write "UserInfos.vi" "UserInfos"(w1121) -> ()
          }
          event "LatitudeLongitude": Value Change {
            n980 = event-data() -> ("NewVal"=w1126:string)  [unwired: 1 in, 5 out]
            n981 = global read "UserInfos.vi" "UserInfos"() -> (w1133:T28)
            n982 = Unbundle(w1133) -> ("location"=w1132:string, "Field"=w1131:string, "Company"=w1130:string, "Lab"=w1129:string, "Operator"=w1128:string, "Well"=w1127:string, "Formation"=w1125:string, "Country"=w1124:string, "Client"=w1123:string)  [unwired: 1 out]
            n983 = Bundle("location"=w1132, "Field"=w1131, "Company"=w1130, "Lab"=w1129, "Operator"=w1128, "Well"=w1127, "NewVal"=w1126, "Formation"=w1125, "Country"=w1124, "Client"=w1123) -> (w1134:T35)  [unwired: 1 in]
            n984 = global write "UserInfos.vi" "UserInfos"(w1134) -> ()
          }
          event "Formation": Value Change {
            n985 = event-data() -> ("NewVal"=w1137:string)  [unwired: 1 in, 5 out]
            n986 = global read "UserInfos.vi" "UserInfos"() -> (w1146:T28)
            n987 = Unbundle(w1146) -> ("location"=w1144:string, "Field"=w1143:string, "Company"=w1142:string, "Lab"=w1141:string, "Operator"=w1140:string, "Well"=w1139:string, "Lat/Long"=w1138:string, "Country"=w1136:string, "Client"=w1135:string)  [unwired: 1 out]
            n988 = Bundle("location"=w1144, "Field"=w1143, "Company"=w1142, "Lab"=w1141, "Operator"=w1140, "Well"=w1139, "Lat/Long"=w1138, "NewVal"=w1137, "Country"=w1136, "Client"=w1135) -> (w1145:T36)  [unwired: 1 in]
            n989 = global write "UserInfos.vi" "UserInfos"(w1145) -> ()
          }
          event "Country": Value Change {
            n990 = event-data() -> ("NewVal"=w1148:string)  [unwired: 1 in, 5 out]
            n991 = global read "UserInfos.vi" "UserInfos"() -> (w1157:T28)
            n992 = Unbundle(w1157) -> ("location"=w1156:string, "Field"=w1155:string, "Company"=w1154:string, "Lab"=w1153:string, "Operator"=w1152:string, "Well"=w1151:string, "Lat/Long"=w1150:string, "Formation"=w1149:string, "Client"=w1147:string)  [unwired: 1 out]
            n993 = Bundle("location"=w1156, "Field"=w1155, "Company"=w1154, "Lab"=w1153, "Operator"=w1152, "Well"=w1151, "Lat/Long"=w1150, "Formation"=w1149, "NewVal"=w1148, "Client"=w1147) -> (w1158:T37)  [unwired: 1 in]
            n994 = global write "UserInfos.vi" "UserInfos"(w1158) -> ()
          }
          event "Client": Value Change {
            n995 = event-data() -> ("NewVal"=w1159:string)  [unwired: 1 in, 5 out]
            n996 = global read "UserInfos.vi" "UserInfos"() -> (w1168:T28)
            n997 = Unbundle(w1168) -> ("location"=w1170:string, "Field"=w1167:string, "Company"=w1166:string, "Lab"=w1165:string, "Operator"=w1163:string, "Well"=w1164:string, "Lat/Long"=w1162:string, "Formation"=w1161:string, "Country"=w1160:string)  [unwired: 1 out]
            n998 = Bundle("location"=w1170, "Field"=w1167, "Company"=w1166, "Lab"=w1165, "Operator"=w1163, "Well"=w1164, "Lat/Long"=w1162, "Formation"=w1161, "Country"=w1160, "NewVal"=w1159) -> (w1169:T38)  [unwired: 1 in]
            n999 = global write "UserInfos.vi" "UserInfos"(w1169) -> ()
          }
          event "EndCalibration": Value Change {
            n1000 = event-data() -> ()  [unwired: 1 in, 6 out]
            n1001 = global read "CalibrationState.vi" "CalibrationState"() -> (w1174:T7)
            n1002 = Unbundle(w1174) -> ("CalibrationStep"=w1173:u32)  [unwired: 4 out]
            n1003 = Greater Or Equal?(x=w1173, y=u32 6) -> (x >= y?=w1171:bool)
            n1004 = case shown="Vrai" w1171 {
              frame False {
              }
              frame True {
                n1005 = stacked-sequence {
                  frame #0 {
                    n1006 = property on="ComputeCalibrationResult" class="Bool (strict)"("Val(Sgnl)"=TRUE ("Value (Signaling)")) -> ()  [unwired: 2 in, 2 out]
                  }
                  frame #1 {
                    # "On marque l'état de calibration"
                    n1007 = global read "CalibrationState.vi" "CalibrationState"() -> (w1182:T7)
                    n1008 = Unbundle(w1182) -> ("CalibrationStep"=w1178:u32, "Volumes"=w1180:dbl[], "PressureRatios"=w1179:dbl[], "Weights"=w1176:bool[])  [unwired: 1 out]
                    n1009 = Bundle(TRUE, "CalibrationStep"=w1178, "Volumes"=w1180, "PressureRatios"=w1179, "Weights"=w1176) -> (w1181:T7)  [unwired: 1 in]
                    n1010 = global write "CalibrationState.vi" "CalibrationState"(w1181) -> ()
                  }
                  frame #2 {
                    # "On repasse en mode idle"
                    n1011 = global write "AppState.vi" "AppState"(u16 0) -> ()
                  }
                  frame #3 {
                    w1185 = TRUE ("Value (Signaling)")
                    # "On affiche cache ce qu'il faut"
                    n1012 = property on="ChangeMenuState" class="Bool (strict)"("Val(Sgnl)"=w1185) -> ()  [unwired: 2 in, 2 out]
                    n1013 = property on="CalibrationResultsVisible" class="Bool (strict)"("Val(Sgnl)"=w1185) -> ()  [unwired: 2 in, 2 out]
                    n1014 = property on="CalibrationButtonsVisible" class="Bool (strict)"("Val(Sgnl)"=FALSE ("Value (Signaling)")) -> ()  [unwired: 2 in, 2 out]
                    n1015 = property on="FittedPolynomCoeffs" class="Tabl (strict)"("DisabledEnum"=T6."Enabled" ("Disabled")) -> ()  [unwired: 2 in, 2 out]
                  }
                }
              }
            }
          }
          event "ComputeCalibrationResult": Value Change {
            n1016 = event-data() -> ("NewVal"=w1187:bool)  [unwired: 1 in, 5 out]
            n1017 = case shown="Vrai" w1187 {
              frame False {
              }
              frame True {
                n1018 = stacked-sequence {
                  frame #0 {
                    # "On calcule le polynôme interpolateur"
                    n1019 = global read "CalibrationState.vi" "CalibrationState"() -> (w1198:T7)
                    n1020 = Unbundle(w1198) -> ("Volumes"=w1192:dbl[], "PressureRatios"=w1190:dbl[], "Weights"=w1191:bool[])  [unwired: 2 out]
                    n1021 = global read "FittedCurvePolynom.vi" "FittedCurvePolynom"() -> (w1199:dbl[])
                    n1022 = local read "ResiduServices"() -> (w1196:dbl)
                    n1023 = call "GetSelectedElements.vi"("Masks"=w1191, "Array[in]"=w1190) -> ("Array[out]"=w1188:dbl[])  [unwired: 9 in]
                    n1024 = call "GetSelectedElements.vi"("Masks"=w1191, "Array[in]"=w1192) -> ("Array[out]"=w1189:dbl[])  [unwired: 9 in]
                    n1025 = call "CalculerPolynome.vi"("Résidu [in]"=w1196, "e3 [in]"=1e-06, "Meilleure poly [in]"=w1199, "Y"=w1189, "X"=w1188) -> ("Résidu [out]"=w1194:dbl, "Meilleur poly [out]"=w1197:dbl[])  [unwired: 5 in]
                    n1026 = global write "FittedCurvePolynom.vi" "FittedCurvePolynom"(w1197) -> ()
                    n1027 = local write "FittedPolynomCoeffsServices"(w1197) -> ()
                    n1028 = local write "FittedPolynomCoeffs"(w1197) -> ()
                    n1029 = Square Root(x=w1194) -> (sqrt(x)=w1193:dbl)
                    n1030 = local write "ResiduServices"(w1193) -> ()
                    n1031 = local write "ResidueInd"(w1193) -> ()
                  }
                  frame #1 {
                    # "On ajoute les indicateurs de bonnes calibration (corrélation, average abs deviation)"
                    n1032 = global read "CalibrationState.vi" "CalibrationState"() -> (w1211:T7)
                    n1033 = Unbundle(w1211) -> ("Volumes"=w1202:dbl[], "PressureRatios"=w1204:dbl[], "Weights"=w1200:bool[])  [unwired: 2 out]
                    n1034 = global read "FittedCurvePolynom.vi" "FittedCurvePolynom"() -> (w1210:dbl[])
                    n1035 = call "GetSelectedElements.vi"("Masks"=w1200, "Array[in]"=w1204) -> ("Array[out]"=w1203:dbl[])  [unwired: 9 in]
                    n1036 = call "GetSelectedElements.vi"("Masks"=w1200, "Array[in]"=w1202) -> ("Array[out]"=w1201:dbl[])  [unwired: 9 in]
                    n1037 = call "Horner.vi"("Meilleure poly"=w1210, "X"=w1203) -> ("Y"=w1208:dbl[])  [unwired: 9 in]
                    n1038 = call "ArraySubstraction.vi"("Y [in]"=w1208, "X [in]"=w1201) -> ("Array[out]"=w1207:dbl[])  [unwired: 9 in]
                    n1039 = call "Correlation.vi"("Y"=w1208, "X"=w1201) -> ("c"=w1209:dbl)  [unwired: 9 in]
                    n1040 = local write "CorrelationServices"(w1209) -> ()
                    n1041 = local write "Correlation"(w1209) -> ()
                    n1042 = call "ElementWiseAbs.vi"("Array [in]"=w1207) -> ("Array[out]"=w1206:dbl[])  [unwired: 10 in]
                    n1043 = call "Mean.vi"("Array"=w1206) -> ("Mean"=w1205:dbl)  [unwired: 10 in]
                    n1044 = local write "AverageAbsoluteDeviation"(w1205) -> ()
                    n1045 = local write "AverageAbsoluteDeviationServices"(w1205) -> ()
                  }
                  frame #2 {
                    # "On actualise le graphe de service"
                    n1046 = property on="UpdateServiceGraph" class="Bool (strict)"("Val(Sgnl)"=TRUE ("Value (Signaling)")) -> ()  [unwired: 2 in, 2 out]
                  }
                }
              }
            }
          }
          event "UpdateServiceGraph": Value Change {
            n1047 = event-data() -> ()  [unwired: 1 in, 6 out]
            n1048 = global read "CalibrationState.vi" "CalibrationState"() -> (w1219:T7)
            n1049 = Unbundle(w1219) -> (w1214:bool, "Volumes"=w1216:dbl[], "PressureRatios"=w1221:dbl[], "Weights"=w1213:bool[])  [unwired: 1 out]
            n1050 = local write "SamplesMasks"(w1213) -> ()
            n1051 = call "GetSelectedElements.vi"("Masks"=w1213, "Array[in]"=w1216) -> ("Array[out]"=w1215:dbl[])  [unwired: 9 in]
            n1052 = call "GetSelectedElements.vi"("Masks"=w1213, "Array[in]"=w1221) -> ("Array[out]"=w1222:dbl[])  [unwired: 9 in]
            n1053 = case shown="Vrai" w1214 {
              tunnel: w1222 -> [_ w1229]
              tunnel: [cluster{"Array":dbl[], "Y":dbl[]} {"Array"=[], "Y"=[]} w1227] -> w1217
              frame False {
              }
              frame True {
                n1054 = global read "FittedCurvePolynom.vi" "FittedCurvePolynom"() -> (w1225:dbl[])
                n1055 = call "Interpolate.vi"("X"=w1229, "Points interpolation"=u32 1000) -> ("Array"=w1228:dbl[])  [unwired: 9 in]
                n1056 = call "Horner.vi"("Meilleure poly"=w1225, "X"=w1228) -> ("Y"=w1226:dbl[])  [unwired: 9 in]
                n1057 = Bundle("Array"=w1228, "Y"=w1226) -> (w1227:cluster{"Array":dbl[], "Y":dbl[]})  [unwired: 1 in]
              }
            }
            n1058 = Bundle("Array[out]"=w1222, "Array[out]"=w1215) -> (w1220:cluster{"Array[out]":dbl[], "Array[out]":dbl[]})  [unwired: 1 in]
            n1059 = Build Array(w1220, w1217) -> (w1218:cluster{"Array":dbl[], "Y":dbl[]}[])
            n1060 = local write "XYGraphService"(w1218) -> ()
          }
          event "SamplesMasks": Value Change {
            n1061 = event-data() -> ("NewVal"=w1230:bool[])  [unwired: 1 in, 5 out]
            n1062 = stacked-sequence {
              tunnel: w1230 -> [w1233 _ _]
              frame #0 {
                # "Change l'état de calibration pour mettre les nouveaux masques"
                n1063 = global read "CalibrationState.vi" "CalibrationState"() -> (w1240:T7)
                n1064 = Unbundle(w1240) -> (w1238:bool, "CalibrationStep"=w1237:u32, "Volumes"=w1236:dbl[], "PressureRatios"=w1235:dbl[], "Weights"=w1234:bool[])
                n1065 = Replace Array Subset(array=w1234, new element=w1233, index=0) -> (w1231:bool[])
                n1066 = Bundle(w1238, "CalibrationStep"=w1237, "Volumes"=w1236, "PressureRatios"=w1235, "Weights"=w1231) -> (w1239:T7)  [unwired: 1 in]
                n1067 = global write "CalibrationState.vi" "CalibrationState"(w1239) -> ()
              }
              frame #1 {
                # "Recalcul le polynome si nécessaire"
                n1068 = global read "CalibrationState.vi" "CalibrationState"() -> (w1242:T7)
                n1069 = Unbundle(w1242) -> (w1241:bool)  [unwired: 4 out]
                n1070 = case shown="Vrai" w1241 {
                  frame False {
                  }
                  frame True {
                    n1071 = property on="ComputeCalibrationResult" class="Bool (strict)"("Val(Sgnl)"=TRUE ("Value (Signaling)")) -> ()  [unwired: 2 in, 2 out]
                  }
                }
              }
              frame #2 {
                # "Dans tous les cas, met à jour le graphe de service"
                n1072 = property on="UpdateServiceGraph" class="Bool (strict)"("Val(Sgnl)"=TRUE ("Value (Signaling)")) -> ()  [unwired: 2 in, 2 out]
              }
            }
          }
          event "CalibrationFilePath": Value Change {
            n1073 = event-data() -> ("NewVal"=w1247:path)  [unwired: 1 in, 5 out]
            n1074 = Not Equal?(x=path "", y=w1247) -> (x != y?=w1248:bool)
            n1075 = case shown="Faux" w1248 {
              tunnel: [T6."Disabled and Grayed Out" ("Disabled") T6."Enabled" ("Disabled")] -> w1245
              frame False {
              }
              frame True {
              }
            }
            n1076 = property on="LoadCalibrationFileBtn" class="Bool (strict)"("DisabledEnum"=w1245) -> ()  [unwired: 2 in, 2 out]
          }
          event "LoadCalibrationFileBtn": Value Change {
            n1077 = event-data() -> ("NewVal"=w1253:bool)  [unwired: 1 in, 5 out]
            n1078 = case shown="Faux" w1253 {
              tunnel: w1252 -> [w1254 w1256]
              tunnel: [w1254 w1255] -> w1251
              frame False {
              }
              frame True {
                n1079 = stacked-sequence {
                  tunnel: w1256 -> [w1258 _ _]
                  tunnel: [w1257 _ _] -> w1255
                  frame #0 {
                    n1080 = local read "CalibrationFilePath"() -> (w1260:path)
                    n1081 = call "LoadCalibrationFile.vi"("error in (no error)"=w1258, "Path"=w1260) -> ("error out"=w1257:errorcluster, "CalibrationState"=w1259:T7)  [unwired: 8 in]
                    n1082 = global write "CalibrationState.vi" "CalibrationState"(w1259) -> ()
                  }
                  frame #1 {
                    n1083 = property on="btnEtal" class="Bool (strict)"("Val(Sgnl)"=TRUE ("Value (Signaling)")) -> ()  [unwired: 2 in, 2 out]
                  }
                  frame #2 {
                    n1084 = property on="btnEtal" class="Bool (strict)"("Value"=FALSE ("btnEtal")) -> ()  [unwired: 2 in, 2 out]
                  }
                }
              }
            }
          }
          event Timeout {
            n1085 = event-data() -> ()  [unwired: 1 in, 3 out]
          }
          event "SaveCalibrationFile": Value Change {
            n1086 = event-data() -> ("NewVal"=w1265:bool)  [unwired: 1 in, 5 out]
            n1087 = case shown="Vrai" w1265 {
              tunnel: w1264 -> [w1266 w1272]
              tunnel: [w1266 w1269] -> w1263
              frame False {
              }
              frame True {
                n1088 = Default Directory() -> (w1273:path)
                n1089 = call "File Dialog3"("start path"=w1273, "default name"="calibration.txt", "error in"=w1272, "pattern (all files)"="*.txt") -> ("selected path"=w1270:path, "cancelled"=w1267:bool, "error out"=w1271:errorcluster)  [unwired: 8 in, 1 out]
                n1090 = Not(x=w1267) -> (.not. x?=w1268:bool)
                n1091 = case shown="Vrai" w1268 {
                  tunnel: w1271 -> [w1276 w1279]
                  tunnel: w1270 -> [_ w1278]
                  tunnel: [w1276 w1277] -> w1269
                  frame False {
                  }
                  frame True {
                    n1092 = flat-sequence {
                      tunnel: [w1282] -> w1277
                      tunnel: w1279 -> [w1281]
                      tunnel: w1278 -> [w1280]
                      frame #0 {
                        n1093 = global read "CalibrationState.vi" "CalibrationState"() -> (w1283:T7)
                        n1094 = call "WriteCalibrationFile.vi"("error in (no error)"=w1281, "CalibrationState"=w1283, "Path"=w1280) -> ("error out"=w1282:errorcluster)  [unwired: 8 in]
                      }
                      frame #1 {
                        n1095 = local write "SaveCalibrationFile"(FALSE ("SaveCalibrationFile")) -> ()
                      }
                    }
                  }
                }
              }
            }
          }
          event "btnVidanger": Value Change {
            # "Possibilité de vidanger à tout moment"
            n1096 = event-data() -> ("NewVal"=w1287:bool)  [unwired: 1 in, 5 out]
            n1097 = case shown="Vrai" w1287 {
              tunnel: w1286 -> [w1288 w1290]
              tunnel: [w1288 w1289] -> w1285
              frame False {
              }
              frame True {
                n1098 = stacked-sequence {
                  tunnel: w1290 -> [_ _ _ w1305 _ _]
                  tunnel: [_ _ _ w1305 _ _] -> w1289
                  frame #0 {
                    n1099 = property on="manualModeBtn" class="Bool (strict)"("Val(Sgnl)"=FALSE, "DisabledEnum"=T6."Disabled and Grayed Out" ("Disabled")) -> ()  [unwired: 2 in, 2 out]
                  }
                  frame #1 {
                    n1100 = global write "AppState.vi" "AppState"(u16 3 ("AppState")) -> ()
                  }
                  frame #2 {
                    w1301 = FALSE ("Value (Signaling)")
                    # "Efface/Affiche les contrôles nécessaires"
                    n1101 = global read "LanguagesSettings.vi" "LanguageSettings"() -> (w1297:T9)
                    n1102 = property on="CalibrationResultsVisible" class="Bool (strict)"("Val(Sgnl)"=w1301) -> ()  [unwired: 2 in, 2 out]
                    n1103 = property on="CalibrationButtonsVisible" class="Bool (strict)"("Val(Sgnl)"=w1301) -> ()  [unwired: 2 in, 2 out]
                    n1104 = property on="MeasureIndicatorsVisible" class="Bool (strict)"("Val(Sgnl)"=w1301) -> ()  [unwired: 2 in, 2 out]
                    n1105 = property on="MeasureSetupButtonsVisible" class="Bool (strict)"("Val(Sgnl)"=w1301) -> ()  [unwired: 2 in, 2 out]
                    n1106 = property on="ChangeMenuState" class="Bool (strict)"("Val(Sgnl)"=w1301) -> ()  [unwired: 2 in, 2 out]
                    n1107 = property on="ExportMeasuresButtonsVisible" class="Bool (strict)"("Val(Sgnl)"=w1301) -> ()  [unwired: 2 in, 2 out]
                    n1108 = Unbundle By Name(w1297) -> ("LocalisationFileContent[out]"=w1296:T16)
                    n1109 = local read "LanguagesList"() -> (w1300:i32)
                    n1110 = property on="PurgeState" class="Ch"("Visible"=TRUE) -> ()  [unwired: 2 in, 2 out]
                    n1111 = call "FindLocalizedString.vi"("LangIndex"=w1300, "LocalizationFileContent"=w1296, "WordIndex"=u32 88) -> ("Found"=w1299:bool, "LocalizedString"=w1298:string)  [unwired: 7 in]
                    n1112 = case shown="Vrai" w1299 {
                      tunnel: w1298 -> [_ w1304]
                      tunnel: ["Not found" w1304] -> w1294
                      frame False {
                      }
                      frame True {
                      }
                    }
                    n1113 = property on="PurgeState" class="Ch"("Text.Text"=w1294) -> ()  [unwired: 2 in, 2 out]
                  }
                  frame #3 {
                    # "Effectue la vidange"
                  }
                  frame #4 {
                    # "Affiche le message de réussite, retransitionne vers l'état idle"
                    n1114 = global read "LanguagesSettings.vi" "LanguageSettings"() -> (w1306:T9)
                    n1115 = global write "AppState.vi" "AppState"(u16 0 ("AppState")) -> ()
                    n1116 = property on="manualModeBtn" class="Bool (strict)"("DisabledEnum"=T6."Enabled" ("Disabled")) -> ()  [unwired: 2 in, 2 out]
                    n1117 = Unbundle By Name(w1306) -> ("LocalisationFileContent[out]"=w1309:T16)
                    n1118 = local read "LanguagesList"() -> (w1312:i32)
                    n1119 = call "FindLocalizedString.vi"("LangIndex"=w1312, "LocalizationFileContent"=w1309, "WordIndex"=u32 87) -> ("Found"=w1311:bool, "LocalizedString"=w1310:string)  [unwired: 7 in]
                    n1120 = case shown="Vrai" w1311 {
                      tunnel: w1310 -> [_ w1316]
                      tunnel: ["Not found" w1316] -> w1307
                      frame False {
                      }
                      frame True {
                      }
                    }
                    n1121 = property on="PurgeState" class="Ch"("Text.Text"=w1307) -> ()  [unwired: 2 in, 2 out]
                  }
                  frame #5 {
                    n1122 = property on="ChangeMenuState" class="Bool (strict)"("Val(Sgnl)"=TRUE ("Value (Signaling)")) -> ()  [unwired: 2 in, 2 out]
                  }
                }
              }
            }
          }
          event "Pressure Offset", "Pressure Gain": Value Change {
            n1123 = event-data() -> ()  [unwired: 1 in, 6 out]
            n1124 = local read "Pressure Offset"() -> (w1321:dbl)
            n1125 = local read "Pressure Gain"() -> (w1320:dbl)
            n1126 = call "capt_scaling.vi"("error in"=w1319, "Gain"=w1320, "Offset"=w1321) -> ("error out"=w1318:errorcluster)  [unwired: 8 in]
          }
        }
        n1127 = local read "btnExit"() -> (w352:bool)
        n1128 = case shown="Erreur" w348 {
          tunnel: w348 -> [w353 w355]
          tunnel: [w353 errorcluster {"status"=FALSE, "code"=0, "source"=""} ("error in")] -> w349
          frame No Error {
          }
          frame Error {
            n1129 = local write "error out"(w355) -> ()
          }
        }
      }
      n1130 = while {
        shift-right: [w100] -> _
        shift-left: w99 -> [w102]
        stop <- w103 stop-if-true
        # "Boucle d'acquisition continue"
        n1131 = local read "btnExit"() -> (w103:bool)
        n1132 = call "ContinuousPressureAcquisition.vi"("error in"=w102) -> ("error out"=w101:errorcluster)  [unwired: 10 in]
        n1133 = case shown="Erreur" w101 {
          tunnel: [w104 errorcluster {"status"=FALSE, "code"=0, "source"=""} ("error in")] -> w100
          tunnel: w101 -> [w104 _]
          frame No Error {
          }
          frame Error {
          }
        }
      }
    }
    frame #2 {
      # "Nettoyage avant quittage"
      n1134 = global read "HardwarePresent.vi" "HardwarePresent"() -> (w1322:bool)
      n1135 = case shown="Vrai" w1322 {
        frame False {
          n1136 = Stop() -> ()  [unwired: 1 in]
        }
        frame True {
          n1137 = Quit LabVIEW(quit? (T)=TRUE) -> ()
        }
      }
    }
  }
